vi "UNITEST MAIN v01.vi"() -> ()   [LabVIEW 2025]
uses:
  controls/LAB-IQ UI Data.ctl
  02c5850b-52e8-4ed5-91f8-6f0ad62f4994.vi
  support/Message Queue/Enqueue Message (Single).vi
  <vilib>/Utility/error.llb/Error Cluster From Error Code.vi
  <vilib>/ErrorRing/Error Ring.xnode
  support/Message Queue/LAB-IQ Message Queue.lvlib
  support/User Event - Stop/LAB-IQ User Event - Stop.lvlib
panel:
  in  "Stop Scratch":bool
  in  "Enter Fixed SRR 2":dbl min=0.0 max=0.0 format="%.3f"
  in  "E.Velocity 2":bool=TRUE caption="SRR"
  out "Message":string="Load Entered is out of range!!!"
  in  "Tab Control 3":T1(tab)
  in  "Tab Control 5":enum32{""}(tab)
  in  "Tab Control 14":T2(tab)=enum."Motor Load"
  in  "Ramp MulFac":dbl=2.0
  in  "pulses LoadDiffRamp(2..10)":dbl=9.0
  in  "PulseControlRamp(diff<=3N)":dbl=5.0 min=1.0 max=1000.0 step=1.0 format="%#.1f"
  in  "SetLoadDeadband(%) Load(0-10N)":dbl=0.1 min=0.0001 max=100.0 step=0.0001 format="%#.6f"
  in  "PID gains out delay (microForce)":T3={"proportional gain (Kc)"=300.0, "integral time (Ti, min)"=0.00011, "derivative time (Td, min)"=0.0} {"derivative time (Td, min)" format="%.3f"; "integral time (Ti, min)" min=1e-05 max=100.0 step=1e-06 format="%.6f"; "proportional gain (Kc)" format="%.3f"}
  in  "Ramp":bool
  in  "Gain 2":dbl=0.016
  in  "pulses LoadDiff(2..10)":dbl=10.0
  in  "pulses LoadDiff(11..50)":dbl=40.0
  in  "PulseControl(diff<=3N)":dbl=1.0 min=1.0 max=1000.0 step=1.0 format="%#.1f"
  out "SetLoadDeadband(%)  2":dbl=1.0 min=0.001 max=100.0 step=0.001 format="%#.6f"
  in  "Dummy Run":bool
  out "Vertical load (N)":dbl format="%#.3f"
  in  "AutoTune":bool
  in  "Offset  3":dbl=1.5
  in  "apply load":bool
  in  "Enter ByPass Load":dbl
  in  "reinit 3":bool=TRUE
  in  "output range delay":cluster{"output high":dbl, "output low":dbl}={"output high"=100.0, "output low"=-100.0} {"output low" format="%.2f"; "output high" format="%.2f"}
  in  "PID gains out delay":T3={"proportional gain (Kc)"=30.0, "integral time (Ti, min)"=0.00101, "derivative time (Td, min)"=0.0} {"derivative time (Td, min)" format="%.3f"; "integral time (Ti, min)" min=1e-05 max=100.0 step=0.0001 format="%.4f"; "proportional gain (Kc)" format="%.3f"}
  in  "Bypass Load":bool
  in  "pulsesSent":dbl=200.0
  out "pulses":dbl
  out "actpid":dbl
  out "gFF Rot 7":cluster{dbl, dbl, dbl}(graph)
  in  "pulses LoadDiff(21..1000)":dbl=40.0
  in  "Delay":dbl=1.5 min=0.001 max=5.0 step=0.001 format="%#.6f"
  in  "deadband":dbl=0.2
  in  "Tab Control 26":enum32{"Page 1", "Page 2"}(tab)
  in  "ClearAll":bool
  out "Mz(Nm)":dbl[](array[numeric])
  out "My(Nm)":dbl[](array[numeric])
  out "Mx(Nm)":dbl[](array[numeric])
  in  "Save Dwell":dbl=0.015 caption="Save Dwell (sec)" min=0.0 max=5.0 step=0.001 format="%.3f"
  out "Mx":dbl[](graph)
  out "My":dbl[](graph)
  out "Mz":dbl[](graph)
  out "Fx(N)":dbl[](graph)
  out "Fy(N)":dbl[](graph)
  out "Fz(N)":dbl[](graph)
  in  "ZeroAll":bool
  in  "Acq Delay (ms)":dbl=10.0
  in  "Burst Delay (ms)":dbl=10.0
  out "model":string
  out "SN":i32
  out "FFx(N)":dbl[](array[numeric])
  in  "Sensor IP":string="192.168.1.100"
  in  "Port":i32=8080
  out "FFy(N)":dbl[](array[numeric])
  out "Load(N)":dbl[](array[numeric])
  out "AE":bool
  in  "delete Handle":bool
  in  "Create Handle":bool=TRUE
  out "ft_data":dbl[](array[numeric])=[1.0, 1.0, 1.0, 1.0, 1.0, 1.0]
  out "ft_range":dbl[](array[numeric])=[1.0, 1.0, 1.0, 1.0, 1.0, 1.0]
  in  "stop 6":bool
  out "running_flag":bool
  out "ft_udp_handle":i32
  out "get-data-return":i32
  out "get-range-return":i32
  out "zero-return":i32
  out "filter-return":i32
  out "initial-return":i32
  out "deleteHandle-result":i32
  in  "Tab Control 19":enum32{"Platform COM", "Config ", "DevInfo"}(tab)=enum."Config "
  in  "SAMPLES":dbl=100.0
  in  "Re-initilaize":bool
  in  "Filter ON/OFF":bool=TRUE
  in  "TracHomeSurgeOffsetCounts 10MM":dbl=505100.0
  in  "TracHomeSwayOffsetCounts 10MM":dbl=1432.0
  in  "Acoustic Emission:":dbl=1.0 min=0.0001 max=200.0 step=0.0001 format="%.4f"
  in  "Apply Filter (FF)":bool
  in  "Filter% 2":dbl=50.0 min=50.0 max=100.0 step=0.1 format="%.1f"
  in  "Apply Filter (Load)":bool=TRUE
  in  "Filter%":dbl=80.0 min=50.0 max=100.0 step=0.1 format="%.1f"
  in  "Sway distance (mm)":dbl=245.0
  in  "Surge distance (mm)":dbl=370.0
  in  "DataSavingLoopDelay(ms)":dbl=15.0
  in  "SAVE  2":bool
  in  "Enter Distance":bool caption="Enter Counts"
  in  "Sway Counts:":dbl=100.0 min=0.0 max=100000000.0 step=1.0 format="%.2f"
  in  "Distance (mm): 3":dbl=100.0 caption="Distance (mm):" min=0.0 max=1500.0 step=0.001 format="%.5f"
  in  "Surge Counts:":dbl=100.0 min=0.0 max=100000000.0 step=1.0 format="%.1f"
  in  "Distance (mm): 2":dbl=100.0 caption="Distance (mm):" min=0.0 max=1500.0 step=0.0001 format="%.3f"
  in  "Distance (mm):":dbl=100.0 min=0.0 max=1500.0 step=0.001 format="%.5f"
  in  "Heave Counts:":dbl=100.0 min=0.0 max=100000000.0 step=1.0
  in  "LRMHomeSurgeOffsetCounts":dbl=307197.0
  in  "LRMHomeSwayOffsetCounts":dbl=26880.0
  in  "TracHomeSurgeOffsetCounts 20MM":dbl=505100.0
  in  "TracHomeSwayOffsetCounts 20MM":dbl=1432.0
  in  "RotHomeSwayOffsetCounts":dbl=14656.0
  in  "RotHomeSurgeOffsetCounts":dbl=311465.0
  in  "Heave distance":dbl=340.0
  out "Zmm":dbl=1600.0
  out "Heave Pulses/mm":dbl=1600.0
  out "Surge Pulses/mm":dbl=1600.0
  out "Sway Pulses/mm":dbl=320.0
  in  "Heave Pitch":dbl=4.0
  in  "Surge Pitch":dbl=3.0
  in  "Sway Pitch":dbl=2.0
  in  "Heave PPR":dbl=6400.0
  in  "Surge PPR":dbl=6400.0
  in  "Sway PPR":dbl=6400.0
  in  "GUI":T4(tab)
  in  "Platform Settings":bool caption="Password"
  in  "Configure":bool caption="Password"
  in  "Home":bool caption="Password"
  in  "EXIT":bool
  in  "Analysis":bool caption="Password"
  in  "service 2":bool caption="Password"
  in  "MainPage":T5(tab)=enum."HOME"
  in  "Select Load Head":bool
  in  "Notes :":string
  in  "FILE":string
  in  "Sample ID :":string
  in  "Operator ID :":string
  in  "Operator Name :":string
  in  "Auto":bool caption="Power Status"
  out "mm/s  Surge":dbl=7.0 caption="Jog" min=0.001 max=50.0 step=0.0001 format="%.2f"
  in  "Update Surge Speed":bool
  out "Drive Error":string
  in  "Disable Axis Jog Soft Limits":bool
  out "mm/s  Sway":dbl=7.0 caption="Jog" min=0.001 max=50.0 step=0.0001 format="%.2f"
  out "Sway and Surge COM Status":bool=TRUE caption="Load COM Status"
  out "Heave COM Status":bool=TRUE caption="Load COM Status"
  in  "Enable Platform":bool
  in  "Surge Forward Main":bool
  in  "Surge Backward Main":bool
  in  "Sway Right Main":bool
  in  "Sway Left Main":bool
  in  "Heave Down Main":bool
  in  "Heave Up main":bool
  in  "Update Sway Speed":bool
  in  "Update Heave Speed":bool
  out "mm/s Heave":dbl=7.0 caption="Jog" min=0.001 max=30.0 step=0.0001 format="%.2f"
  in  "mm/sec":dbl=1.0 caption="Jog" min=0.001 max=50.0 step=0.001 format="%.2f"
  in  "mm":dbl=0.001 caption="Jog" min=0.001 max=200.0 step=0.0001 format="%#.3f"
  in  "Surface Analysis":bool
  in  "Imaging":bool
  in  "Image Analysis":bool
  in  "Post Analysis":bool
  in  "SSP 0.75":bool
  in  "SSP 0.5":bool
  in  "SSP 0.3":bool
  in  "Warning":enum32{"Page 2"}(tab)
  in  "gui GIF":enum32{"Check", "Deca", "kilo", "Micro"}(tab)
  out "Communication is established":bool=TRUE caption="Load COM Status"
  in  "Reference Sample":u16(ring) items=["None", "Brass", "Aluminium", "Mild Steel"]
  out "Load Cell Communication Slide":u8(slide)=1 min=1 max=10 step=1 scale=0.0..10.0
  in  "com 3":bool
  out "com":bool
  out "DecaForce COM Status":bool caption="Load COM Status"
  in  "Loading Mode":u16(ring) items=["Constant", "Ramp", "Steps", "Indentation"]
  in  "Enter the CoF Trip":dbl=1.0
  in  "Enter the Friction Force Trip":dbl=520.0 min=500.0 max=500.0 step=1.0 format="%#.1f"
  in  "Enter the Normal load Trip":dbl=520.0 min=500.0 max=500.0 step=0.001 format="%.3f"
  in  "KiloForce":bool
  in  "DecaForce":bool
  in  "MicroForce":bool
  in  "LHBack":bool
  in  "LHNext":bool
  in  "Load Selection":T6(tab)
  in  "Enter the Load  (N)":dbl=2.0 min=2.0 max=50.0 step=0.1 format="%#.4f"
  in  "Enter the Final Load (N)":dbl=1.0 min=0.0 max=500.0 step=1.0 format="%#.0f"
  in  "Update":bool
  in  "Enter the Loading Rate (N/min)":dbl=60.0 min=60.0 max=1200.0 step=0.1 format="%.2f"
  out "Warning 2":bool
  in  "Stribeck Table  For loading":string[][](table)=[["", "", ""], ["", "", ""], ["", "", ""], ["", "", ""]]
  in  "Stribeck table":bool
  in  "seq":bool=TRUE
  in  "Clear 3":bool
  in  "Indentation":string[][](table)=[["Detection", "5", "2"], ["Unload", "0", "5"], ["Load", "10", "2"], ["Unload", "0", "5"], ["Detection", "5", "2"], ["Unload", "0", "5"]]
  in  "Multipoint":bool caption="Singlepoint"
  in  "AppLoad 4":bool
  in  "zNL":bool
  out "NL disp":dbl caption="Normal Load ( N )" min=-2000.0 max=2000.0 step=0.0001 format="%.1f"
  in  "Traction":bool
  in  "Surge Forward MM":bool
  in  "Surge Backward MM":bool
  in  "M3 Image":enum32{"Page 1", "Page 2"}(tab)
  in  "String 39":string="Jog heave to bring the upper sample closer to the lower sample within 1mm."
  in  "Sway Left MM":bool
  in  "Sway Right MM":bool
  in  "Disable Axis Jog Soft Limits":bool
  in  "mm":dbl=0.001 caption="Jog" min=0.001 max=5.0 step=0.0001 format="%#.3f"
  in  "Heave Down MM":bool
  in  "Heave Up MM":bool
  in  "Wear Track Diameter (mm)":dbl=5.0 caption="Wear Track Diameter (mm):" min=1.0 max=30.0 step=1.0 format="%.2f"
  in  "Set WTD":bool
  in  "HomeScratch":bool
  in  "HomeRot":bool
  in  "PlaceModule":bool
  in  "Motion Mode:":u16(ring) items=["Uniform Rotation", "Angular Oscillation", "Stribeck ", "Steps"]
  in  "LR Sway":bool
  in  "Rot Hor":bool
  in  "Rot Ver":bool
  in  "Scratch":bool
  in  "LR Cam":bool
  in  "MMBack":bool
  in  "MMNext":bool
  in  "Rotary Module Selection":T7(tab)
  in  "SPEED SELECTION :":enum32{"Speed in RPM", "Speed in m/sec"}(radio)=enum."Speed in m/sec"
  in  "TEST SELECTION":enum32{"Time", "Cycle"}(radio)
  in  "Enter the Speed(mm/sec)":dbl=1.0 min=0.1 max=10.0 step=0.1 format="%.1f"
  in  "Enter the Speed(RPM)":dbl=45.0 min=5.0 max=300.0 step=1.0
  in  "Enter the Frequency (Hz)":dbl=1.0 min=0.1 max=10.0 step=0.1 format="%.1f"
  in  "Enter the Angle (Deg)":dbl=45.0 min=5.0 max=300.0 step=1.0
  in  "Angular Oscillation Set":bool
  in  "Rotary Tab":enum32{"Page 1", "Page 2"}(tab)
  out "e.v/ssr 2":enum32{"E.V", "SSR"}(tab)
  in  "Enter the Final E.Velocity (m/s) 2":dbl=1.0 min=0.001 max=4.0 step=0.001 format="%.3f"
  in  "Enter initial E.Velocity (m/s) 2":dbl=2.0 min=0.001 max=4.0 step=0.001 format="%.3f"
  in  "Enter Fixed E.Velocity 2":dbl=1.0 min=0.001 max=2.0 step=0.001 format="%.3f"
  in  "Enter Final SRR 2":dbl=1.0 min=0.001 max=1.0 step=0.001 format="%.2f"
  in  "Enter initial SRR 2":dbl=1.0 min=0.001 max=1.0 step=0.001 format="%.2f"
  out "Final Speed (RPM) 3":dbl=1.0 min=0.1 max=3000.0 step=0.1 format="%.1f"
  out "Initial Speed (RPM) 2":dbl=100.0 min=0.1 max=3000.0 step=0.1 format="%.1f"
  in  "Enter the Final Velocity (m/s) 3":dbl=1.0 min=0.001 max=2.0 step=0.001 format="%.3f"
  in  "Enter initial Velocity (m/s)  3":dbl=2.0 min=0.001 max=2.0 step=0.001 format="%.3f"
  out "Ramp Up 2":bool caption="Ramp Down"
  in  "File Path :  2":path
  in  "Import 2":bool
  in  "Save 2":bool
  in  "SPEED SELECTION : rotary":enum32{"Speed in Rpm", "Speed in m/sec"}(radio)=enum."Speed in m/sec"
  in  "calculate rotary":bool
  in  "String 45":string="File Path Location : C:-->LAB-IQ 150 --> User Defined\n                                       Protocol-->File.txt"
  in  "Step Speed":enum32{"Step Speed", "Step (load-Speed)"}(tab)
  in  "StepTable For Speed":string[][](table)=[["", "", ""], ["", "", ""], ["", "", ""], ["", "", ""]]
  in  "StepTable For Load-Speed":string[][](table)=[["", "", ""], ["", "", ""], ["", "", ""], ["", "", ""]]
  in  "StepTable For Speed 3":string[][](table)=[["", "", ""], ["", "", ""], ["", "", ""], ["", "", ""]]
  in  "Motion Direction:  3":u16(ring) items=["Clockwise", "Counter Clockwise"]
  out "Humidity  Status  3":bool caption="Communication Status"
  out "Low Temp  Status  2":bool caption="Communication Status"
  out "TK4 status 2":bool caption="Communication Status"
  in  "String 40":string="Before selecting Acoustic make sure the sensor output pin is connected to A4."
  in  "Stage Temperature":dbl[](array[numeric])=[150.0, 230.0, 300.0, 350.0, 400.0, 450.0, 500.0]
  in  "Sample Temperature":dbl[](array[numeric])=[100.0, 150.0, 200.0, 250.0, 300.0, 350.0, 400.0]
  in  "Humidity (Amb)":bool
  in  "Clear List":bool
  out "Sensors Picked":string
  in  "Add to list":bool
  in  "Wear":bool
  in  "Vibration":bool
  in  "Humidity (Chamber)":bool
  in  "Temperature (Chamber)":bool
  in  "ECR":bool
  in  "Temperature (Amb)":bool
  in  "Microphone":bool
  in  "Acoustic Emission 3":bool
  in  "SNext":bool
  in  "APBack":bool
  in  "Enter the Temperature (°C):":dbl
  in  "Enter the Stage \nTemperature (°C):":dbl=20.0 min=20.0 max=150.0 step=1.0 format="%#.0f"
  in  "Enter the Humidity (%Rh):":dbl=30.0 min=30.0 max=85.0 step=1.0
  in  "Low Temp":bool
  in  "High Temp":bool
  in  "Humidity":bool
  in  "Main Screen Tab":T8(tab)
  in  "AppLoadSeq scratch":bool
  in  "ClrLog":bool
  out "Trip Log":string
  in  "STOP":bool
  in  "Start Test":bool
  out "Test status":bool caption="Test Status"
  out "AR Led":bool caption="AR"
  out "Data":bool=TRUE
  out "Health":bool=TRUE
  out "Sway COM Status":bool=TRUE caption="Load COM Status"
  out "Heave COM Status":bool=TRUE caption="Load COM Status"
  in  "Grp Tab":enum32{"Rot/LRM", "FBT"}(tab)
  in  "Sub Graph":T9(tab)
  in  "Speed Reset Graph":bool
  in  "Speed Tab":enum32{" Rotary Disc", "MTM Ball", "MTM Disc"}(tab)
  out "speed mm/sec":dbl(graph)=0.13298760003255525
  out "MTM BALL SPEED":dbl(graph)=0.13298760003255525
  out "MTM DISC  SPEED":dbl(graph)=0.13298760003255525
  in  "Temperature Reset":bool
  out "Temperature (deg c)":dbl(graph)=0.13298760003255525
  in  "ECR RESET":bool
  out "ECR":dbl(graph)=0.13298760003255525
  out "Acoustic Emission (mV)":dbl min=0.0 max=5000.0 step=0.1
  in  "Aqucostic Reset Graph":bool
  out "gACQUOS":dbl(graph)=0.13298760003255525
  in  "Humidity Reset Graph":bool
  out "HumrGp":dbl(graph)=0.13298760003255525
  out "SD (mm)":dbl caption="Sliding Distance ( mm )" min=-200.0 max=200.0 step=0.1 format="%.4f"
  in  "Siliding distance Reset Graph":bool
  out "SDGp":dbl(graph)=0.13298760003255525
  out "Hymidity":bool
  in  "Humidity Disable trip":bool=TRUE
  in  "CoF Trip  2":dbl=540.0 min=100.0 max=540.0 step=1.0
  out "Depth Trip":dbl=600.0
  in  "Depth Trip":bool=TRUE
  out "Weart Deapth":bool
  in  "Depth Reset Graph":bool
  out "Weart":bool
  in  "Depthz":bool
  out "Depth (µm)":dbl min=-200.0 max=200.0 step=0.1 format="%.1f"
  out "WearGp":dbl(graph)=0.13298760003255525
  out "NL Trip 2":dbl=600.0
  out "Load pid":bool
  in  "Load Disable Trip":bool=TRUE
  in  "Load Reset Graph":bool
  out "NL Display 4":dbl caption="Normal Load ( N )" min=-2000.0 max=2000.0 step=0.0001 format="%.1f"
  out "Main Chart 3":cluster{dbl, "NL disp":dbl, dbl}(graph)
  in  "FF Tab":T10(tab)
  in  "COF Reset Graph":bool
  in  "COF Disable Trip":bool=TRUE
  out "COF TRIP":dbl=600.0
  out "COF MAIN CHART":cluster{dbl, "NL disp":dbl, dbl}(graph)
  out "Friction Force (N)":dbl min=-2000.0 max=2000.0 step=0.0001 format="%.1f"
  in  "FF Reset Graph":bool
  in  "FF Disable Trip":bool=TRUE
  out "FF TRIP":dbl=600.0
  out "FF MAIN CHART":cluster{dbl, "NL disp":dbl, dbl}(graph)
  in  "BACK":bool
  out "Ambient \nTemperature":dbl min=0.0 max=5000.0 step=0.1 format="%.1f"
  out "Ambient\n Humidity":dbl min=0.0 max=5000.0 step=0.1 format="%.2f"
  out "NL disp 2":dbl caption="Normal Load ( N )" min=-2000.0 max=2000.0 step=0.0001 format="%.1f"
  out "Set Humidity":dbl caption="Set Humidity  (% Rh)" min=-2000.0 max=2000.0 step=1.0 format="%.1f"
  out "humidity disp":dbl caption="Humidity (% Rh)" min=-2000.0 max=2000.0 step=1.0 format="%.1f"
  in  "Humidity On":bool
  in  "zNL 2":bool
  out "NLt":bool
  in  "Load En":bool
  out "Freq (Hz)":dbl min=0.0 max=5000.0 step=0.1 format="%.4f"
  out "HumCOMStatus":bool caption="Communication Status"
  out "Load Communication":bool
  in  "Temp Tabs":enum32{"Low Temp", "High Temp"}(tab)
  out "Controller  Status":bool
  out "ChamberTemp":dbl format="%#.1f"
  in  "SetTmp":dbl=-190.0 caption="Set Temperature (Deg C)" min=-190.0 max=100.0 step=1.0 format="%.1f"
  in  "Cooling":bool
  in  "Heater":bool
  out "TK4 status":bool caption="Controller  Status"
  out "ChamberTemp":dbl format="%#.1f"
  in  "SetTmp":dbl caption="Set Temperature (Deg C)" min=0.0 max=1000.0 step=1.0 format="%.1f"
  in  "Set Load (N)":dbl=100.0 min=0.01 max=1500.0 step=0.01 format="%.1f"
  in  "Time Tab":enum32{"cycles", "duration"}(tab)
  out "Test Duration 4":dbl=600.0 caption="Test Duration\n(HH:MM:SS)" min=0.0083 max=180000.0 step=0.0001 format="%<%H:%M:%S>t"
  out "TEST CYCLE":dbl min=0.0 max=5000.0 step=0.01 format="%.2f"
  in  "TOTAL CYCLES":dbl min=0.0 max=5000.0 step=0.1 format="%.4f"
  out "Time ( HH:MM:SS ) 2":dbl min=0.0 max=144000.0 step=1.0 format="%<%H:%M:%S>t"
  in  "Test Duration":dbl=600.0 caption="Test Duration\n(HH:MM:SS)" min=0.0083 max=180000.0 step=0.0001 format="%<%H:%M:%S>t"
  in  "Main Speed Tab":enum32{"ROTARY", "TRACTION"}(tab)
  in  "SPEED TAB":enum32{"RPM", "m/sec"}(tab)
  out "Speed (RPM)":dbl min=0.0 max=5000.0 step=0.1 format="%.1f"
  out "Set Speed":dbl caption="Set Speed (RPM)" min=0.0 max=1500.0 step=0.1 format="%.1f"
  out "Speed (m/sec)":dbl min=0.0 max=5000.0 step=0.001 format="%.4f"
  out "Set Speed (m/sec)":dbl min=0.0 max=1500.0 step=0.001 format="%.4f"
  in  "MTM MOTOR DISPLAY":enum32{"MTM RPM", "MTM m/sec"}(tab)
  out "Disc Speed (RPM)":dbl min=0.0 max=1500.0 step=0.1 format="%.1f"
  out "Ball Speed (RPM)":dbl min=0.0 max=1500.0 step=0.1 format="%.1f"
  out "Disc Speed (m/sec)":dbl min=0.0 max=1500.0 step=0.1 format="%.1f"
  out "Ball Speed (m/sec)":dbl min=0.0 max=1500.0 step=0.1 format="%.1f"
  in  "Angle and Frequency":enum32{"angular", "lrm"}(tab)
  out "Angle (Deg)":dbl min=0.0 max=5000.0 step=0.01 format="%.2f"
  out "Stroke (mm)":dbl min=0.0 max=5000.0 step=0.01 format="%.2f"
  in  "Analysis Home":bool
  in  "Password":string
  in  "Home Service":bool
  in  "Advanced Setting":bool
  in  "About Tab":enum32{"Primary"}(tab)
  in  "ECR Port:":refnum<visa-resource-name>="COM10"
  in  "Ramp Port:":refnum<visa-resource-name>="COM10"
  in  "Installation/Replacement completed":bool
  in  "Loahead":bool
  in  "Heave and Surge COM Port:":refnum<visa-resource-name>="COM9"
  in  "Sway COM Port:":refnum<visa-resource-name>="COM10"
  in  "Temp Modbus:":refnum<visa-resource-name>="COM14"
  in  "Humidity Port:":refnum<visa-resource-name>="COM10"
  in  "Edit Gain Constants":bool
  in  "Save Gain Constants":bool
  in  "Service About":bool
  # "load Aquisition off"
  # "load Aquisition On"
  # "Configuration"
  # "Limits for Heave Surge and Sway"
  # "Modules Offset Parameters"
  # "Counts-Distance Calculator"
  # "File Name :"
  # "Ensure the traction module is aligned\n horizontally with the stage before ENABLE."
  # "SET JOG SPEED"
  # "JOG MODE"
  # "Module Selection"
  # "Positioning Control"
  # "Connect the controller\ncable to M3"
  # "Environment"
  # "Sensors"
  # "Data Points"
  # "Data Points"
  # "Data Points"
  # "Data Points"
  # "ohms"
  # "Data Points"
  # "Data Points"
  # "Data Points"
  # "LAB-IQ 150 / UNITEST / WO2456 / UT150  v05 / AUGUST 2025"
  # "NOTE: This operation needs to be done only when the machine is ON."
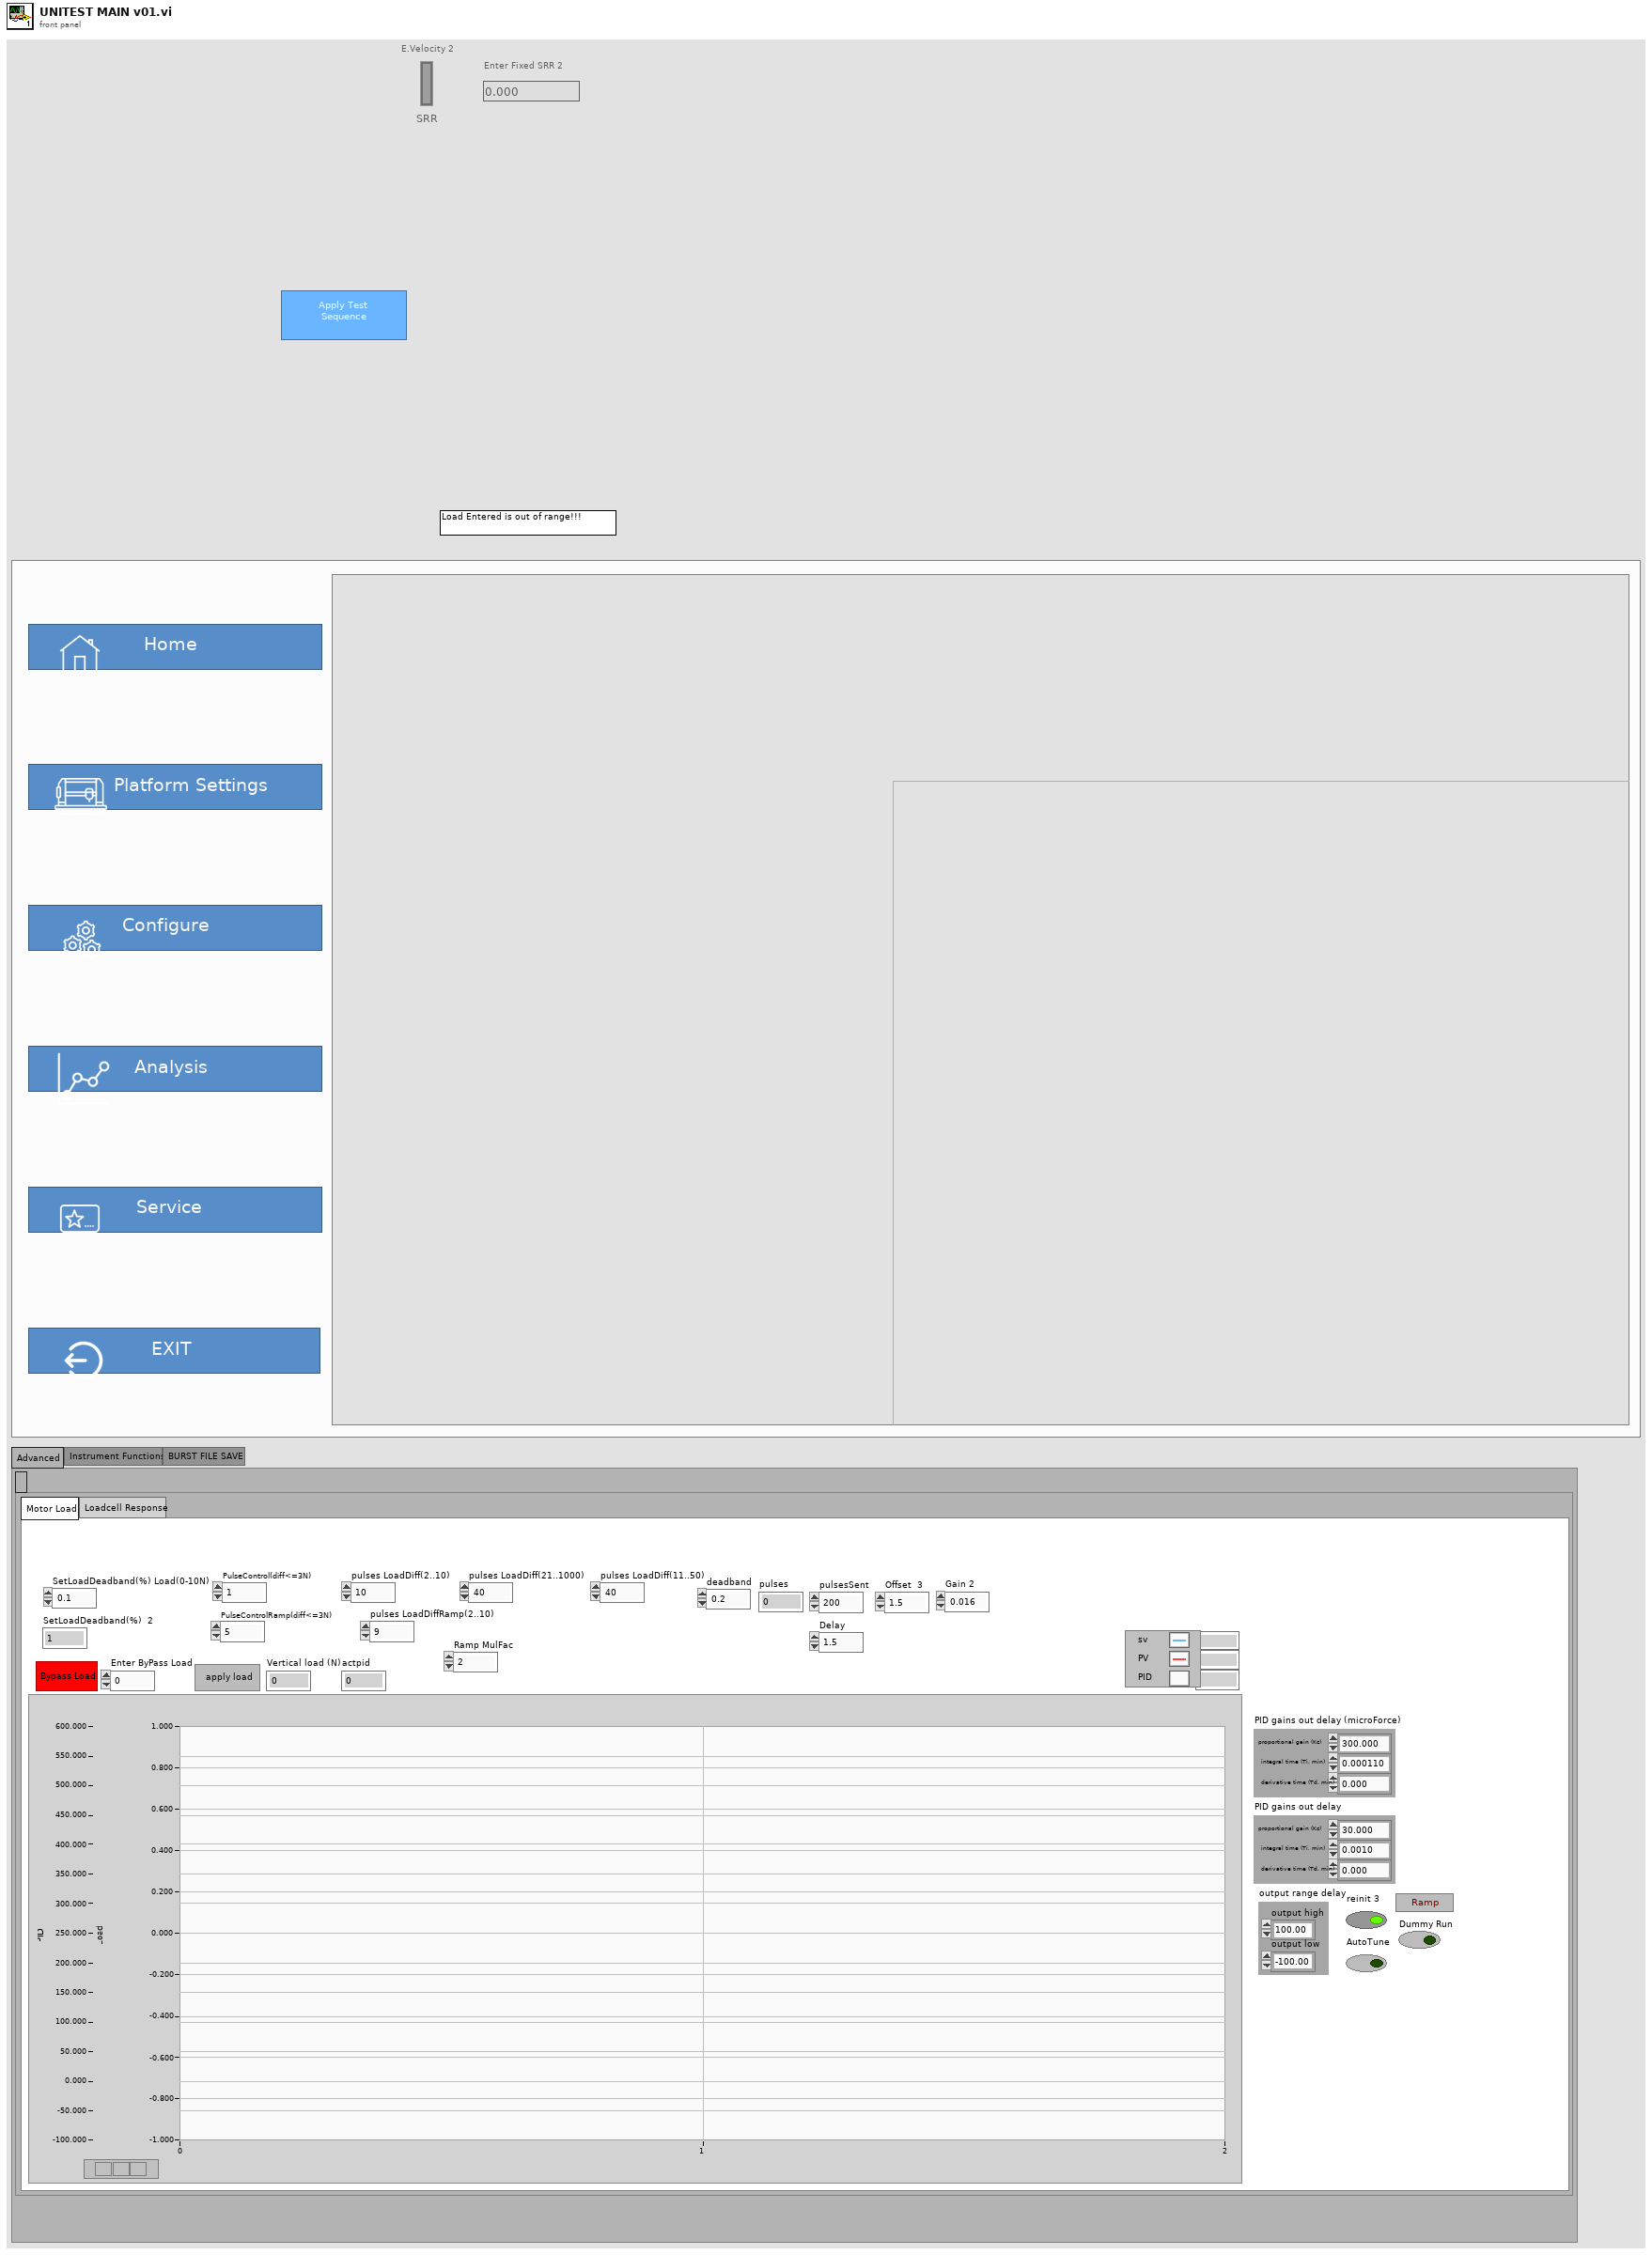
[diagram p1: front panel]
types:
  T1 = enum32{"Advanced", "Motor", "Depth_graph", "UIO Communicator", "Add to list parametrs", "Instrument Functions", "BURST FILE SAVE"}
  T2 = enum32{"LRM heating", "FBT_Heating", "Motor Load", "Loadcell Response", "Voice Load", "Step loading and speed ", "Depth"}
  T3 = cluster{"proportional gain (Kc)":dbl, "integral time (Ti, min)":dbl, "derivative time (Td, min)":dbl}
  T4 = enum32{"Setup", "Load Head", "Motion Module", "Environment", "Begin"}
  T5 = enum32{"Details", "PlatformSetting", "Analysis", "HOME"}
  T6 = enum32{"Constant", "Ramp", "Step", "Indentation"}
  T7 = enum32{"Uniform Rotation", "Angular Oscillation", "Speed Ramp", "Speed Step"}
  T8 = enum32{"  Acquire  ", "Compare Files Rot", "About", "Service"}
  T9 = enum32{"Speed", "Temperature", "ECR", "Acoustic Emission", "Humidity", "Sliding Distance"}
  T10 = enum32{"Coefficient of Friction ", "Friction Force (N)"}
  T11 = typedef "LAB-IQ UI Data.ctl" = cluster{"Main Home Screen":cluster{"GUI":refnum<vi>, "Platform Settings":refnum<vi>, "Configure":refnum<vi>, "Home":refnum<vi>, "EXIT":refnum<vi>, "service 2":refnum<vi>, "MainPage":refnum<vi>, "Analysis":refnum<vi>}, "Platform Settings":cluster{"mm/s  Surge":refnum<vi>, "Update Surge Speed":refnum<vi>, "Drive Error":refnum<vi>, "Disable Axis Jog Soft Limits":refnum<vi>, "mm/s  Sway":refnum<vi>, "Sway and Surge COM Status":refnum<vi>, "Heave COM Status":refnum<vi>, "Enable Platform":refnum<vi>, "Surge Forward Main":refnum<vi>, "Sway Right Main":refnum<vi>, "Sway Left Main":refnum<vi>, "Heave Down Main":refnum<vi>, "Heave Up main":refnum<vi>, "Update Sway Speed":refnum<vi>, "Update Heave Speed":refnum<vi>, "mm/s Heave":refnum<vi>, "mm/sec":refnum<vi>, "mm":refnum<vi>, "Surge Backward Main":refnum<vi>}, "Analysis Screen":cluster{"Analysis Home":refnum<vi>, "Surface Analysis":refnum<vi>, "Imaging":refnum<vi>, "Image Analysis":refnum<vi>, "Post Analysis":refnum<vi>}, "Config Screen":cluster{"Select Load Head":refnum<vi>, "Notes :":refnum<vi>, "FILE":refnum<vi>, "Sample ID :":refnum<vi>, "Operator ID :":refnum<vi>, "Operator Name :":refnum<vi>, "Auto":refnum<vi>}, "Motion Module":cluster{"zNL":refnum<vi>, "NL disp":refnum<vi>, "Rotary Tab":refnum<vi>, "Motion Direction:  3":refnum<vi>, "E.Velocity 2":refnum<vi>, "e.v/ssr 2":refnum<vi>, "Enter Fixed E.Velocity 2":refnum<vi>, "Enter Final SRR 2":refnum<vi>, "Enter initial SRR 2":refnum<vi>, "Enter Fixed SRR 2":refnum<vi>, "Enter the Final E.Velocity (m/s) 2":refnum<vi>, "Enter initial E.Velocity (m/s) 2":refnum<vi>, "Final Speed (RPM) 3":refnum<vi>, "Initial Speed (RPM) 2":refnum<vi>, "Enter the Final Velocity (m/s) 3":refnum<vi>, "Enter initial Velocity (m/s)  3":refnum<vi>, "Ramp Up 2":refnum<vi>, "TEST SELECTION":refnum<vi>, "SPEED SELECTION : ":refnum<vi>, "Angular Oscillation Set":refnum<vi>, "Traction":refnum<vi>, "Step Speed":refnum<vi>, "StepTable For Load-Speed":refnum<vi>, "StepTable For Speed":refnum<vi>, "Surge Forward MM":refnum<vi>, "Surge Backward MM":refnum<vi>, "M3 Image":refnum<vi>, "String 39":refnum<vi>, "Sway Left MM":refnum<vi>, "Sway Right MM":refnum<vi>, "Disable Axis Jog Soft Limits":refnum<vi>, "mm":refnum<vi>, "Heave Down MM":refnum<vi>, "Heave Up MM":refnum<vi>, "Wear Track Diameter (mm)":refnum<vi>, "Set WTD":refnum<vi>, "HomeScratch":refnum<vi>, "HomeRot":refnum<vi>, "PlaceModule":refnum<vi>, "Enter the Angle (Deg)":refnum<vi>, "Enter the Frequency (Hz)":refnum<vi>, "Motion Mode:":refnum<vi>, "LR Sway":refnum<vi>, "Rot Hor":refnum<vi>, "Scratch":refnum<vi>, "LR Cam":refnum<vi>, "MMBack":refnum<vi>, "MMNext":refnum<vi>, "Rot Ver":refnum<vi>, "Rotary Module Selection":refnum<vi>, "calculate rotary":refnum<vi>, "SPEED SELECTION : rotary":refnum<vi>, "Import 2":refnum<vi>, "Save 2":refnum<vi>, "File Path :  2":refnum<vi>, "String 45":refnum<vi>, "StepTable For Speed 3":refnum<vi>, "Enter the Speed(mm/sec)":refnum<vi>, "Enter the Speed(RPM)":refnum<vi>}, "Environmental control":cluster{"Humidity  Status  3":refnum<vi>, "Low Temp  Status  2":refnum<vi>, "TK4 status 2":refnum<vi>, "Stage Temperature":refnum<vi>, "Sample Temperature":refnum<vi>, "Humidity (Amb)":refnum<vi>, "Clear List":refnum<vi>, "Add to list":refnum<vi>, "Wear":refnum<vi>, "Vibration":refnum<vi>, "Humidity (Chamber)":refnum<vi>, "Temperature (Chamber)":refnum<vi>, "ECR ":refnum<vi>, "Temperature (Amb)":refnum<vi>, "Microphone":refnum<vi>, "Acoustic Emission 3":refnum<vi>, "SNext":refnum<vi>, "APBack":refnum<vi>, "Enter the Temperature (°C):":refnum<vi>, "Enter the Stage \nTemperature (°C):":refnum<vi>, "Enter the Humidity (%Rh):":refnum<vi>, "Low Temp":refnum<vi>, "High Temp":refnum<vi>, "Humidity":refnum<vi>, "Sensors Picked":refnum<vi>}, "About Screen":cluster{"Password":refnum<vi>, "Home Service":refnum<vi>, "Advanced Setting":refnum<vi>, "About Tab":refnum<vi>, "ECR Port:":refnum<vi>, "Ramp Port:":refnum<vi>, "Installation/Replacement completed":refnum<vi>, "Loahead":refnum<vi>, "Heave and Surge COM Port:":refnum<vi>, "Sway COM Port:":refnum<vi>, "Temp Modbus:":refnum<vi>, "Humidity Port:":refnum<vi>, "Edit Gain Constants":refnum<vi>, "Save Gain Constants":refnum<vi>}, "Main Screen":cluster{"Main Screen Tab":refnum<vi>, "Angle and Frequency":refnum<vi>, "Stroke (mm)":refnum<vi>, "Angle (Deg)":refnum<vi>, "Main Speed Tab":refnum<vi>, "MTM MOTOR DISPLAY":refnum<vi>, "Disc Speed (m/sec)":refnum<vi>, "Ball Speed (m/sec)":refnum<vi>, "Disc Speed (RPM)":refnum<vi>, "Ball Speed (RPM)":refnum<vi>, "SPEED TAB":refnum<vi>, "Speed (m/sec)":refnum<vi>, "Set Speed (m/sec)":refnum<vi>, "Speed (RPM)":refnum<vi>, "Set Speed":refnum<vi>, "Time Tab":refnum<vi>, "Time ( HH:MM:SS ) 2":refnum<vi>, "Test Duration":refnum<vi>, "Test Duration 4":refnum<vi>, "TEST CYCLE":refnum<vi>, "TOTAL CYCLES":refnum<vi>, "Set Load (N)":refnum<vi>, "Temp Tabs":refnum<vi>, "Heater":refnum<vi>, "TK4 status":refnum<vi>, "ChamberTemp":refnum<vi>, "SetTmp":refnum<vi>, "Controller  Status":refnum<vi>, "ChamberTemp 2":refnum<vi>, "SetTmp 2":refnum<vi>, "Controller  Status 2":refnum<vi>, "ChamberTemp 3":refnum<vi>, "SetTmp 3":refnum<vi>, "Cooling":refnum<vi>, "Load Communication":refnum<vi>, "Ambient \nTemperature":refnum<vi>, "HumCOMStatus":refnum<vi>, "Ambient\n Humidity":refnum<vi>, "Freq (Hz)":refnum<vi>, "Load En":refnum<vi>, "NLt":refnum<vi>, "zNL 2":refnum<vi>, "Humidity On":refnum<vi>, "humidity disp":refnum<vi>, "Set Humidity":refnum<vi>, "NL disp 2":refnum<vi>, "Humidity On 2":refnum<vi>, "humidity disp 2":refnum<vi>, "Set Humidity 2":refnum<vi>, "NL disp 3":refnum<vi>, "AppLoadSeq scratch":refnum<vi>, "Stop Scratch":refnum<vi>, "ClrLog":refnum<vi>, "Trip Log":refnum<vi>, "STOP":refnum<vi>, "Start Test":refnum<vi>, "Test status":refnum<vi>, "AR Led":refnum<vi>, "Data":refnum<vi>, "Health":refnum<vi>, "Sway COM Status":refnum<vi>, "Heave COM Status":refnum<vi>, "Grp Tab":refnum<vi>, "Sub Graph":refnum<vi>, "SD (mm)":refnum<vi>, "Siliding distance Reset Graph":refnum<vi>, "SDGp":refnum<vi>, "Humidity Reset Graph":refnum<vi>, "HumrGp":refnum<vi>, "Acoustic Emission (mV)":refnum<vi>, "Aqucostic Reset Graph":refnum<vi>, "gACQUOS":refnum<vi>, "ECR RESET":refnum<vi>, "ECR":refnum<vi>, "Temperature Reset":refnum<vi>, "Acoustic Emission (mV) 2":refnum<vi>, "Aqucostic Reset Graph 2":refnum<vi>, "gACQUOS 2":refnum<vi>, "ECR RESET 2":refnum<vi>, "ECR 2":refnum<vi>, "Temperature Reset 2":refnum<vi>, "Temperature (deg c)":refnum<vi>, "Speed Reset Graph":refnum<vi>, "Speed Tab":refnum<vi>, "MTM DISC  SPEED":refnum<vi>, "MTM BALL SPEED":refnum<vi>, "speed mm/sec":refnum<vi>, "Hymidity":refnum<vi>, "Humidity Disable trip":refnum<vi>, "CoF Trip  2":refnum<vi>, "Depth Trip":refnum<vi>, "Weart Deapth":refnum<vi>, "Depth Reset Graph":refnum<vi>, "Weart":refnum<vi>, "Depthz":refnum<vi>, "Depth (µm)":refnum<vi>, "WearGp":refnum<vi>, "NL Trip 2":refnum<vi>, "Load pid":refnum<vi>, "Load Disable Trip":refnum<vi>, "Load Reset Graph":refnum<vi>, "NL Display 4":refnum<vi>, "Main Chart 3":refnum<vi>, "BACK":refnum<vi>, "Depth Trip 2":refnum<vi>}, "Loading":cluster{"Indentation":refnum<vi>, "Reference Sample":refnum<vi>, "Load Cell Communication Slide":refnum<vi>, "com 3":refnum<vi>, "com":refnum<vi>, "DecaForce COM Status":refnum<vi>, "Update":refnum<vi>, "Clear 3":refnum<vi>, "seq":refnum<vi>, "Stribeck table":refnum<vi>, "Stribeck Table  For loading":refnum<vi>, "Loading Mode":refnum<vi>, "Enter the Final Load (N)":refnum<vi>, "Enter the CoF Trip":refnum<vi>, "Enter the Friction Force Trip":refnum<vi>, "Enter the Normal load Trip":refnum<vi>, "Enter the Load  (N)":refnum<vi>, "KiloForce":refnum<vi>, "DecaForce ":refnum<vi>, "MicroForce":refnum<vi>, "LHBack":refnum<vi>, "LHNext":refnum<vi>, "Enter the Loading Rate (N/min)":refnum<vi>, "Message":refnum<vi>, "Warning 2":refnum<vi>, "SSP 0.75":refnum<vi>, "SSP 0.5":refnum<vi>, "SSP 0.3":refnum<vi>, "Warning":refnum<vi>, "gui GIF":refnum<vi>, "Communication is established":refnum<vi>, "AppLoad 4":refnum<vi>, "Multipoint":refnum<vi>, "Load Selection":refnum<vi>}, "PID":cluster{"Ramp MulFac":refnum<vi>, "pulses LoadDiffRamp(2..10)":refnum<vi>, "PulseControlRamp(diff<=3N)":refnum<vi>, "SetLoadDeadband(%) Load(0-10N)":refnum<vi>, "PID gains out delay (microForce)":refnum<vi>, "Ramp":refnum<vi>, "Gain 2":refnum<vi>, "pulses LoadDiff(2..10)":refnum<vi>, "pulses LoadDiff(11..50)":refnum<vi>, "PulseControl(diff<=3N)":refnum<vi>, "SetLoadDeadband(%)  2":refnum<vi>, "Dummy Run":refnum<vi>, "Vertical load (N)":refnum<vi>, "AutoTune":refnum<vi>, "Offset 3 ":refnum<vi>, "apply load":refnum<vi>, "Offset  3":refnum<vi>, "apply load 2":refnum<vi>, "Enter ByPass Load":refnum<vi>, "reinit 3":refnum<vi>, "output range delay":refnum<vi>, "PID gains out delay":refnum<vi>, "Bypass Load":refnum<vi>, "pulsesSent":refnum<vi>, "pulses ":refnum<vi>, "actpid":refnum<vi>, "gFF Rot":refnum<vi>, "pulses LoadDiff(21..1000)":refnum<vi>, "Delay":refnum<vi>, "deadband":refnum<vi>}, "Config Parameters":cluster{"Tab Control 3":refnum<vi>, "Tab Control 19":refnum<vi>, "SAMPLES":refnum<vi>, "Re-initilaize":refnum<vi>, "Filter ON/OFF":refnum<vi>, "TracHomeSurgeOffsetCounts 10MM":refnum<vi>, "TracHomeSwayOffsetCounts 10MM":refnum<vi>, "Acoustic Emission:":refnum<vi>, "Apply Filter (FF)":refnum<vi>, "Filter% 2":refnum<vi>, "Apply Filter (Load)":refnum<vi>, "Filter% ":refnum<vi>, "Sway distance (mm)":refnum<vi>, "Surge distance (mm)":refnum<vi>, "DataSavingLoopDelay(ms)":refnum<vi>, "SAVE 2":refnum<vi>, "Enter Distance":refnum<vi>, "Sway Counts:":refnum<vi>, "Distance (mm): 3":refnum<vi>, "Surge Counts:":refnum<vi>, "Distance (mm): 2":refnum<vi>, "Distance (mm):":refnum<vi>, "Heave Counts:":refnum<vi>, "LRMHomeSurgeOffsetCounts":refnum<vi>, "LRMHomeSwayOffsetCounts":refnum<vi>, "TracHomeSurgeOffsetCounts 20MM":refnum<vi>, "TracHomeSwayOffsetCounts 20MM":refnum<vi>, "RotHomeSwayOffsetCounts":refnum<vi>, "RotHomeSurgeOffsetCounts":refnum<vi>, "Heave distance":refnum<vi>, "Zmm":refnum<vi>, "Heave Pulses/mm":refnum<vi>, "Surge Pulses/mm":refnum<vi>, "Sway Pulses/mm":refnum<vi>, "Heave Pitch":refnum<vi>, "Surge Pitch":refnum<vi>, "Sway Pitch":refnum<vi>, "Heave PPR":refnum<vi>, "Surge PPR":refnum<vi>, "Sway PPR":refnum<vi>, "Tab Control 5":refnum<vi>, "Tab Control 14":refnum<vi>, "Tab Control 26":refnum<vi>, "AE":refnum<vi>}, "Loading Com Port":cluster{"ClearAll":refnum<vi>, "Mz(Nm)":refnum<vi>, "My(Nm)":refnum<vi>, "Mx(Nm)":refnum<vi>, "Save Dwell":refnum<vi>, "Mx ":refnum<vi>, "My ":refnum<vi>, "Mz":refnum<vi>, "Fx(N)":refnum<vi>, "Fy(N)":refnum<vi>, "Fz(N)":refnum<vi>, "ZeroAll":refnum<vi>, "Acq Delay (ms)":refnum<vi>, "Burst Delay (ms)":refnum<vi>, "model":refnum<vi>, "SN":refnum<vi>, "FFx(N)":refnum<vi>, "Sensor IP":refnum<vi>, "Port":refnum<vi>, "FFy(N)":refnum<vi>, "Load(N)":refnum<vi>, "delete Handle":refnum<vi>, "Create Handle":refnum<vi>, "ft_data":refnum<vi>, "ft_range":refnum<vi>, "ft_data 2":refnum<vi>, "stop 6":refnum<vi>, "running_flag":refnum<vi>, "ft_udp_handle":refnum<vi>, "get-data-return":refnum<vi>, "get-range-return":refnum<vi>, "zero-return":refnum<vi>, "filter-return":refnum<vi>, "initial-return":refnum<vi>, "deleteHandle-result":refnum<vi>}}
  T12 = typedef "init queue out loop.ctl" = cluster{"UI Loop":refnum<queue>, "LOAD COM LOOP ":refnum<queue>, "SWAY MOTOR COM LOOP":refnum<queue>, "HEAVE MOTOR COM LOOP":refnum<queue>, "TEMPERATURE COM LOOP":refnum<queue>, "RAMP MOTOR COM LOOP":refnum<queue>, "ECR PORT":refnum<queue>, "HUMIDITY COM PORT":refnum<queue>, "PROGRAM LOOP":refnum<queue>, "MONITOR LOOP":refnum<queue>, "REPORT":refnum<queue>, "LOAD PID":refnum<queue>}
  T13 = enum8{"Enabled", "Disabled", "Disabled and Grayed Out"}
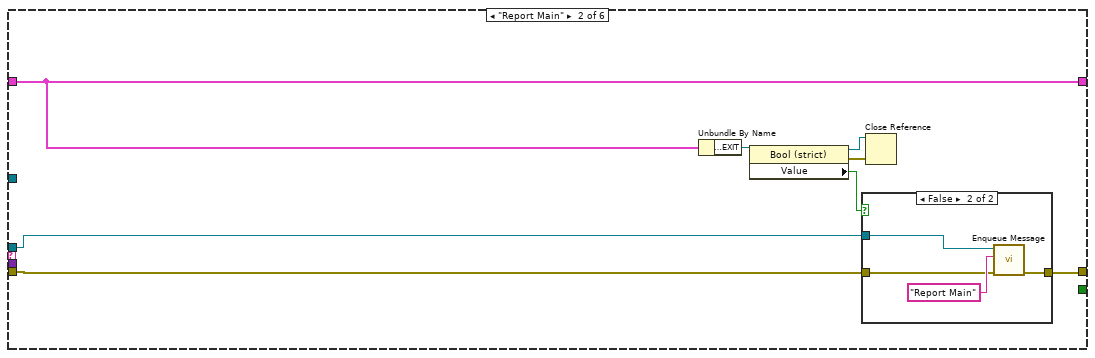
[diagram p2: hidden frame]
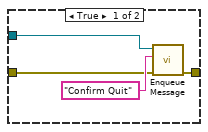
[diagram p3: hidden frame]
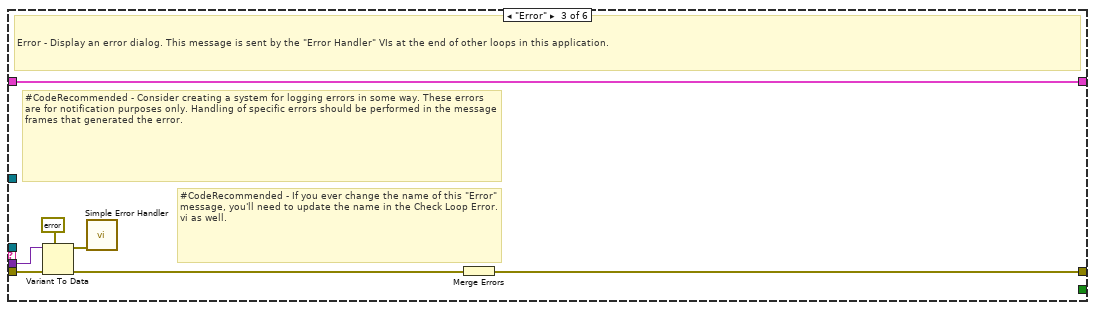
[diagram p4: hidden frame]
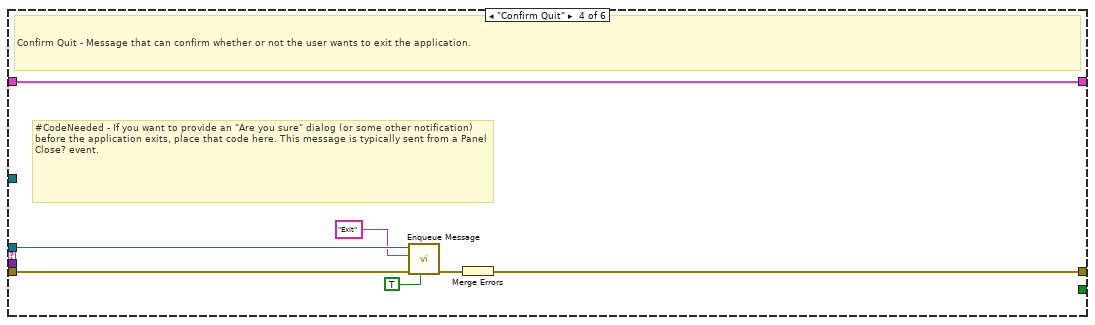
[diagram p5: hidden frame]
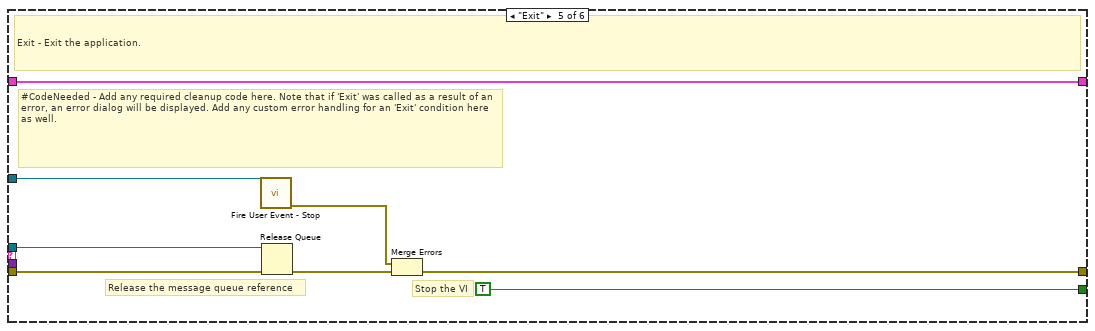
[diagram p6: hidden frame]
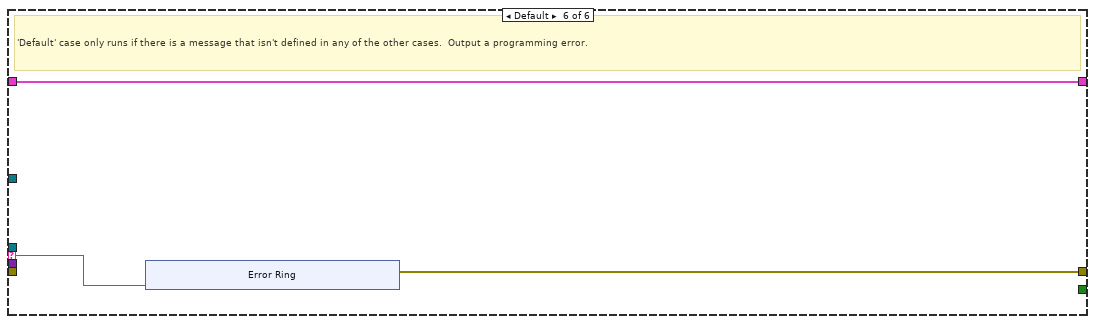
[diagram p7: hidden frame]
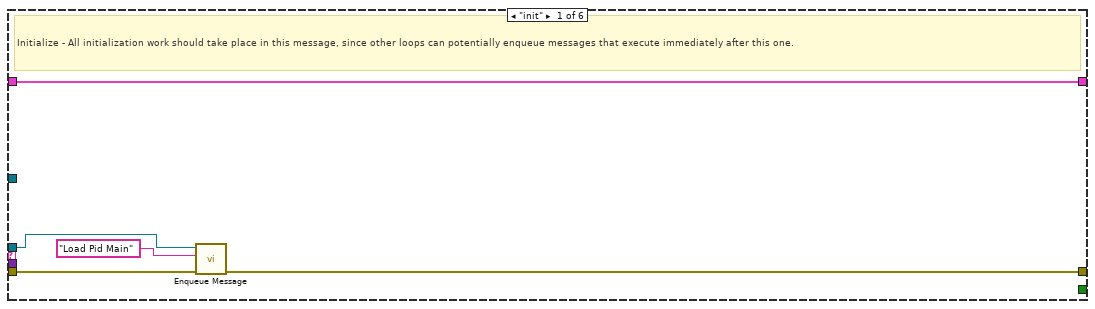
[diagram p8: hidden frame]
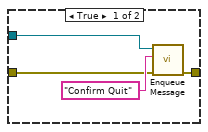
[diagram p9: hidden frame]
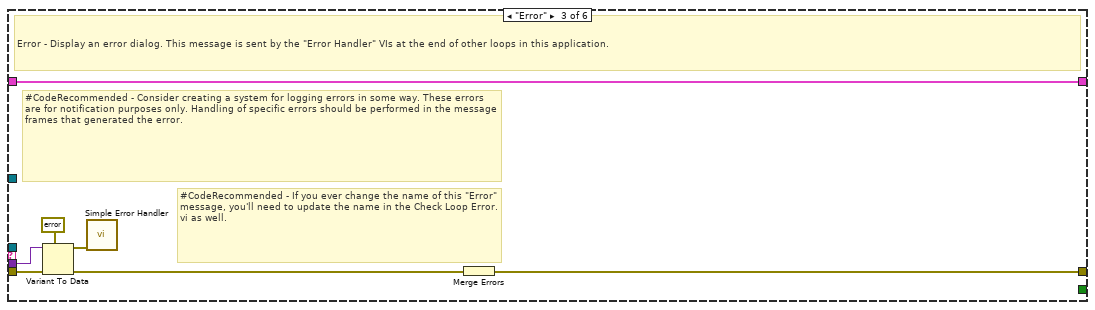
[diagram p10: hidden frame]
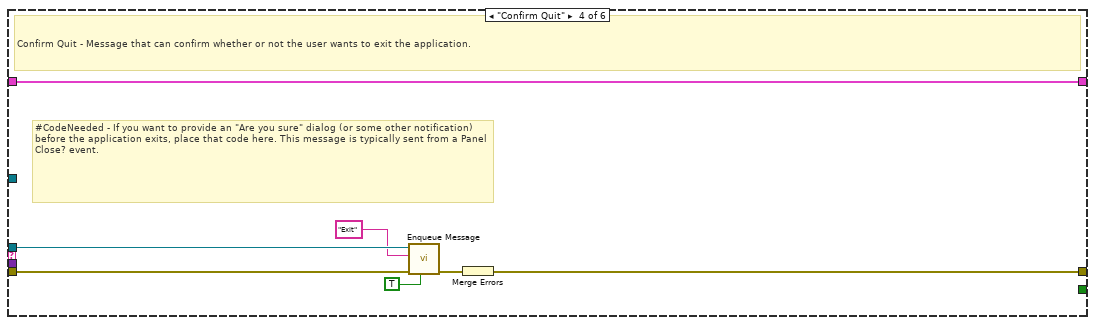
[diagram p11: hidden frame]
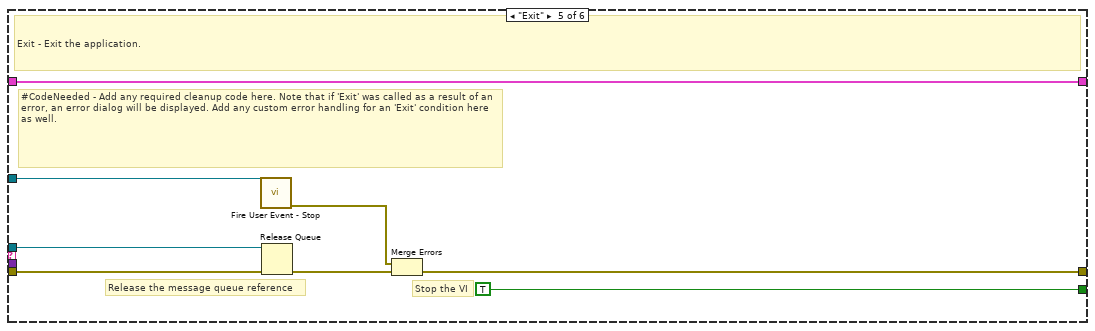
[diagram p12: hidden frame]
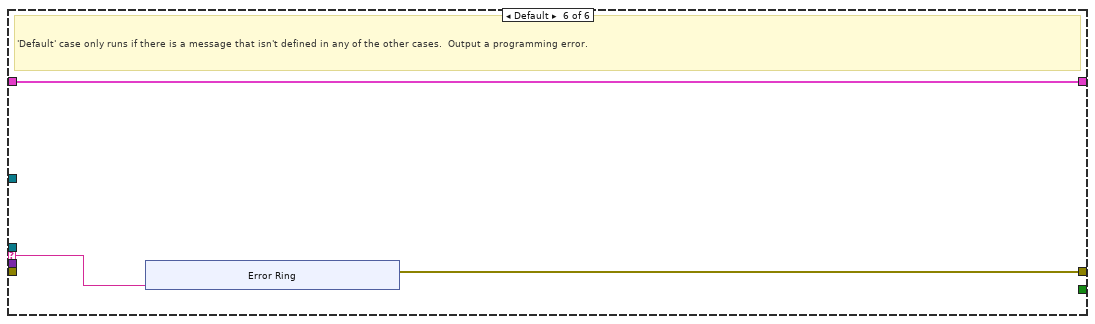
[diagram p13: hidden frame]
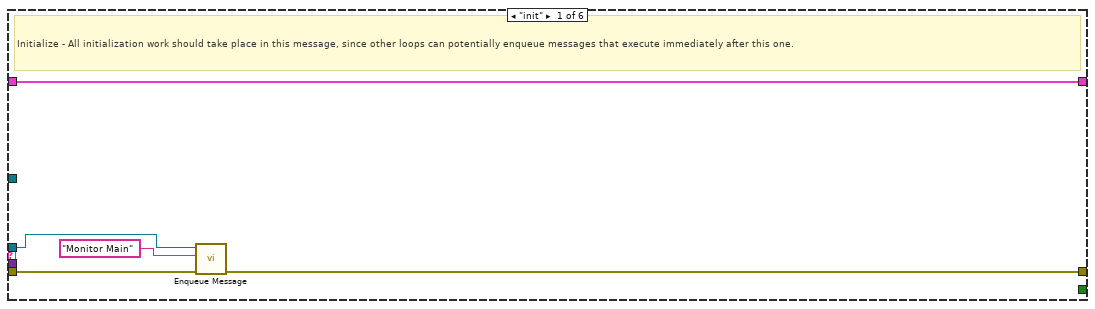
[diagram p14: hidden frame]
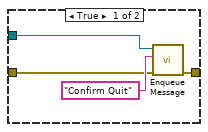
[diagram p15: hidden frame]
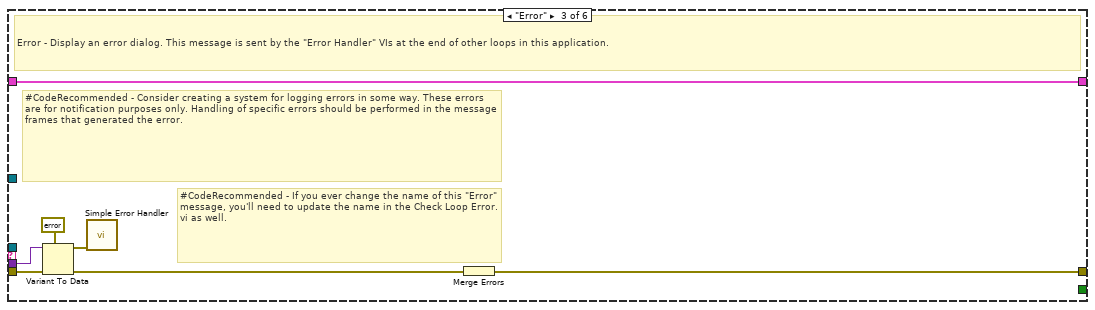
[diagram p16: hidden frame]
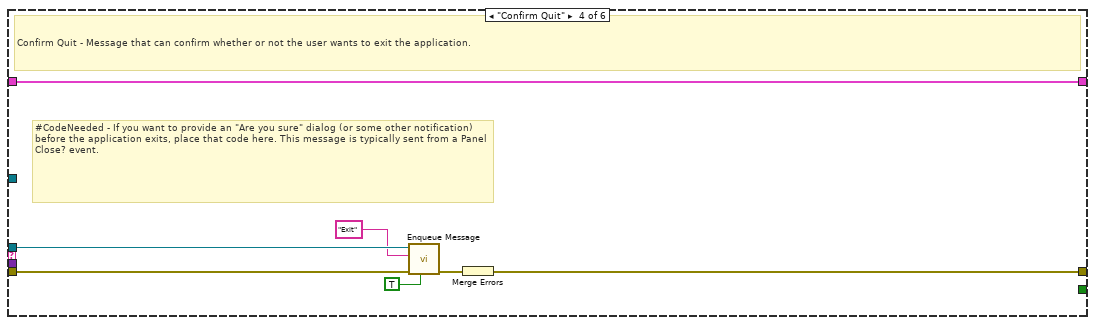
[diagram p17: hidden frame]
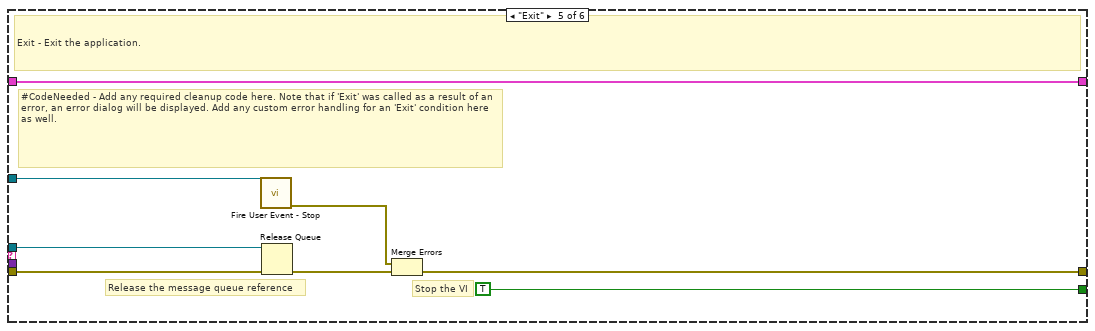
[diagram p18: hidden frame]
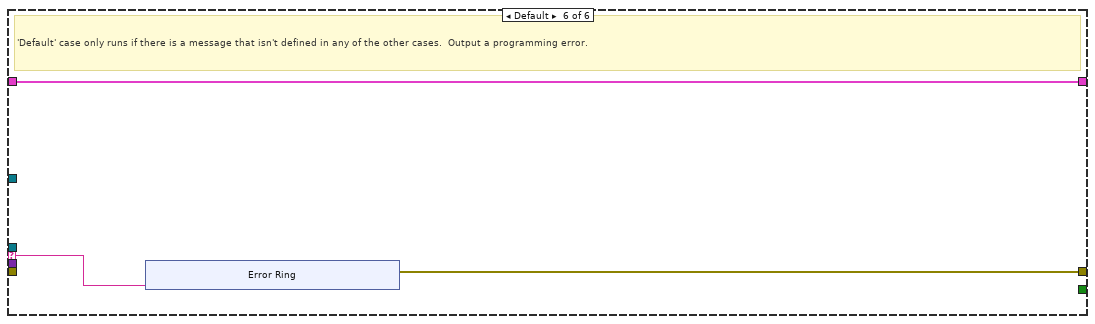
[diagram p19: hidden frame]
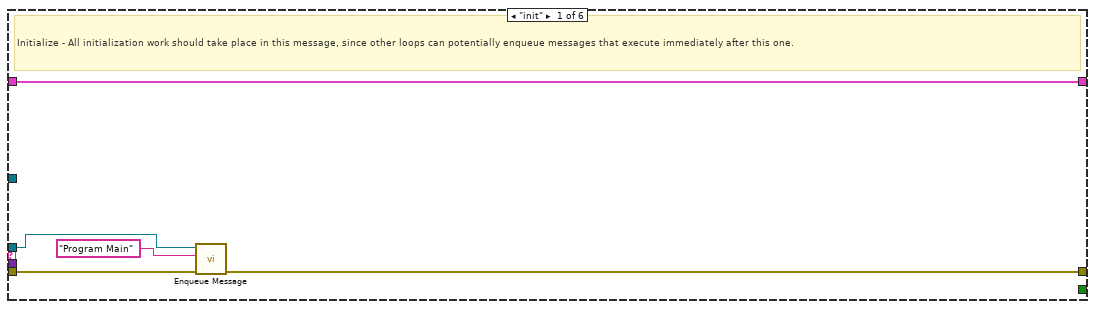
[diagram p20: hidden frame]
diagram:
  n1 = flat-sequence {
    tunnel: [w52] -> w39
    tunnel: T11 {"Main Home Screen"={"GUI"=refnum, "Platform Settings"=refnum, "Configure"=refnum, "Home"=refnum, "EXIT"=refnum, "service 2"=refnum, "MainPage"=refnum, "Analysis"=refnum}, "Platform Settings"={"mm/s  Surge"=refnum, "Update Surge Speed"=refnum, "Drive Error"=refnum, "Disable Axis Jog Soft Limits"=refnum, "mm/s  Sway"=refnum, "Sway and Surge COM Status"=refnum, "Heave COM Status"=refnum, "Enable Platform"=refnum, "Surge Forward Main"=refnum, "Sway Right Main"=refnum, "Sway Left Main"=refnum, "Heave Down Main"=refnum, "Heave Up main"=refnum, "Update Sway Speed"=refnum, "Update Heave Speed"=refnum, "mm/s Heave"=refnum, "mm/sec"=refnum, "mm"=refnum, "Surge Backward Main"=refnum}, "Analysis Screen"={"Analysis Home"=refnum, "Surface Analysis"=refnum, "Imaging"=refnum, "Image Analysis"=refnum, "Post Analysis"=refnum}, "Config Screen"={"Select Load Head"=refnum, "Notes :"=refnum, "FILE"=refnum, "Sample ID :"=refnum, "Operator ID :"=refnum, "Operator Name :"=refnum, "Auto"=refnum}, "Motion Module"={"zNL"=refnum, "NL disp"=refnum, "Rotary Tab"=refnum, "Motion Direction:  3"=refnum, "E.Velocity 2"=refnum, "e.v/ssr 2"=refnum, "Enter Fixed E.Velocity 2"=refnum, "Enter Final SRR 2"=refnum, "Enter initial SRR 2"=refnum, "Enter Fixed SRR 2"=refnum, "Enter the Final E.Velocity (m/s) 2"=refnum, "Enter initial E.Velocity (m/s) 2"=refnum, "Final Speed (RPM) 3"=refnum, "Initial Speed (RPM) 2"=refnum, "Enter the Final Velocity (m/s) 3"=refnum, "Enter initial Velocity (m/s)  3"=refnum, "Ramp Up 2"=refnum, "TEST SELECTION"=refnum, "SPEED SELECTION : "=refnum, "Angular Oscillation Set"=refnum, "Traction"=refnum, "Step Speed"=refnum, "StepTable For Load-Speed"=refnum, "StepTable For Speed"=refnum, "Surge Forward MM"=refnum, "Surge Backward MM"=refnum, "M3 Image"=refnum, "String 39"=refnum, "Sway Left MM"=refnum, "Sway Right MM"=refnum, "Disable Axis Jog Soft Limits"=refnum, "mm"=refnum, "Heave Down MM"=refnum, "Heave Up MM"=refnum, "Wear Track Diameter (mm)"=refnum, "Set WTD"=refnum, "HomeScratch"=refnum, "HomeRot"=refnum, "PlaceModule"=refnum, "Enter the Angle (Deg)"=refnum, "Enter the Frequency (Hz)"=refnum, "Motion Mode:"=refnum, "LR Sway"=refnum, "Rot Hor"=refnum, "Scratch"=refnum, "LR Cam"=refnum, "MMBack"=refnum, "MMNext"=refnum, "Rot Ver"=refnum, "Rotary Module Selection"=refnum, "calculate rotary"=refnum, "SPEED SELECTION : rotary"=refnum, "Import 2"=refnum, "Save 2"=refnum, "File Path :  2"=refnum, "String 45"=refnum, "StepTable For Speed 3"=refnum, "Enter the Speed(mm/sec)"=refnum, "Enter the Speed(RPM)"=refnum}, "Environmental control"={"Humidity  Status  3"=refnum, "Low Temp  Status  2"=refnum, "TK4 status 2"=refnum, "Stage Temperature"=refnum, "Sample Temperature"=refnum, "Humidity (Amb)"=refnum, "Clear List"=refnum, "Add to list"=refnum, "Wear"=refnum, "Vibration"=refnum, "Humidity (Chamber)"=refnum, "Temperature (Chamber)"=refnum, "ECR "=refnum, "Temperature (Amb)"=refnum, "Microphone"=refnum, "Acoustic Emission 3"=refnum, "SNext"=refnum, "APBack"=refnum, "Enter the Temperature (°C):"=refnum, "Enter the Stage \nTemperature (°C):"=refnum, "Enter the Humidity (%Rh):"=refnum, "Low Temp"=refnum, "High Temp"=refnum, "Humidity"=refnum, "Sensors Picked"=refnum}, "About Screen"={"Password"=refnum, "Home Service"=refnum, "Advanced Setting"=refnum, "About Tab"=refnum, "ECR Port:"=refnum, "Ramp Port:"=refnum, "Installation/Replacement completed"=refnum, "Loahead"=refnum, "Heave and Surge COM Port:"=refnum, "Sway COM Port:"=refnum, "Temp Modbus:"=refnum, "Humidity Port:"=refnum, "Edit Gain Constants"=refnum, "Save Gain Constants"=refnum}, "Main Screen"={"Main Screen Tab"=refnum, "Angle and Frequency"=refnum, "Stroke (mm)"=refnum, "Angle (Deg)"=refnum, "Main Speed Tab"=refnum, "MTM MOTOR DISPLAY"=refnum, "Disc Speed (m/sec)"=refnum, "Ball Speed (m/sec)"=refnum, "Disc Speed (RPM)"=refnum, "Ball Speed (RPM)"=refnum, "SPEED TAB"=refnum, "Speed (m/sec)"=refnum, "Set Speed (m/sec)"=refnum, "Speed (RPM)"=refnum, "Set Speed"=refnum, "Time Tab"=refnum, "Time ( HH:MM:SS ) 2"=refnum, "Test Duration"=refnum, "Test Duration 4"=refnum, "TEST CYCLE"=refnum, "TOTAL CYCLES"=refnum, "Set Load (N)"=refnum, "Temp Tabs"=refnum, "Heater"=refnum, "TK4 status"=refnum, "ChamberTemp"=refnum, "SetTmp"=refnum, "Controller  Status"=refnum, "ChamberTemp 2"=refnum, "SetTmp 2"=refnum, "Controller  Status 2"=refnum, "ChamberTemp 3"=refnum, "SetTmp 3"=refnum, "Cooling"=refnum, "Load Communication"=refnum, "Ambient \nTemperature"=refnum, "HumCOMStatus"=refnum, "Ambient\n Humidity"=refnum, "Freq (Hz)"=refnum, "Load En"=refnum, "NLt"=refnum, "zNL 2"=refnum, "Humidity On"=refnum, "humidity disp"=refnum, "Set Humidity"=refnum, "NL disp 2"=refnum, "Humidity On 2"=refnum, "humidity disp 2"=refnum, "Set Humidity 2"=refnum, "NL disp 3"=refnum, "AppLoadSeq scratch"=refnum, "Stop Scratch"=refnum, "ClrLog"=refnum, "Trip Log"=refnum, "STOP"=refnum, "Start Test"=refnum, "Test status"=refnum, "AR Led"=refnum, "Data"=refnum, "Health"=refnum, "Sway COM Status"=refnum, "Heave COM Status"=refnum, "Grp Tab"=refnum, "Sub Graph"=refnum, "SD (mm)"=refnum, "Siliding distance Reset Graph"=refnum, "SDGp"=refnum, "Humidity Reset Graph"=refnum, "HumrGp"=refnum, "Acoustic Emission (mV)"=refnum, "Aqucostic Reset Graph"=refnum, "gACQUOS"=refnum, "ECR RESET"=refnum, "ECR"=refnum, "Temperature Reset"=refnum, "Acoustic Emission (mV) 2"=refnum, "Aqucostic Reset Graph 2"=refnum, "gACQUOS 2"=refnum, "ECR RESET 2"=refnum, "ECR 2"=refnum, "Temperature Reset 2"=refnum, "Temperature (deg c)"=refnum, "Speed Reset Graph"=refnum, "Speed Tab"=refnum, "MTM DISC  SPEED"=refnum, "MTM BALL SPEED"=refnum, "speed mm/sec"=refnum, "Hymidity"=refnum, "Humidity Disable trip"=refnum, "CoF Trip  2"=refnum, "Depth Trip"=refnum, "Weart Deapth"=refnum, "Depth Reset Graph"=refnum, "Weart"=refnum, "Depthz"=refnum, "Depth (µm)"=refnum, "WearGp"=refnum, "NL Trip 2"=refnum, "Load pid"=refnum, "Load Disable Trip"=refnum, "Load Reset Graph"=refnum, "NL Display 4"=refnum, "Main Chart 3"=refnum, "BACK"=refnum, "Depth Trip 2"=refnum}, "Loading"={"Indentation"=refnum, "Reference Sample"=refnum, "Load Cell Communication Slide"=refnum, "com 3"=refnum, "com"=refnum, "DecaForce COM Status"=refnum, "Update"=refnum, "Clear 3"=refnum, "seq"=refnum, "Stribeck table"=refnum, "Stribeck Table  For loading"=refnum, "Loading Mode"=refnum, "Enter the Final Load (N)"=refnum, "Enter the CoF Trip"=refnum, "Enter the Friction Force Trip"=refnum, "Enter the Normal load Trip"=refnum, "Enter the Load  (N)"=refnum, "KiloForce"=refnum, "DecaForce "=refnum, "MicroForce"=refnum, "LHBack"=refnum, "LHNext"=refnum, "Enter the Loading Rate (N/min)"=refnum, "Message"=refnum, "Warning 2"=refnum, "SSP 0.75"=refnum, "SSP 0.5"=refnum, "SSP 0.3"=refnum, "Warning"=refnum, "gui GIF"=refnum, "Communication is established"=refnum, "AppLoad 4"=refnum, "Multipoint"=refnum, "Load Selection"=refnum}, "PID"={"Ramp MulFac"=refnum, "pulses LoadDiffRamp(2..10)"=refnum, "PulseControlRamp(diff<=3N)"=refnum, "SetLoadDeadband(%) Load(0-10N)"=refnum, "PID gains out delay (microForce)"=refnum, "Ramp"=refnum, "Gain 2"=refnum, "pulses LoadDiff(2..10)"=refnum, "pulses LoadDiff(11..50)"=refnum, "PulseControl(diff<=3N)"=refnum, "SetLoadDeadband(%)  2"=refnum, "Dummy Run"=refnum, "Vertical load (N)"=refnum, "AutoTune"=refnum, "Offset 3 "=refnum, "apply load"=refnum, "Offset  3"=refnum, "apply load 2"=refnum, "Enter ByPass Load"=refnum, "reinit 3"=refnum, "output range delay"=refnum, "PID gains out delay"=refnum, "Bypass Load"=refnum, "pulsesSent"=refnum, "pulses "=refnum, "actpid"=refnum, "gFF Rot"=refnum, "pulses LoadDiff(21..1000)"=refnum, "Delay"=refnum, "deadband"=refnum}, "Config Parameters"={"Tab Control 3"=refnum, "Tab Control 19"=refnum, "SAMPLES"=refnum, "Re-initilaize"=refnum, "Filter ON/OFF"=refnum, "TracHomeSurgeOffsetCounts 10MM"=refnum, "TracHomeSwayOffsetCounts 10MM"=refnum, "Acoustic Emission:"=refnum, "Apply Filter (FF)"=refnum, "Filter% 2"=refnum, "Apply Filter (Load)"=refnum, "Filter% "=refnum, "Sway distance (mm)"=refnum, "Surge distance (mm)"=refnum, "DataSavingLoopDelay(ms)"=refnum, "SAVE 2"=refnum, "Enter Distance"=refnum, "Sway Counts:"=refnum, "Distance (mm): 3"=refnum, "Surge Counts:"=refnum, "Distance (mm): 2"=refnum, "Distance (mm):"=refnum, "Heave Counts:"=refnum, "LRMHomeSurgeOffsetCounts"=refnum, "LRMHomeSwayOffsetCounts"=refnum, "TracHomeSurgeOffsetCounts 20MM"=refnum, "TracHomeSwayOffsetCounts 20MM"=refnum, "RotHomeSwayOffsetCounts"=refnum, "RotHomeSurgeOffsetCounts"=refnum, "Heave distance"=refnum, "Zmm"=refnum, "Heave Pulses/mm"=refnum, "Surge Pulses/mm"=refnum, "Sway Pulses/mm"=refnum, "Heave Pitch"=refnum, "Surge Pitch"=refnum, "Sway Pitch"=refnum, "Heave PPR"=refnum, "Surge PPR"=refnum, "Sway PPR"=refnum, "Tab Control 5"=refnum, "Tab Control 14"=refnum, "Tab Control 26"=refnum, "AE"=refnum}, "Loading Com Port"={"ClearAll"=refnum, "Mz(Nm)"=refnum, "My(Nm)"=refnum, "Mx(Nm)"=refnum, "Save Dwell"=refnum, "Mx "=refnum, "My "=refnum, "Mz"=refnum, "Fx(N)"=refnum, "Fy(N)"=refnum, "Fz(N)"=refnum, "ZeroAll"=refnum, "Acq Delay (ms)"=refnum, "Burst Delay (ms)"=refnum, "model"=refnum, "SN"=refnum, "FFx(N)"=refnum, "Sensor IP"=refnum, "Port"=refnum, "FFy(N)"=refnum, "Load(N)"=refnum, "delete Handle"=refnum, "Create Handle"=refnum, "ft_data"=refnum, "ft_range"=refnum, "ft_data 2"=refnum, "stop 6"=refnum, "running_flag"=refnum, "ft_udp_handle"=refnum, "get-data-return"=refnum, "get-range-return"=refnum, "zero-return"=refnum, "filter-return"=refnum, "initial-return"=refnum, "deleteHandle-result"=refnum}} ("Data Cluster") -> [w51]
    tunnel: w39 -> [w81]
    tunnel: [w61] -> w38
    tunnel: w38 -> [w88]
    tunnel: [w82] -> w37
    tunnel: w37 -> [w97]
    tunnel: [w96] -> w36
    tunnel: w36 -> [w133]
    tunnel: [w132] -> w34
    tunnel: w34 -> [w194]
    tunnel: [w193] -> w33
    tunnel: w33 -> [w221]
    tunnel: [w220] -> w32
    tunnel: w32 -> [w237]
    tunnel: [w236] -> w31
    tunnel: w31 -> [w330]
    tunnel: [w329] -> w3
    tunnel: w3 -> [w360]
    tunnel: [w359] -> w2
    tunnel: w2 -> [w406]
    tunnel: [w405] -> w1
    tunnel: [w441] -> w9
    tunnel: w1 -> [w442]
    frame #0 {
      n2 = control-ref of="GUI"() -> (w60:refnum<vi>)
      n3 = control-ref of="MainPage"() -> (w54:refnum<vi>)
      n4 = control-ref of="Platform Settings"() -> (w59:refnum<vi>)
      n5 = control-ref of="Configure"() -> (w58:refnum<vi>)
      n6 = control-ref of="Home"() -> (w57:refnum<vi>)
      n7 = control-ref of="EXIT"() -> (w56:refnum<vi>)
      n8 = control-ref of="service 2"() -> (w55:refnum<vi>)
      n9 = control-ref of="Analysis"() -> (w53:refnum<vi>)
      n10 = Bundle By Name(cluster=w51, "Main Home Screen.GUI"=w60, "Main Home Screen.Platform Settings"=w59, "Main Home Screen.Configure"=w58, "Main Home Screen.Home"=w57, "Main Home Screen.EXIT"=w56, "Main Home Screen.service 2"=w55, "Main Home Screen.MainPage"=w54, "Main Home Screen.Analysis"=w53) -> (w52:T11)
    }
    frame #1 {
      n11 = control-ref of="Sway Right Main"() -> (w71:refnum<vi>)
      n12 = control-ref of="Sway Left Main"() -> (w70:refnum<vi>)
      n13 = control-ref of="Heave Down Main"() -> (w69:refnum<vi>)
      n14 = control-ref of="Heave Up main"() -> (w68:refnum<vi>)
      n15 = control-ref of="Update Sway Speed"() -> (w67:refnum<vi>)
      n16 = control-ref of="Update Heave Speed"() -> (w66:refnum<vi>)
      n17 = control-ref of="Surge Backward Main"() -> (w62:refnum<vi>)
      n18 = control-ref of="Update Surge Speed"() -> (w79:refnum<vi>)
      n19 = control-ref of="Disable Axis Jog Soft Limits"() -> (w77:refnum<vi>)
      n20 = control-ref of="Sway and Surge COM Status"() -> (w75:refnum<vi>)
      n21 = control-ref of="Heave COM Status"() -> (w74:refnum<vi>)
      n22 = control-ref of="Enable Platform"() -> (w73:refnum<vi>)
      n23 = control-ref of="Surge Forward Main"() -> (w72:refnum<vi>)
      n24 = control-ref of="mm/s Heave"() -> (w65:refnum<vi>)
      n25 = control-ref of="mm/sec"() -> (w64:refnum<vi>)
      n26 = control-ref of="mm"() -> (w63:refnum<vi>)
      n27 = control-ref of="mm/s  Surge"() -> (w80:refnum<vi>)
      n28 = control-ref of="mm/s  Sway"() -> (w76:refnum<vi>)
      n29 = control-ref of="Drive Error"() -> (w78:refnum<vi>)
      n30 = Bundle By Name(cluster=w81, "Platform Settings.mm/s  Surge"=w80, "Platform Settings.Update Surge Speed"=w79, "Platform Settings.Drive Error"=w78, "Platform Settings.Disable Axis Jog Soft Limits"=w77, "Platform Settings.mm/s  Sway"=w76, "Platform Settings.Sway and Surge COM Status"=w75, "Platform Settings.Heave COM Status"=w74, "Platform Settings.Enable Platform"=w73, "Platform Settings.Surge Forward Main"=w72, "Platform Settings.Sway Right Main"=w71, "Platform Settings.Sway Left Main"=w70, "Platform Settings.Heave Down Main"=w69, "Platform Settings.Heave Up main"=w68, "Platform Settings.Update Sway Speed"=w67, "Platform Settings.Update Heave Speed"=w66, "Platform Settings.mm/s Heave"=w65, "Platform Settings.mm/sec"=w64, "Platform Settings.mm"=w63, "Platform Settings.Surge Backward Main"=w62) -> (w61:T11)
    }
    frame #2 {
      n31 = control-ref of="Analysis Home"() -> (w87:refnum<vi>)
      n32 = control-ref of="Surface Analysis"() -> (w86:refnum<vi>)
      n33 = control-ref of="Imaging"() -> (w85:refnum<vi>)
      n34 = control-ref of="Image Analysis"() -> (w84:refnum<vi>)
      n35 = control-ref of="Post Analysis"() -> (w83:refnum<vi>)
      n36 = Bundle By Name(cluster=w88, "Analysis Screen.Analysis Home"=w87, "Analysis Screen.Surface Analysis"=w86, "Analysis Screen.Imaging"=w85, "Analysis Screen.Image Analysis"=w84, "Analysis Screen.Post Analysis"=w83) -> (w82:T11)
    }
    frame #3 {
      n37 = control-ref of="Select Load Head"() -> (w95:refnum<vi>)
      n38 = control-ref of="Auto"() -> (w89:refnum<vi>)
      n39 = control-ref of="Notes :"() -> (w94:refnum<vi>)
      n40 = control-ref of="FILE"() -> (w93:refnum<vi>)
      n41 = control-ref of="Sample ID :"() -> (w92:refnum<vi>)
      n42 = control-ref of="Operator ID :"() -> (w91:refnum<vi>)
      n43 = control-ref of="Operator Name :"() -> (w90:refnum<vi>)
      n44 = Bundle By Name(cluster=w97, "Config Screen.Select Load Head"=w95, "Config Screen.Notes :"=w94, "Config Screen.FILE"=w93, "Config Screen.Sample ID :"=w92, "Config Screen.Operator ID :"=w91, "Config Screen.Operator Name :"=w90, "Config Screen.Auto"=w89) -> (w96:T11)
    }
    frame #4 {
      n45 = control-ref of="Warning"() -> (w125:refnum<vi>)
      n46 = control-ref of="gui GIF"() -> (w124:refnum<vi>)
      n47 = control-ref of="Load Selection"() -> (w98:refnum<vi>)
      n48 = control-ref of="Warning 2"() -> (w129:refnum<vi>)
      n49 = control-ref of="SSP 0.75"() -> (w128:refnum<vi>)
      n50 = control-ref of="SSP 0.5"() -> (w127:refnum<vi>)
      n51 = control-ref of="SSP 0.3"() -> (w126:refnum<vi>)
      n52 = control-ref of="Communication is established"() -> (w123:refnum<vi>)
      n53 = control-ref of="AppLoad 4"() -> (w122:refnum<vi>)
      n54 = control-ref of="Multipoint"() -> (w121:refnum<vi>)
      n55 = control-ref of="com 3"() -> (w117:refnum<vi>)
      n56 = control-ref of="com"() -> (w116:refnum<vi>)
      n57 = control-ref of="DecaForce COM Status"() -> (w115:refnum<vi>)
      n58 = control-ref of="Update"() -> (w114:refnum<vi>)
      n59 = control-ref of="Clear 3"() -> (w113:refnum<vi>)
      n60 = control-ref of="seq"() -> (w112:refnum<vi>)
      n61 = control-ref of="Stribeck table"() -> (w111:refnum<vi>)
      n62 = control-ref of="KiloForce"() -> (w103:refnum<vi>)
      n63 = control-ref of="DecaForce"() -> (w102:refnum<vi>)
      n64 = control-ref of="MicroForce"() -> (w101:refnum<vi>)
      n65 = control-ref of="LHBack"() -> (w100:refnum<vi>)
      n66 = control-ref of="LHNext"() -> (w99:refnum<vi>)
      n67 = control-ref of="Enter the Loading Rate (N/min)"() -> (w131:refnum<vi>)
      n68 = control-ref of="Enter the Final Load (N)"() -> (w108:refnum<vi>)
      n69 = control-ref of="Enter the CoF Trip"() -> (w107:refnum<vi>)
      n70 = control-ref of="Enter the Friction Force Trip"() -> (w106:refnum<vi>)
      n71 = control-ref of="Enter the Normal load Trip"() -> (w105:refnum<vi>)
      n72 = control-ref of="Enter the Load  (N)"() -> (w104:refnum<vi>)
      n73 = control-ref of="Message"() -> (w130:refnum<vi>)
      n74 = control-ref of="Indentation"() -> (w120:refnum<vi>)
      n75 = control-ref of="Stribeck Table  For loading"() -> (w110:refnum<vi>)
      n76 = control-ref of="Reference Sample"() -> (w119:refnum<vi>)
      n77 = control-ref of="Load Cell Communication Slide"() -> (w118:refnum<vi>)
      n78 = control-ref of="Loading Mode"() -> (w109:refnum<vi>)
      n79 = Bundle By Name(cluster=w133, "Loading.Enter the Loading Rate (N/min)"=w131, "Loading.Message"=w130, "Loading.Warning 2"=w129, "Loading.SSP 0.75"=w128, "Loading.SSP 0.5"=w127, "Loading.SSP 0.3"=w126, "Loading.Warning"=w125, "Loading.gui GIF"=w124, "Loading.Communication is established"=w123, "Loading.AppLoad 4"=w122, "Loading.Multipoint"=w121, "Loading.Indentation"=w120, "Loading.Reference Sample"=w119, "Loading.Load Cell Communication Slide"=w118, "Loading.com 3"=w117, "Loading.com"=w116, "Loading.DecaForce COM Status"=w115, "Loading.Update"=w114, "Loading.Clear 3"=w113, "Loading.seq"=w112, "Loading.Stribeck table"=w111, "Loading.Stribeck Table  For loading"=w110, "Loading.Loading Mode"=w109, "Loading.Enter the Final Load (N)"=w108, "Loading.Enter the CoF Trip"=w107, "Loading.Enter the Friction Force Trip"=w106, "Loading.Enter the Normal load Trip"=w105, "Loading.Enter the Load  (N)"=w104, "Loading.KiloForce"=w103, "Loading.DecaForce"=w102, "Loading.MicroForce"=w101, "Loading.LHBack"=w100, "Loading.LHNext"=w99, "Loading.Load Selection"=w98) -> (w132:T11)
    }
    frame #5 {
      n80 = control-ref of="TEST SELECTION"() -> (w175:refnum<vi>)
      n81 = control-ref of="SPEED SELECTION :"() -> (w174:refnum<vi>)
      n82 = control-ref of="SPEED SELECTION : rotary"() -> (w141:refnum<vi>)
      n83 = control-ref of="Rotary Tab"() -> (w190:refnum<vi>)
      n84 = control-ref of="e.v/ssr 2"() -> (w187:refnum<vi>)
      n85 = control-ref of="Step Speed"() -> (w171:refnum<vi>)
      n86 = control-ref of="M3 Image"() -> (w166:refnum<vi>)
      n87 = control-ref of="Rotary Module Selection"() -> (w143:refnum<vi>)
      n88 = control-ref of="zNL"() -> (w192:refnum<vi>)
      n89 = control-ref of="E.Velocity 2"() -> (w188:refnum<vi>)
      n90 = control-ref of="Ramp Up 2"() -> (w176:refnum<vi>)
      n91 = control-ref of="Angular Oscillation Set"() -> (w173:refnum<vi>)
      n92 = control-ref of="Traction"() -> (w172:refnum<vi>)
      n93 = control-ref of="Surge Forward MM"() -> (w168:refnum<vi>)
      n94 = control-ref of="Surge Backward MM"() -> (w167:refnum<vi>)
      n95 = control-ref of="Sway Left MM"() -> (w164:refnum<vi>)
      n96 = control-ref of="Sway Right MM"() -> (w163:refnum<vi>)
      n97 = control-ref of="Disable Axis Jog Soft Limits"() -> (w162:refnum<vi>)
      n98 = control-ref of="Heave Down MM"() -> (w160:refnum<vi>)
      n99 = control-ref of="Heave Up MM"() -> (w159:refnum<vi>)
      n100 = control-ref of="Set WTD"() -> (w157:refnum<vi>)
      n101 = control-ref of="HomeScratch"() -> (w156:refnum<vi>)
      n102 = control-ref of="HomeRot"() -> (w155:refnum<vi>)
      n103 = control-ref of="PlaceModule"() -> (w154:refnum<vi>)
      n104 = control-ref of="LR Sway"() -> (w150:refnum<vi>)
      n105 = control-ref of="Rot Hor"() -> (w149:refnum<vi>)
      n106 = control-ref of="Scratch"() -> (w148:refnum<vi>)
      n107 = control-ref of="LR Cam"() -> (w147:refnum<vi>)
      n108 = control-ref of="MMBack"() -> (w146:refnum<vi>)
      n109 = control-ref of="MMNext"() -> (w145:refnum<vi>)
      n110 = control-ref of="Rot Ver"() -> (w144:refnum<vi>)
      n111 = control-ref of="calculate rotary"() -> (w142:refnum<vi>)
      n112 = control-ref of="Import 2"() -> (w140:refnum<vi>)
      n113 = control-ref of="Save 2"() -> (w139:refnum<vi>)
      n114 = control-ref of="NL disp"() -> (w191:refnum<vi>)
      n115 = control-ref of="Enter Fixed E.Velocity 2"() -> (w186:refnum<vi>)
      n116 = control-ref of="Enter Final SRR 2"() -> (w185:refnum<vi>)
      n117 = control-ref of="Enter initial SRR 2"() -> (w184:refnum<vi>)
      n118 = control-ref of="Enter Fixed SRR 2"() -> (w183:refnum<vi>)
      n119 = control-ref of="Enter the Final E.Velocity (m/s) 2"() -> (w182:refnum<vi>)
      n120 = control-ref of="Enter initial E.Velocity (m/s) 2"() -> (w181:refnum<vi>)
      n121 = control-ref of="Final Speed (RPM) 3"() -> (w180:refnum<vi>)
      n122 = control-ref of="Initial Speed (RPM) 2"() -> (w179:refnum<vi>)
      n123 = control-ref of="Enter the Final Velocity (m/s) 3"() -> (w178:refnum<vi>)
      n124 = control-ref of="Enter initial Velocity (m/s)  3"() -> (w177:refnum<vi>)
      n125 = control-ref of="mm"() -> (w161:refnum<vi>)
      n126 = control-ref of="Wear Track Diameter (mm)"() -> (w158:refnum<vi>)
      n127 = control-ref of="Enter the Angle (Deg)"() -> (w153:refnum<vi>)
      n128 = control-ref of="Enter the Frequency (Hz)"() -> (w152:refnum<vi>)
      n129 = control-ref of="Enter the Speed(mm/sec)"() -> (w135:refnum<vi>)
      n130 = control-ref of="Enter the Speed(RPM)"() -> (w134:refnum<vi>)
      n131 = control-ref of="String 39"() -> (w165:refnum<vi>)
      n132 = control-ref of="String 45"() -> (w137:refnum<vi>)
      n133 = control-ref of="StepTable For Load-Speed"() -> (w170:refnum<vi>)
      n134 = control-ref of="StepTable For Speed"() -> (w169:refnum<vi>)
      n135 = control-ref of="Motion Direction:  3"() -> (w189:refnum<vi>)
      n136 = control-ref of="Motion Mode:"() -> (w151:refnum<vi>)
      n137 = control-ref of="StepTable For Speed 3"() -> (w136:refnum<vi>)
      n138 = control-ref of="File Path :  2"() -> (w138:refnum<vi>)
      n139 = Bundle By Name(cluster=w194, "Motion Module.zNL"=w192, "Motion Module.NL disp"=w191, "Motion Module.Rotary Tab"=w190, "Motion Module.Motion Direction:  3"=w189, "Motion Module.E.Velocity 2"=w188, "Motion Module.e.v/ssr 2"=w187, "Motion Module.Enter Fixed E.Velocity 2"=w186, "Motion Module.Enter Final SRR 2"=w185, "Motion Module.Enter initial SRR 2"=w184, "Motion Module.Enter Fixed SRR 2"=w183, "Motion Module.Enter the Final E.Velocity (m/s) 2"=w182, "Motion Module.Enter initial E.Velocity (m/s) 2"=w181, "Motion Module.Final Speed (RPM) 3"=w180, "Motion Module.Initial Speed (RPM) 2"=w179, "Motion Module.Enter the Final Velocity (m/s) 3"=w178, "Motion Module.Enter initial Velocity (m/s)  3"=w177, "Motion Module.Ramp Up 2"=w176, "Motion Module.TEST SELECTION"=w175, "Motion Module.SPEED SELECTION :"=w174, "Motion Module.Angular Oscillation Set"=w173, "Motion Module.Traction"=w172, "Motion Module.Step Speed"=w171, "Motion Module.StepTable For Load-Speed"=w170, "Motion Module.StepTable For Speed"=w169, "Motion Module.Surge Forward MM"=w168, "Motion Module.Surge Backward MM"=w167, "Motion Module.M3 Image"=w166, "Motion Module.String 39"=w165, "Motion Module.Sway Left MM"=w164, "Motion Module.Sway Right MM"=w163, "Motion Module.Disable Axis Jog Soft Limits"=w162, "Motion Module.mm"=w161, "Motion Module.Heave Down MM"=w160, "Motion Module.Heave Up MM"=w159, "Motion Module.Wear Track Diameter (mm)"=w158, "Motion Module.Set WTD"=w157, "Motion Module.HomeScratch"=w156, "Motion Module.HomeRot"=w155, "Motion Module.PlaceModule"=w154, "Motion Module.Enter the Angle (Deg)"=w153, "Motion Module.Enter the Frequency (Hz)"=w152, "Motion Module.Motion Mode:"=w151, "Motion Module.LR Sway"=w150, "Motion Module.Rot Hor"=w149, "Motion Module.Scratch"=w148, "Motion Module.LR Cam"=w147, "Motion Module.MMBack"=w146, "Motion Module.MMNext"=w145, "Motion Module.Rot Ver"=w144, "Motion Module.Rotary Module Selection"=w143, "Motion Module.calculate rotary"=w142, "Motion Module.SPEED SELECTION : rotary"=w141, "Motion Module.Import 2"=w140, "Motion Module.Save 2"=w139, "Motion Module.File Path :  2"=w138, "Motion Module.String 45"=w137, "Motion Module.StepTable For Speed 3"=w136, "Motion Module.Enter the Speed(mm/sec)"=w135, "Motion Module.Enter the Speed(RPM)"=w134) -> (w193:T11)
    }
    frame #6 {
      n140 = control-ref of="Add to list"() -> (w212:refnum<vi>)
      n141 = control-ref of="Wear"() -> (w211:refnum<vi>)
      n142 = control-ref of="Vibration"() -> (w210:refnum<vi>)
      n143 = control-ref of="Humidity (Chamber)"() -> (w209:refnum<vi>)
      n144 = control-ref of="Temperature (Chamber)"() -> (w208:refnum<vi>)
      n145 = control-ref of="ECR"() -> (w207:refnum<vi>)
      n146 = control-ref of="Temperature (Amb)"() -> (w206:refnum<vi>)
      n147 = control-ref of="Microphone"() -> (w205:refnum<vi>)
      n148 = control-ref of="Acoustic Emission 3"() -> (w204:refnum<vi>)
      n149 = control-ref of="SNext"() -> (w203:refnum<vi>)
      n150 = control-ref of="APBack"() -> (w202:refnum<vi>)
      n151 = control-ref of="Low Temp"() -> (w198:refnum<vi>)
      n152 = control-ref of="High Temp"() -> (w197:refnum<vi>)
      n153 = control-ref of="Humidity"() -> (w196:refnum<vi>)
      n154 = control-ref of="Humidity  Status  3"() -> (w219:refnum<vi>)
      n155 = control-ref of="Low Temp  Status  2"() -> (w218:refnum<vi>)
      n156 = control-ref of="TK4 status 2"() -> (w217:refnum<vi>)
      n157 = control-ref of="Humidity (Amb)"() -> (w214:refnum<vi>)
      n158 = control-ref of="Clear List"() -> (w213:refnum<vi>)
      n159 = control-ref of="Enter the Temperature (°C):"() -> (w201:refnum<vi>)
      n160 = control-ref of="Enter the Stage \nTemperature (°C):"() -> (w200:refnum<vi>)
      n161 = control-ref of="Enter the Humidity (%Rh):"() -> (w199:refnum<vi>)
      n162 = control-ref of="Sensors Picked"() -> (w195:refnum<vi>)
      n163 = control-ref of="Stage Temperature"() -> (w216:refnum<vi>)
      n164 = control-ref of="Sample Temperature"() -> (w215:refnum<vi>)
      n165 = Bundle By Name(cluster=w221, "Environmental control.Humidity  Status  3"=w219, "Environmental control.Low Temp  Status  2"=w218, "Environmental control.TK4 status 2"=w217, "Environmental control.Stage Temperature"=w216, "Environmental control.Sample Temperature"=w215, "Environmental control.Humidity (Amb)"=w214, "Environmental control.Clear List"=w213, "Environmental control.Add to list"=w212, "Environmental control.Wear"=w211, "Environmental control.Vibration"=w210, "Environmental control.Humidity (Chamber)"=w209, "Environmental control.Temperature (Chamber)"=w208, "Environmental control.ECR"=w207, "Environmental control.Temperature (Amb)"=w206, "Environmental control.Microphone"=w205, "Environmental control.Acoustic Emission 3"=w204, "Environmental control.SNext"=w203, "Environmental control.APBack"=w202, "Environmental control.Enter the Temperature (°C):"=w201, "Environmental control.Enter the Stage \nTemperature (°C):"=w200, "Environmental control.Enter the Humidity (%Rh):"=w199, "Environmental control.Low Temp"=w198, "Environmental control.High Temp"=w197, "Environmental control.Humidity"=w196, "Environmental control.Sensors Picked"=w195) -> (w220:T11)
    }
    frame #7 {
      n166 = control-ref of="ECR Port:"() -> (w231:refnum<vi>)
      n167 = control-ref of="Ramp Port:"() -> (w230:refnum<vi>)
      n168 = control-ref of="Heave and Surge COM Port:"() -> (w227:refnum<vi>)
      n169 = control-ref of="Sway COM Port:"() -> (w226:refnum<vi>)
      n170 = control-ref of="Temp Modbus:"() -> (w225:refnum<vi>)
      n171 = control-ref of="Humidity Port:"() -> (w224:refnum<vi>)
      n172 = control-ref of="About Tab"() -> (w232:refnum<vi>)
      n173 = control-ref of="Home Service"() -> (w234:refnum<vi>)
      n174 = control-ref of="Advanced Setting"() -> (w233:refnum<vi>)
      n175 = control-ref of="Installation/Replacement completed"() -> (w229:refnum<vi>)
      n176 = control-ref of="Loahead"() -> (w228:refnum<vi>)
      n177 = control-ref of="Edit Gain Constants"() -> (w223:refnum<vi>)
      n178 = control-ref of="Save Gain Constants"() -> (w222:refnum<vi>)
      n179 = control-ref of="Password"() -> (w235:refnum<vi>)
      n180 = Bundle By Name(cluster=w237, "About Screen.Password"=w235, "About Screen.Home Service"=w234, "About Screen.Advanced Setting"=w233, "About Screen.About Tab"=w232, "About Screen.ECR Port:"=w231, "About Screen.Ramp Port:"=w230, "About Screen.Installation/Replacement completed"=w229, "About Screen.Loahead"=w228, "About Screen.Heave and Surge COM Port:"=w227, "About Screen.Sway COM Port:"=w226, "About Screen.Temp Modbus:"=w225, "About Screen.Humidity Port:"=w224, "About Screen.Edit Gain Constants"=w223, "About Screen.Save Gain Constants"=w222) -> (w236:T11)
    }
    frame #8 {
      n181 = control-ref of="SDGp"() -> (w269:refnum<vi>)
      n182 = control-ref of="HumrGp"() -> (w267:refnum<vi>)
      n183 = control-ref of="gACQUOS"() -> (w264:refnum<vi>)
      n184 = control-ref of="ECR"() -> (w262:refnum<vi>)
      n185 = control-ref of="Temperature (deg c)"() -> (w260:refnum<vi>)
      n186 = control-ref of="MTM DISC  SPEED"() -> (w257:refnum<vi>)
      n187 = control-ref of="MTM BALL SPEED"() -> (w256:refnum<vi>)
      n188 = control-ref of="speed mm/sec"() -> (w255:refnum<vi>)
      n189 = control-ref of="WearGp"() -> (w245:refnum<vi>)
      n190 = control-ref of="Main Chart 3"() -> (w239:refnum<vi>)
      n191 = control-ref of="Main Screen Tab"() -> (w328:refnum<vi>)
      n192 = control-ref of="Angle and Frequency"() -> (w327:refnum<vi>)
      n193 = control-ref of="Main Speed Tab"() -> (w324:refnum<vi>)
      n194 = control-ref of="MTM MOTOR DISPLAY"() -> (w323:refnum<vi>)
      n195 = control-ref of="SPEED TAB"() -> (w318:refnum<vi>)
      n196 = control-ref of="Time Tab"() -> (w313:refnum<vi>)
      n197 = control-ref of="Temp Tabs"() -> (w306:refnum<vi>)
      n198 = control-ref of="Grp Tab"() -> (w273:refnum<vi>)
      n199 = control-ref of="Sub Graph"() -> (w272:refnum<vi>)
      n200 = control-ref of="Speed Tab"() -> (w258:refnum<vi>)
      n201 = control-ref of="Heater"() -> (w305:refnum<vi>)
      n202 = control-ref of="TK4 status"() -> (w304:refnum<vi>)
      n203 = control-ref of="Controller  Status"() -> (w301:refnum<vi>)
      n204 = control-ref of="Cooling"() -> (w298:refnum<vi>)
      n205 = control-ref of="Load Communication"() -> (w297:refnum<vi>)
      n206 = control-ref of="HumCOMStatus"() -> (w295:refnum<vi>)
      n207 = control-ref of="Load En"() -> (w292:refnum<vi>)
      n208 = control-ref of="NLt"() -> (w291:refnum<vi>)
      n209 = control-ref of="zNL 2"() -> (w290:refnum<vi>)
      n210 = control-ref of="Humidity On"() -> (w289:refnum<vi>)
      n211 = control-ref of="AppLoadSeq scratch"() -> (w285:refnum<vi>)
      n212 = control-ref of="Stop Scratch"() -> (w284:refnum<vi>)
      n213 = control-ref of="ClrLog"() -> (w283:refnum<vi>)
      n214 = control-ref of="STOP"() -> (w281:refnum<vi>)
      n215 = control-ref of="Start Test"() -> (w280:refnum<vi>)
      n216 = control-ref of="Test status"() -> (w279:refnum<vi>)
      n217 = control-ref of="AR Led"() -> (w278:refnum<vi>)
      n218 = control-ref of="Data"() -> (w277:refnum<vi>)
      n219 = control-ref of="Health"() -> (w276:refnum<vi>)
      n220 = control-ref of="Sway COM Status"() -> (w275:refnum<vi>)
      n221 = control-ref of="Heave COM Status"() -> (w274:refnum<vi>)
      n222 = control-ref of="Siliding distance Reset Graph"() -> (w270:refnum<vi>)
      n223 = control-ref of="Humidity Reset Graph"() -> (w268:refnum<vi>)
      n224 = control-ref of="Aqucostic Reset Graph"() -> (w265:refnum<vi>)
      n225 = control-ref of="ECR RESET"() -> (w263:refnum<vi>)
      n226 = control-ref of="Temperature Reset"() -> (w261:refnum<vi>)
      n227 = control-ref of="Speed Reset Graph"() -> (w259:refnum<vi>)
      n228 = control-ref of="Hymidity"() -> (w254:refnum<vi>)
      n229 = control-ref of="Humidity Disable trip"() -> (w253:refnum<vi>)
      n230 = control-ref of="Weart Deapth"() -> (w250:refnum<vi>)
      n231 = control-ref of="Depth Reset Graph"() -> (w249:refnum<vi>)
      n232 = control-ref of="Weart"() -> (w248:refnum<vi>)
      n233 = control-ref of="Depthz"() -> (w247:refnum<vi>)
      n234 = control-ref of="Load pid"() -> (w243:refnum<vi>)
      n235 = control-ref of="Load Disable Trip"() -> (w242:refnum<vi>)
      n236 = control-ref of="Load Reset Graph"() -> (w241:refnum<vi>)
      n237 = control-ref of="BACK"() -> (w238:refnum<vi>)
      n238 = control-ref of="Depth Trip"() -> ()  [unwired: 1 out]
      n239 = control-ref of="Stroke (mm)"() -> (w326:refnum<vi>)
      n240 = control-ref of="Angle (Deg)"() -> (w325:refnum<vi>)
      n241 = control-ref of="Disc Speed (m/sec)"() -> (w322:refnum<vi>)
      n242 = control-ref of="Ball Speed (m/sec)"() -> (w321:refnum<vi>)
      n243 = control-ref of="Disc Speed (RPM)"() -> (w320:refnum<vi>)
      n244 = control-ref of="Ball Speed (RPM)"() -> (w319:refnum<vi>)
      n245 = control-ref of="Speed (m/sec)"() -> (w317:refnum<vi>)
      n246 = control-ref of="Set Speed (m/sec)"() -> (w316:refnum<vi>)
      n247 = control-ref of="Speed (RPM)"() -> (w315:refnum<vi>)
      n248 = control-ref of="Set Speed"() -> (w314:refnum<vi>)
      n249 = control-ref of="Time ( HH:MM:SS ) 2"() -> (w312:refnum<vi>)
      n250 = control-ref of="Test Duration"() -> (w311:refnum<vi>)
      n251 = control-ref of="Test Duration 4"() -> (w310:refnum<vi>)
      n252 = control-ref of="TEST CYCLE"() -> (w309:refnum<vi>)
      n253 = control-ref of="TOTAL CYCLES"() -> (w308:refnum<vi>)
      n254 = control-ref of="Set Load (N)"() -> (w307:refnum<vi>)
      n255 = control-ref of="ChamberTemp"() -> (w303:refnum<vi>)
      n256 = control-ref of="SetTmp"() -> (w302:refnum<vi>)
      n257 = control-ref of="ChamberTemp"() -> (w300:refnum<vi>)
      n258 = control-ref of="SetTmp"() -> (w299:refnum<vi>)
      n259 = control-ref of="Ambient \nTemperature"() -> (w296:refnum<vi>)
      n260 = control-ref of="Ambient\n Humidity"() -> (w294:refnum<vi>)
      n261 = control-ref of="Freq (Hz)"() -> (w293:refnum<vi>)
      n262 = control-ref of="humidity disp"() -> (w288:refnum<vi>)
      n263 = control-ref of="Set Humidity"() -> (w287:refnum<vi>)
      n264 = control-ref of="NL disp 2"() -> (w286:refnum<vi>)
      n265 = control-ref of="SD (mm)"() -> (w271:refnum<vi>)
      n266 = control-ref of="Acoustic Emission (mV)"() -> (w266:refnum<vi>)
      n267 = control-ref of="CoF Trip  2"() -> (w252:refnum<vi>)
      n268 = control-ref of="Depth Trip"() -> (w251:refnum<vi>)
      n269 = control-ref of="Depth (µm)"() -> (w246:refnum<vi>)
      n270 = control-ref of="NL Trip 2"() -> (w244:refnum<vi>)
      n271 = control-ref of="NL Display 4"() -> (w240:refnum<vi>)
      n272 = control-ref of="Trip Log"() -> (w282:refnum<vi>)
      n273 = control-ref of="COF TRIP"() -> ()  [unwired: 1 out]
      n274 = control-ref of="Friction Force (N)"() -> ()  [unwired: 1 out]
      n275 = control-ref of="FF Reset Graph"() -> ()  [unwired: 1 out]
      n276 = control-ref of="FF Disable Trip"() -> ()  [unwired: 1 out]
      n277 = control-ref of="FF TRIP"() -> ()  [unwired: 1 out]
      n278 = control-ref of="FF MAIN CHART"() -> ()  [unwired: 1 out]
      n279 = control-ref of="COF Disable Trip"() -> ()  [unwired: 1 out]
      n280 = control-ref of="COF Reset Graph"() -> ()  [unwired: 1 out]
      n281 = control-ref of="COF MAIN CHART"() -> ()  [unwired: 1 out]
      n282 = control-ref of="FF Tab"() -> ()  [unwired: 1 out]
      n283 = Bundle By Name(cluster=w330, "Main Screen.Main Screen Tab"=w328, "Main Screen.Angle and Frequency"=w327, "Main Screen.Stroke (mm)"=w326, "Main Screen.Angle (Deg)"=w325, "Main Screen.Main Speed Tab"=w324, "Main Screen.MTM MOTOR DISPLAY"=w323, "Main Screen.Disc Speed (m/sec)"=w322, "Main Screen.Ball Speed (m/sec)"=w321, "Main Screen.Disc Speed (RPM)"=w320, "Main Screen.Ball Speed (RPM)"=w319, "Main Screen.SPEED TAB"=w318, "Main Screen.Speed (m/sec)"=w317, "Main Screen.Set Speed (m/sec)"=w316, "Main Screen.Speed (RPM)"=w315, "Main Screen.Set Speed"=w314, "Main Screen.Time Tab"=w313, "Main Screen.Time ( HH:MM:SS ) 2"=w312, "Main Screen.Test Duration"=w311, "Main Screen.Test Duration 4"=w310, "Main Screen.TEST CYCLE"=w309, "Main Screen.TOTAL CYCLES"=w308, "Main Screen.Set Load (N)"=w307, "Main Screen.Temp Tabs"=w306, "Main Screen.Heater"=w305, "Main Screen.TK4 status"=w304, "Main Screen.ChamberTemp"=w303, "Main Screen.SetTmp"=w302, "Main Screen.Controller  Status"=w301, "Main Screen.ChamberTemp 2"=w300, "Main Screen.SetTmp 2"=w299, "Main Screen.Cooling"=w298, "Main Screen.Load Communication"=w297, "Main Screen.Ambient \nTemperature"=w296, "Main Screen.HumCOMStatus"=w295, "Main Screen.Ambient\n Humidity"=w294, "Main Screen.Freq (Hz)"=w293, "Main Screen.Load En"=w292, "Main Screen.NLt"=w291, "Main Screen.zNL 2"=w290, "Main Screen.Humidity On"=w289, "Main Screen.humidity disp"=w288, "Main Screen.Set Humidity"=w287, "Main Screen.NL disp 2"=w286, "Main Screen.AppLoadSeq scratch"=w285, "Main Screen.Stop Scratch"=w284, "Main Screen.ClrLog"=w283, "Main Screen.Trip Log"=w282, "Main Screen.STOP"=w281, "Main Screen.Start Test"=w280, "Main Screen.Test status"=w279, "Main Screen.AR Led"=w278, "Main Screen.Data"=w277, "Main Screen.Health"=w276, "Main Screen.Sway COM Status"=w275, "Main Screen.Heave COM Status"=w274, "Main Screen.Grp Tab"=w273, "Main Screen.Sub Graph"=w272, "Main Screen.SD (mm)"=w271, "Main Screen.Siliding distance Reset Graph"=w270, "Main Screen.SDGp"=w269, "Main Screen.Humidity Reset Graph"=w268, "Main Screen.HumrGp"=w267, "Main Screen.Acoustic Emission (mV)"=w266, "Main Screen.Aqucostic Reset Graph"=w265, "Main Screen.gACQUOS"=w264, "Main Screen.ECR RESET"=w263, "Main Screen.ECR"=w262, "Main Screen.Temperature Reset"=w261, "Main Screen.Temperature (deg c)"=w260, "Main Screen.Speed Reset Graph"=w259, "Main Screen.Speed Tab"=w258, "Main Screen.MTM DISC  SPEED"=w257, "Main Screen.MTM BALL SPEED"=w256, "Main Screen.speed mm/sec"=w255, "Main Screen.Hymidity"=w254, "Main Screen.Humidity Disable trip"=w253, "Main Screen.CoF Trip  2"=w252, "Main Screen.Depth Trip"=w251, "Main Screen.Weart Deapth"=w250, "Main Screen.Depth Reset Graph"=w249, "Main Screen.Weart"=w248, "Main Screen.Depthz"=w247, "Main Screen.Depth (µm)"=w246, "Main Screen.WearGp"=w245, "Main Screen.NL Trip 2"=w244, "Main Screen.Load pid"=w243, "Main Screen.Load Disable Trip"=w242, "Main Screen.Load Reset Graph"=w241, "Main Screen.NL Display 4"=w240, "Main Screen.Main Chart 3"=w239, "Main Screen.BACK"=w238) -> (w329:T11)
    }
    frame #9 {
      n284 = control-ref of="gFF Rot 7"() -> (w334:refnum<vi>)
      n285 = control-ref of="Ramp"() -> (w353:refnum<vi>)
      n286 = control-ref of="Dummy Run"() -> (w347:refnum<vi>)
      n287 = control-ref of="AutoTune"() -> (w345:refnum<vi>)
      n288 = control-ref of="apply load"() -> (w343:refnum<vi>)
      n289 = control-ref of="reinit 3"() -> (w341:refnum<vi>)
      n290 = control-ref of="Bypass Load"() -> (w338:refnum<vi>)
      n291 = control-ref of="PID gains out delay (microForce)"() -> (w354:refnum<vi>)
      n292 = control-ref of="output range delay"() -> (w340:refnum<vi>)
      n293 = control-ref of="PID gains out delay"() -> (w339:refnum<vi>)
      n294 = control-ref of="Ramp MulFac"() -> (w358:refnum<vi>)
      n295 = control-ref of="pulses LoadDiffRamp(2..10)"() -> (w357:refnum<vi>)
      n296 = control-ref of="PulseControlRamp(diff<=3N)"() -> (w356:refnum<vi>)
      n297 = control-ref of="SetLoadDeadband(%) Load(0-10N)"() -> (w355:refnum<vi>)
      n298 = control-ref of="Gain 2"() -> (w352:refnum<vi>)
      n299 = control-ref of="pulses LoadDiff(2..10)"() -> (w351:refnum<vi>)
      n300 = control-ref of="pulses LoadDiff(11..50)"() -> (w350:refnum<vi>)
      n301 = control-ref of="PulseControl(diff<=3N)"() -> (w349:refnum<vi>)
      n302 = control-ref of="SetLoadDeadband(%)  2"() -> (w348:refnum<vi>)
      n303 = control-ref of="Vertical load (N)"() -> (w346:refnum<vi>)
      n304 = control-ref of="Offset  3"() -> (w344:refnum<vi>)
      n305 = control-ref of="Enter ByPass Load"() -> (w342:refnum<vi>)
      n306 = control-ref of="pulsesSent"() -> (w337:refnum<vi>)
      n307 = control-ref of="pulses"() -> (w336:refnum<vi>)
      n308 = control-ref of="actpid"() -> (w335:refnum<vi>)
      n309 = control-ref of="pulses LoadDiff(21..1000)"() -> (w333:refnum<vi>)
      n310 = control-ref of="Delay"() -> (w332:refnum<vi>)
      n311 = control-ref of="deadband"() -> (w331:refnum<vi>)
      n312 = Bundle By Name(cluster=w360, "PID.Ramp MulFac"=w358, "PID.pulses LoadDiffRamp(2..10)"=w357, "PID.PulseControlRamp(diff<=3N)"=w356, "PID.SetLoadDeadband(%) Load(0-10N)"=w355, "PID.PID gains out delay (microForce)"=w354, "PID.Ramp"=w353, "PID.Gain 2"=w352, "PID.pulses LoadDiff(2..10)"=w351, "PID.pulses LoadDiff(11..50)"=w350, "PID.PulseControl(diff<=3N)"=w349, "PID.SetLoadDeadband(%)  2"=w348, "PID.Dummy Run"=w347, "PID.Vertical load (N)"=w346, "PID.AutoTune"=w345, "PID.Offset 3"=w344, "PID.apply load"=w343, "PID.Enter ByPass Load"=w342, "PID.reinit 3"=w341, "PID.output range delay"=w340, "PID.PID gains out delay"=w339, "PID.Bypass Load"=w338, "PID.pulsesSent"=w337, "PID.pulses"=w336, "PID.actpid"=w335, "PID.gFF Rot"=w334, "PID.pulses LoadDiff(21..1000)"=w333, "PID.Delay"=w332, "PID.deadband"=w331) -> (w359:T11)
    }
    frame #10 {
      n313 = control-ref of="Tab Control 3"() -> (w404:refnum<vi>)
      n314 = control-ref of="Tab Control 19"() -> (w403:refnum<vi>)
      n315 = control-ref of="Tab Control 5"() -> (w364:refnum<vi>)
      n316 = control-ref of="Tab Control 14"() -> (w363:refnum<vi>)
      n317 = control-ref of="Tab Control 26"() -> (w362:refnum<vi>)
      n318 = control-ref of="Re-initilaize"() -> (w401:refnum<vi>)
      n319 = control-ref of="Filter ON/OFF"() -> (w400:refnum<vi>)
      n320 = control-ref of="Apply Filter (FF)"() -> (w396:refnum<vi>)
      n321 = control-ref of="Apply Filter (Load)"() -> (w394:refnum<vi>)
      n322 = control-ref of="SAVE  2"() -> (w389:refnum<vi>)
      n323 = control-ref of="Enter Distance"() -> (w388:refnum<vi>)
      n324 = control-ref of="AE"() -> (w361:refnum<vi>)
      n325 = control-ref of="SAMPLES"() -> (w402:refnum<vi>)
      n326 = control-ref of="TracHomeSurgeOffsetCounts 10MM"() -> (w399:refnum<vi>)
      n327 = control-ref of="TracHomeSwayOffsetCounts 10MM"() -> (w398:refnum<vi>)
      n328 = control-ref of="Acoustic Emission:"() -> (w397:refnum<vi>)
      n329 = control-ref of="Filter% 2"() -> (w395:refnum<vi>)
      n330 = control-ref of="Filter%"() -> (w393:refnum<vi>)
      n331 = control-ref of="Sway distance (mm)"() -> (w392:refnum<vi>)
      n332 = control-ref of="Surge distance (mm)"() -> (w391:refnum<vi>)
      n333 = control-ref of="DataSavingLoopDelay(ms)"() -> (w390:refnum<vi>)
      n334 = control-ref of="Sway Counts:"() -> (w387:refnum<vi>)
      n335 = control-ref of="Distance (mm): 3"() -> (w386:refnum<vi>)
      n336 = control-ref of="Surge Counts:"() -> (w385:refnum<vi>)
      n337 = control-ref of="Distance (mm): 2"() -> (w384:refnum<vi>)
      n338 = control-ref of="Distance (mm):"() -> (w383:refnum<vi>)
      n339 = control-ref of="Heave Counts:"() -> (w382:refnum<vi>)
      n340 = control-ref of="LRMHomeSurgeOffsetCounts"() -> (w381:refnum<vi>)
      n341 = control-ref of="LRMHomeSwayOffsetCounts"() -> (w380:refnum<vi>)
      n342 = control-ref of="TracHomeSurgeOffsetCounts 20MM"() -> (w379:refnum<vi>)
      n343 = control-ref of="TracHomeSwayOffsetCounts 20MM"() -> (w378:refnum<vi>)
      n344 = control-ref of="RotHomeSwayOffsetCounts"() -> (w377:refnum<vi>)
      n345 = control-ref of="RotHomeSurgeOffsetCounts"() -> (w376:refnum<vi>)
      n346 = control-ref of="Heave distance"() -> (w375:refnum<vi>)
      n347 = control-ref of="Zmm"() -> (w374:refnum<vi>)
      n348 = control-ref of="Heave Pulses/mm"() -> (w373:refnum<vi>)
      n349 = control-ref of="Surge Pulses/mm"() -> (w372:refnum<vi>)
      n350 = control-ref of="Sway Pulses/mm"() -> (w371:refnum<vi>)
      n351 = control-ref of="Heave Pitch"() -> (w370:refnum<vi>)
      n352 = control-ref of="Surge Pitch"() -> (w369:refnum<vi>)
      n353 = control-ref of="Sway Pitch"() -> (w368:refnum<vi>)
      n354 = control-ref of="Heave PPR"() -> (w367:refnum<vi>)
      n355 = control-ref of="Surge PPR"() -> (w366:refnum<vi>)
      n356 = control-ref of="Sway PPR"() -> (w365:refnum<vi>)
      n357 = Bundle By Name(cluster=w406, "Config Parameters.Tab Control 3"=w404, "Config Parameters.Tab Control 19"=w403, "Config Parameters.SAMPLES"=w402, "Config Parameters.Re-initilaize"=w401, "Config Parameters.Filter ON/OFF"=w400, "Config Parameters.TracHomeSurgeOffsetCounts 10MM"=w399, "Config Parameters.TracHomeSwayOffsetCounts 10MM"=w398, "Config Parameters.Acoustic Emission:"=w397, "Config Parameters.Apply Filter (FF)"=w396, "Config Parameters.Filter% 2"=w395, "Config Parameters.Apply Filter (Load)"=w394, "Config Parameters.Filter%"=w393, "Config Parameters.Sway distance (mm)"=w392, "Config Parameters.Surge distance (mm)"=w391, "Config Parameters.DataSavingLoopDelay(ms)"=w390, "Config Parameters.SAVE 2"=w389, "Config Parameters.Enter Distance"=w388, "Config Parameters.Sway Counts:"=w387, "Config Parameters.Distance (mm): 3"=w386, "Config Parameters.Surge Counts:"=w385, "Config Parameters.Distance (mm): 2"=w384, "Config Parameters.Distance (mm):"=w383, "Config Parameters.Heave Counts:"=w382, "Config Parameters.LRMHomeSurgeOffsetCounts"=w381, "Config Parameters.LRMHomeSwayOffsetCounts"=w380, "Config Parameters.TracHomeSurgeOffsetCounts 20MM"=w379, "Config Parameters.TracHomeSwayOffsetCounts 20MM"=w378, "Config Parameters.RotHomeSwayOffsetCounts"=w377, "Config Parameters.RotHomeSurgeOffsetCounts"=w376, "Config Parameters.Heave distance"=w375, "Config Parameters.Zmm"=w374, "Config Parameters.Heave Pulses/mm"=w373, "Config Parameters.Surge Pulses/mm"=w372, "Config Parameters.Sway Pulses/mm"=w371, "Config Parameters.Heave Pitch"=w370, "Config Parameters.Surge Pitch"=w369, "Config Parameters.Sway Pitch"=w368, "Config Parameters.Heave PPR"=w367, "Config Parameters.Surge PPR"=w366, "Config Parameters.Sway PPR"=w365, "Config Parameters.Tab Control 5"=w364, "Config Parameters.Tab Control 14"=w363, "Config Parameters.Tab Control 26"=w362, "Config Parameters.AE"=w361) -> (w405:T11)
    }
    frame #11 {
      n358 = control-ref of="Mx"() -> (w435:refnum<vi>)
      n359 = control-ref of="My"() -> (w434:refnum<vi>)
      n360 = control-ref of="Mz"() -> (w433:refnum<vi>)
      n361 = control-ref of="Fx(N)"() -> (w432:refnum<vi>)
      n362 = control-ref of="Fy(N)"() -> (w431:refnum<vi>)
      n363 = control-ref of="Fz(N)"() -> (w430:refnum<vi>)
      n364 = control-ref of="ClearAll"() -> (w440:refnum<vi>)
      n365 = control-ref of="ZeroAll"() -> (w429:refnum<vi>)
      n366 = control-ref of="delete Handle"() -> (w419:refnum<vi>)
      n367 = control-ref of="Create Handle"() -> (w418:refnum<vi>)
      n368 = control-ref of="stop 6"() -> (w415:refnum<vi>)
      n369 = control-ref of="running_flag"() -> (w414:refnum<vi>)
      n370 = control-ref of="Save Dwell"() -> (w436:refnum<vi>)
      n371 = control-ref of="Acq Delay (ms)"() -> (w428:refnum<vi>)
      n372 = control-ref of="Burst Delay (ms)"() -> (w427:refnum<vi>)
      n373 = control-ref of="SN"() -> (w425:refnum<vi>)
      n374 = control-ref of="Port"() -> (w422:refnum<vi>)
      n375 = control-ref of="ft_udp_handle"() -> (w413:refnum<vi>)
      n376 = control-ref of="get-data-return"() -> (w412:refnum<vi>)
      n377 = control-ref of="get-range-return"() -> (w411:refnum<vi>)
      n378 = control-ref of="zero-return"() -> (w410:refnum<vi>)
      n379 = control-ref of="filter-return"() -> (w409:refnum<vi>)
      n380 = control-ref of="initial-return"() -> (w408:refnum<vi>)
      n381 = control-ref of="deleteHandle-result"() -> (w407:refnum<vi>)
      n382 = control-ref of="model"() -> (w426:refnum<vi>)
      n383 = control-ref of="Sensor IP"() -> (w423:refnum<vi>)
      n384 = control-ref of="Mz(Nm)"() -> (w439:refnum<vi>)
      n385 = control-ref of="My(Nm)"() -> (w438:refnum<vi>)
      n386 = control-ref of="Mx(Nm)"() -> (w437:refnum<vi>)
      n387 = control-ref of="FFx(N)"() -> (w424:refnum<vi>)
      n388 = control-ref of="FFy(N)"() -> (w421:refnum<vi>)
      n389 = control-ref of="Load(N)"() -> (w420:refnum<vi>)
      n390 = control-ref of="ft_data"() -> (w417:refnum<vi>)
      n391 = control-ref of="ft_range"() -> (w416:refnum<vi>)
      n392 = Bundle By Name(cluster=w442, "Loading Com Port.ClearAll"=w440, "Loading Com Port.Mz(Nm)"=w439, "Loading Com Port.My(Nm)"=w438, "Loading Com Port.Mx(Nm)"=w437, "Loading Com Port.Save Dwell"=w436, "Loading Com Port.Mx"=w435, "Loading Com Port.My"=w434, "Loading Com Port.Mz"=w433, "Loading Com Port.Fx(N)"=w432, "Loading Com Port.Fy(N)"=w431, "Loading Com Port.Fz(N)"=w430, "Loading Com Port.ZeroAll"=w429, "Loading Com Port.Acq Delay (ms)"=w428, "Loading Com Port.Burst Delay (ms)"=w427, "Loading Com Port.model"=w426, "Loading Com Port.SN"=w425, "Loading Com Port.FFx(N)"=w424, "Loading Com Port.Sensor IP"=w423, "Loading Com Port.Port"=w422, "Loading Com Port.FFy(N)"=w421, "Loading Com Port.Load(N)"=w420, "Loading Com Port.delete Handle"=w419, "Loading Com Port.Create Handle"=w418, "Loading Com Port.ft_data"=w417, "Loading Com Port.ft_range"=w416, "Loading Com Port.stop 6"=w415, "Loading Com Port.running_flag"=w414, "Loading Com Port.ft_udp_handle"=w413, "Loading Com Port.get-data-return"=w412, "Loading Com Port.get-range-return"=w411, "Loading Com Port.zero-return"=w410, "Loading Com Port.filter-return"=w409, "Loading Com Port.initial-return"=w408, "Loading Com Port.deleteHandle-result"=w407) -> (w441:T11)
    }
  }
  n393 = call <userlib>:"Fit VI window to Largest Dec.vi"() -> ("error out"=w27:errorcluster, "dup VI Ref"=w24:refnum<vi>)  [unwired: 6 in]
  n394 = invoke on="Invoke Node" class="VI" method="FP.Run-Time Position.Maximized"(reference=w24, error in=w27) -> (error out=w26:errorcluster)  [unwired: 2 in, 3 out]
  n395 = call <vilib>:"Clear Errors.vi"("error in (no error)"=w26) -> ("error out"=w25:errorcluster)  [unwired: 5 in, 1 out]
  n396 = control-ref of="This VI"() -> (w30:refnum<vi>)
  n397 = invoke on="Invoke Node" class="VI" method="Default Vals.Reinit All"(reference=w30, error in=w25) -> (reference out=w28:refnum<vi>, error out=w29:errorcluster)  [unwired: 1 in, 1 out]
  n398 = Close Reference(reference=w28, error in (no error)=w29) -> (error out=w23:errorcluster)
  n399 = call "Create User Event - Stop.vi"("error in (no error)"=w23) -> ("error out"=w7:errorcluster, "User Event - Stop"=w8:refnum<user-event>)  [unwired: 9 in]
  n400 = call "main screen queue out Unitest.vi"("error in (no error)"=w7) -> ("error out"=w50:errorcluster, "output Queue"=w22:T12)  [unwired: 9 in]
  n401 = Unbundle By Name(w22) -> ("UI Loop"=w48:refnum<queue>)
  n402 = Unbundle By Name(w22) -> ("LOAD COM LOOP"=w20:refnum<queue>)
  n403 = Unbundle By Name(w22) -> ("SWAY MOTOR COM LOOP"=w19:refnum<queue>)
  n404 = Unbundle By Name(w22) -> ("HEAVE MOTOR COM LOOP"=w17:refnum<queue>)
  n405 = Unbundle By Name(w22) -> ("TEMPERATURE COM LOOP"=w16:refnum<queue>)
  n406 = Unbundle By Name(w22) -> ("RAMP MOTOR COM LOOP"=w13:refnum<queue>)
  n407 = Unbundle By Name(w22) -> ("ECR PORT"=w12:refnum<queue>)
  n408 = Unbundle By Name(w22) -> ("HUMIDITY COM PORT"=w11:refnum<queue>)
  n409 = Unbundle By Name(w22) -> ("PROGRAM LOOP"=w10:refnum<queue>)
  n410 = Unbundle By Name(w22) -> ("MONITOR LOOP"=w6:refnum<queue>)
  n411 = Unbundle By Name(w22) -> ("LOAD PID"=w5:refnum<queue>)
  n412 = Unbundle By Name(w22) -> ("REPORT"=w4:refnum<queue>)
  n413 = register-events(w8) -> (reference out=w42:refnum<event-registration>, error out=w40:errorcluster)  [unwired: 2 in]
  n414 = Merge Errors(w40, w50) -> (w41:errorcluster)
  n415 = while {
    tunnel: w48 -> [w450]
    shift-right: [w448] -> w45
    shift-left: w42 -> [w449]
    tunnel: [w444] -> w43
    stop <- w446 stop-if-true
    # "Event Handling Loop"
    n416 = event shown="[23] \"SNext\": Value Change" {
      selector: w449 -> [_ _ _ _ _ _ _ _ _ _ _ _ _ _ _ _ _ _ _ _ _ _ _ _ _ _ _]
      dyn-events: [_ _ _ _ _ _ _ _ _ _ _ _ _ _ _ _ _ _ _ _ _ _ _ _ _ _ _] -> w448
      timeout: 100 -> [_ _ _ _ _ _ _ _ _ _ _ _ _ _ _ _ _ _ _ _ _ _ _ _ _ _ _]
      tunnel: [_ _ _ _ _ _ _ _ _ _ _ _ _ _ _ _ _ _ _ _ _ _ _ _ _ _ TRUE ("Discard?")] -> w446
      tunnel: w450 -> [w455 w459 w464 w469 w474 w479 w484 w489 w494 w499 w504 w509 w514 w519 w524 w529 w534 w539 w544 w549 w554 w559 w564 w569 w572 w577 w579]
      tunnel: [w454 w457 w462 w467 w472 w477 w482 w487 w492 w497 w502 w507 w512 w517 w522 w527 w532 w537 w542 w547 w552 w557 w562 w567 _ w576 _] -> w447
      tunnel: [w453 w458 w463 w468 w473 w478 w483 w488 w493 w498 w503 w508 w513 w518 w523 w528 w533 w538 w543 w548 w553 w558 w563 w568 w572 w575 w579] -> w445
      event Panel Close? {
        n417 = event-data() -> ()  [unwired: 1 in, 1 out]
        n418 = call-poly "Enqueue Message.vi"("Priority Message? (F)"=TRUE, "Message"="Confirm Quit", "Message Queue"=w455) -> ("error out"=w454:errorcluster, "dup Message Queue"=w453:refnum<queue>)  [unwired: 7 in]
        n419 = event-data("Discard?"=TRUE) -> ()  [unwired: 1 in, 1 out]
      }
      event Timeout {
        n420 = event-data() -> ()  [unwired: 1 in, 1 out]
        n421 = call-poly "Enqueue Message.vi"("Priority Message? (F)"=TRUE, "Message"="Time Out", "Message Queue"=w459) -> ("error out"=w457:errorcluster, "dup Message Queue"=w458:refnum<queue>)  [unwired: 7 in]
      }
      event "SAVE  2": Value Change {
        n422 = event-data() -> ()  [unwired: 1 in, 1 out]
        n423 = call-poly "Enqueue Message.vi"("Priority Message? (F)"=TRUE, "Message"="Service Save", "Message Queue"=w464) -> ("error out"=w462:errorcluster, "dup Message Queue"=w463:refnum<queue>)  [unwired: 7 in]
      }
      event "Home": Value Change {
        n424 = event-data() -> ()  [unwired: 1 in, 1 out]
        n425 = call-poly "Enqueue Message.vi"("Priority Message? (F)"=TRUE, "Message"="HOME", "Message Queue"=w469) -> ("error out"=w467:errorcluster, "dup Message Queue"=w468:refnum<queue>)  [unwired: 7 in]
      }
      event "Platform Settings": Value Change {
        n426 = event-data() -> ()  [unwired: 1 in, 1 out]
        n427 = call-poly "Enqueue Message.vi"("Priority Message? (F)"=TRUE, "Message"="Platform Setting", "Message Queue"=w474) -> ("error out"=w472:errorcluster, "dup Message Queue"=w473:refnum<queue>)  [unwired: 7 in]
      }
      event "Configure": Value Change {
        n428 = event-data() -> ()  [unwired: 1 in, 1 out]
        n429 = call-poly "Enqueue Message.vi"("Priority Message? (F)"=TRUE, "Message"="Configure", "Message Queue"=w479) -> ("error out"=w477:errorcluster, "dup Message Queue"=w478:refnum<queue>)  [unwired: 7 in]
      }
      event "Analysis": Value Change {
        n430 = event-data() -> ()  [unwired: 1 in, 1 out]
        n431 = call-poly "Enqueue Message.vi"("Priority Message? (F)"=TRUE, "Message"="Analysis", "Message Queue"=w484) -> ("error out"=w482:errorcluster, "dup Message Queue"=w483:refnum<queue>)  [unwired: 7 in]
      }
      event "service 2": Value Change {
        n432 = event-data() -> ()  [unwired: 1 in, 1 out]
        n433 = call-poly "Enqueue Message.vi"("Priority Message? (F)"=TRUE, "Message"="service 2", "Message Queue"=w489) -> ("error out"=w487:errorcluster, "dup Message Queue"=w488:refnum<queue>)  [unwired: 7 in]
      }
      event "Auto": Value Change {
        n434 = event-data() -> ()  [unwired: 1 in, 1 out]
        n435 = call-poly "Enqueue Message.vi"("Priority Message? (F)"=TRUE, "Message"="Auto", "Message Queue"=w494) -> ("error out"=w492:errorcluster, "dup Message Queue"=w493:refnum<queue>)  [unwired: 7 in]
      }
      event "Select Load Head": Value Change {
        n436 = event-data() -> ()  [unwired: 1 in, 1 out]
        n437 = call-poly "Enqueue Message.vi"("Priority Message? (F)"=TRUE, "Message"="Select Load Head", "Message Queue"=w499) -> ("error out"=w497:errorcluster, "dup Message Queue"=w498:refnum<queue>)  [unwired: 7 in]
      }
      event "com 3": Value Change {
        n438 = event-data() -> ()  [unwired: 1 in, 1 out]
        n439 = call-poly "Enqueue Message.vi"("Priority Message? (F)"=TRUE, "Message"="com 3", "Message Queue"=w504) -> ("error out"=w502:errorcluster, "dup Message Queue"=w503:refnum<queue>)  [unwired: 7 in]
      }
      event "Loading Mode": Value Change {
        n440 = event-data() -> ()  [unwired: 1 in, 1 out]
        n441 = call-poly "Enqueue Message.vi"("Priority Message? (F)"=TRUE, "Message"="Loading Mode", "Message Queue"=w509) -> ("error out"=w507:errorcluster, "dup Message Queue"=w508:refnum<queue>)  [unwired: 7 in]
      }
      event "SSP 0.3": Value Change {
        n442 = event-data() -> ()  [unwired: 1 in, 1 out]
        n443 = call-poly "Enqueue Message.vi"("Priority Message? (F)"=TRUE, "Message"="SSP 0.3", "Message Queue"=w514) -> ("error out"=w512:errorcluster, "dup Message Queue"=w513:refnum<queue>)  [unwired: 7 in]
      }
      event "SSP 0.5": Value Change {
        n444 = event-data() -> ()  [unwired: 1 in, 1 out]
        n445 = call-poly "Enqueue Message.vi"("Priority Message? (F)"=TRUE, "Message"="SSP 0.5", "Message Queue"=w519) -> ("error out"=w517:errorcluster, "dup Message Queue"=w518:refnum<queue>)  [unwired: 7 in]
      }
      event "SSP 0.75": Value Change {
        n446 = event-data() -> ()  [unwired: 1 in, 1 out]
        n447 = call-poly "Enqueue Message.vi"("Priority Message? (F)"=TRUE, "Message"="SSP 0.75", "Message Queue"=w524) -> ("error out"=w522:errorcluster, "dup Message Queue"=w523:refnum<queue>)  [unwired: 7 in]
      }
      event "LHBack": Value Change {
        n448 = event-data() -> ()  [unwired: 1 in, 1 out]
        n449 = call-poly "Enqueue Message.vi"("Priority Message? (F)"=TRUE, "Message"="LHBack", "Message Queue"=w529) -> ("error out"=w527:errorcluster, "dup Message Queue"=w528:refnum<queue>)  [unwired: 7 in]
      }
      event "LHNext": Value Change {
        n450 = event-data() -> ()  [unwired: 1 in, 1 out]
        n451 = call-poly "Enqueue Message.vi"("Priority Message? (F)"=TRUE, "Message"="LHNext", "Message Queue"=w534) -> ("error out"=w532:errorcluster, "dup Message Queue"=w533:refnum<queue>)  [unwired: 7 in]
      }
      event "Rot Ver": Value Change {
        n452 = event-data() -> ()  [unwired: 1 in, 1 out]
        n453 = call-poly "Enqueue Message.vi"("Priority Message? (F)"=TRUE, "Message"="Rot Ver", "Message Queue"=w539) -> ("error out"=w537:errorcluster, "dup Message Queue"=w538:refnum<queue>)  [unwired: 7 in]
      }
      event "Scratch": Value Change {
        n454 = event-data() -> ()  [unwired: 1 in, 1 out]
        n455 = call-poly "Enqueue Message.vi"("Priority Message? (F)"=TRUE, "Message"="Scratch", "Message Queue"=w544) -> ("error out"=w542:errorcluster, "dup Message Queue"=w543:refnum<queue>)  [unwired: 7 in]
      }
      event "Motion Mode:": Value Change {
        n456 = event-data() -> ()  [unwired: 1 in, 1 out]
        n457 = call-poly "Enqueue Message.vi"("Priority Message? (F)"=TRUE, "Message"="Motion Mode:", "Message Queue"=w549) -> ("error out"=w547:errorcluster, "dup Message Queue"=w548:refnum<queue>)  [unwired: 7 in]
      }
      event "MMBack": Value Change {
        n458 = event-data() -> ()  [unwired: 1 in, 1 out]
        n459 = call-poly "Enqueue Message.vi"("Priority Message? (F)"=TRUE, "Message"="MMBack", "Message Queue"=w554) -> ("error out"=w552:errorcluster, "dup Message Queue"=w553:refnum<queue>)  [unwired: 7 in]
      }
      event "MMNext": Value Change {
        n460 = event-data() -> ()  [unwired: 1 in, 1 out]
        n461 = call-poly "Enqueue Message.vi"("Priority Message? (F)"=TRUE, "Message"="MMNext", "Message Queue"=w559) -> ("error out"=w557:errorcluster, "dup Message Queue"=w558:refnum<queue>)  [unwired: 7 in]
      }
      event "APBack": Value Change {
        n462 = event-data() -> ()  [unwired: 1 in, 1 out]
        n463 = call-poly "Enqueue Message.vi"("Priority Message? (F)"=TRUE, "Message"="APBack", "Message Queue"=w564) -> ("error out"=w562:errorcluster, "dup Message Queue"=w563:refnum<queue>)  [unwired: 7 in]
      }
      event "SNext": Value Change {
        n464 = event-data() -> ()  [unwired: 1 in, 1 out]
        n465 = call-poly "Enqueue Message.vi"("Priority Message? (F)"=TRUE, "Message"="SNext", "Message Queue"=w569) -> ("error out"=w567:errorcluster, "dup Message Queue"=w568:refnum<queue>)  [unwired: 7 in]
      }
      event Application Instance Close {
        # "#CodeRecommended - When a project closes, all VIs within that project are aborted and leave memory. However, any code placed in this event frame is guaranteed to run to completion, so add any cleanup code that absolutely must happen here."
        n466 = event-data() -> ()  [unwired: 1 in, 1 out]
      }
      event "EXIT": Value Change {
        n467 = event-data() -> ()  [unwired: 1 in, 1 out]
        n468 = call-poly "Enqueue Message.vi"("Priority Message? (F)"=TRUE, "Message"="Exit", "Message Queue"=w577) -> ("error out"=w576:errorcluster, "dup Message Queue"=w575:refnum<queue>)  [unwired: 7 in]
      }
      event User Event {
        # "The Message Handling Loop processed an \"Exit\" message, which fired this event to stop the Event Handling Loop."
        n469 = event-data() -> ()  [unwired: 1 in, 1 out]
      }
    }
    n470 = call "LAB-IQ Error Handler - Event Handling Loop.vi"("error in (no error)"=w447, "Message Queue"=w445) -> ("dup error in"=w444:errorcluster)  [unwired: 8 in, 1 out]
  }
  n471 = while {
    tunnel: w48 -> [w594]
    shift-right: [w601] -> _
    shift-left: w9 -> [w602]
    tunnel: w8 -> [w599]
    tunnel: w41 -> [w598]
    tunnel: [w592] -> w49
    tunnel: w20 -> [w590]
    tunnel: w19 -> [w589]
    tunnel: w17 -> [w588]
    tunnel: w16 -> [w587]
    tunnel: w13 -> [w586]
    tunnel: w12 -> [w585]
    tunnel: w11 -> [w584]
    tunnel: w10 -> [w583]
    tunnel: w6 -> [w582]
    tunnel: w5 -> [w581]
    tunnel: w4 -> [w580]
    stop <- w600 stop-if-true
    # "Message Handling Loop"
    n472 = call "Dequeue Message.vi"("error in (no error)"=w598, "Message Queue"=w594) -> ("error out"=w597:errorcluster, "Message Data"=w595:variant, "Message"=w596:string, "dup Message Queue"=w593:refnum<queue>)  [unwired: 6 in]
    n473 = case "Message Cases" shown="\"SNext\"" w596 {
      selector: w596 -> [_ _ _ _ _ _ _ _ _ _ _ _ _ _ _ _ _ _ _ _ _ _ _ _ _ _ _ _ w1295]
      tunnel: w593 -> [_ w611 _ _ _ _ _ _ _ _ _ _ _ _ _ _ _ _ _ _ _ _ _ _ _ _ w1282 w1294 _]
      tunnel: w597 -> [w604 w613 w638 w642 w663 w680 w697 w714 w735 w747 w797 w801 w806 w871 w897 w923 w954 w966 w1014 w1034 w1123 w1200 w1239 w1251 w1263 w1279 w1286 w1287 _]
      tunnel: [w604 w610 w627 w643 w658 w675 w692 w709 w730 w739 w775 w799 w810 w867 w893 w919 w955 w967 w978 w1025 w1114 w1199 w1238 w1250 w1262 w1273 w1284 w1290 w1296] -> w591
      tunnel: w602 -> [w603 w606 w639 w641 w649 w666 w683 w700 w718 w737 w752 w800 w805 w869 w895 w921 w945 w957 w969 w1018 w1106 w1194 w1237 w1249 w1261 w1278 w1285 w1293 w1297]
      tunnel: [w603 w606 w639 w641 w649 w666 w683 w700 w718 w737 w752 w800 w805 w869 w895 w921 w945 w957 w969 w1018 w1106 w1194 w1237 w1249 w1261 w1278 w1285 w1293 w1297] -> w601
      tunnel: [_ _ _ _ _ _ _ _ _ _ _ _ _ _ _ _ _ _ _ _ _ _ _ _ _ _ _ TRUE _] -> w600
      tunnel: w595 -> [_ _ _ _ _ _ _ _ _ _ _ _ _ _ _ _ _ _ _ _ _ _ _ _ _ w1277 _ _ _]
      tunnel: w599 -> [_ _ _ _ _ _ _ _ _ _ _ _ _ _ _ _ _ _ _ _ _ _ _ _ _ _ _ w1289 _]
      tunnel: w590 -> [_ _ w625 _ _ _ _ _ _ _ _ _ _ _ _ _ _ _ _ _ _ _ _ _ _ _ _ _ _]
      tunnel: w589 -> [_ _ w624 _ _ _ _ _ _ _ _ _ _ _ _ _ _ _ _ _ _ _ _ _ _ _ _ _ _]
      tunnel: w588 -> [_ _ w623 _ _ _ _ _ _ _ _ _ _ _ _ _ _ _ _ _ _ _ _ _ _ _ _ _ _]
      tunnel: w587 -> [_ _ w622 _ _ _ _ _ _ _ _ _ _ _ _ _ _ _ _ _ _ _ _ _ _ _ _ _ _]
      tunnel: w586 -> [_ _ w621 _ _ _ _ _ _ _ _ _ _ _ _ _ _ _ _ _ _ _ _ _ _ _ _ _ _]
      tunnel: w585 -> [_ _ w620 _ _ _ _ _ _ _ _ _ _ _ _ _ _ _ _ _ _ _ _ _ _ _ _ _ _]
      tunnel: w584 -> [_ _ w619 _ _ _ _ _ _ _ _ _ _ _ _ _ _ _ _ _ _ _ _ _ _ _ _ _ _]
      tunnel: w583 -> [_ _ w618 _ _ _ _ _ _ _ _ _ _ _ _ _ _ _ _ _ _ _ _ _ _ _ _ _ _]
      tunnel: w582 -> [_ _ w617 _ _ _ _ _ _ _ _ _ _ _ _ _ _ _ _ _ _ _ _ _ _ _ _ _ _]
      tunnel: w581 -> [_ _ w616 _ _ _ _ _ _ _ _ _ _ _ _ _ _ _ _ _ _ _ _ _ _ _ _ _ _]
      tunnel: w580 -> [_ _ w615 _ _ _ _ _ _ _ _ _ _ _ _ _ _ _ _ _ _ _ _ _ _ _ _ _ _]
      frame "Time Out" {
      }
      frame "init" {
        # "Initialize - All initialization work should take place in this message, since other loops can potentially enqueue messages that execute immediately after this one."
        n474 = call-poly "Enqueue Message.vi"("error in (no error)"=w613, "Message"="Init Other Loop", "Message Queue"=w611) -> ("error out"=w614:errorcluster)  [unwired: 7 in, 1 out]
        n475 = call "Read Config Unitest.vi"("error in (no error)"=w614, "main ref"=w606) -> ("error out"=w609:errorcluster)  [unwired: 9 in]
        n476 = call "Encrypt file path creation.vi"("error in (no error)"=w609) -> ("error out"=w608:errorcluster, "File Path"=w607:path)  [unwired: 9 in]
        n477 = call "DATA ENCRYPT STRING FILE WRITE.vi"("file path (dialog if empty)"=w607, "error in (no error)"=w608, "User Action"="System Booted", "main ref"=w606) -> ("error out"=w610:errorcluster)  [unwired: 5 in, 1 out]
      }
      frame "Init Other Loop" {
        w626 = "Init" ("Message")
        n478 = call-poly "Enqueue Message.vi"("error in (no error)"=w638, "Message"=w626, "Message Queue"=w625) -> ("error out"=w637:errorcluster)  [unwired: 7 in, 1 out]
        n479 = call-poly "Enqueue Message.vi"("error in (no error)"=w637, "Message"=w626, "Message Queue"=w624) -> ("error out"=w636:errorcluster)  [unwired: 7 in, 1 out]
        n480 = call-poly "Enqueue Message.vi"("error in (no error)"=w636, "Message"=w626, "Message Queue"=w623) -> ("error out"=w635:errorcluster)  [unwired: 7 in, 1 out]
        n481 = call-poly "Enqueue Message.vi"("error in (no error)"=w635, "Message"=w626, "Message Queue"=w622) -> ("error out"=w634:errorcluster)  [unwired: 7 in, 1 out]
        n482 = call-poly "Enqueue Message.vi"("error in (no error)"=w634, "Message"=w626, "Message Queue"=w621) -> ("error out"=w633:errorcluster)  [unwired: 7 in, 1 out]
        n483 = call-poly "Enqueue Message.vi"("error in (no error)"=w633, "Message"=w626, "Message Queue"=w620) -> ("error out"=w632:errorcluster)  [unwired: 7 in, 1 out]
        n484 = call-poly "Enqueue Message.vi"("error in (no error)"=w632, "Message"=w626, "Message Queue"=w619) -> ("error out"=w631:errorcluster)  [unwired: 7 in, 1 out]
        n485 = call-poly "Enqueue Message.vi"("error in (no error)"=w631, "Message"=w626, "Message Queue"=w618) -> ("error out"=w630:errorcluster)  [unwired: 7 in, 1 out]
        n486 = call-poly "Enqueue Message.vi"("error in (no error)"=w630, "Message"=w626, "Message Queue"=w617) -> ("error out"=w629:errorcluster)  [unwired: 7 in, 1 out]
        n487 = call-poly "Enqueue Message.vi"("error in (no error)"=w629, "Message"=w626, "Message Queue"=w616) -> ("error out"=w628:errorcluster)  [unwired: 7 in, 1 out]
        n488 = call-poly "Enqueue Message.vi"("error in (no error)"=w628, "Message"=w626, "Message Queue"=w615) -> ("error out"=w627:errorcluster)  [unwired: 7 in, 1 out]
      }
      frame "Service Save" {
        n489 = call "Write Config Unitest.vi"("error in (no error)"=w642, "main ref"=w641) -> ("error out"=w647:errorcluster)  [unwired: 9 in]
        n490 = call "Stall Data Flow.vim"("value in"=w647, "milliseconds to wait"=u32 2000) -> ("value out"=w646:errorcluster)  [unwired: 1 out]
        n491 = call "Read Config Unitest.vi"("error in (no error)"=w646, "main ref"=w641) -> ("error out"=w644:errorcluster)  [unwired: 9 in]
        n492 = call "DATA ENCRYPT STRING FILE WRITE.vi"("error in (no error)"=w644, "User Action"="Service Parameter Saved", "main ref"=w641) -> ("error out"=w643:errorcluster)  [unwired: 6 in, 1 out]
      }
      frame "HOME" {
        n493 = call "DATA ENCRYPT STRING FILE WRITE.vi"("error in (no error)"=w663, "User Action"="User Pressed Home", "main ref"=w649) -> ("error out"=w659:errorcluster)  [unwired: 6 in, 1 out]
        n494 = Unbundle By Name(w649) -> ("Main Home Screen.MainPage"=w654:refnum<vi>)
        n495 = Unbundle By Name(w649) -> ("Main Home Screen.Home"=w662:refnum<vi>)
        n496 = Unbundle By Name(w649) -> ("Main Home Screen.GUI"=w652:refnum<vi>)
        n497 = property class="Bool (strict)"(reference=w662, error in=w659, "Value"=FALSE) -> (reference out=w660:refnum<vi>, error out=w661:errorcluster)
        n498 = property class="TabCtl (strict)"(reference=w654, "Value"=T5."HOME") -> (reference out=w656:refnum<vi>, error out=w655:errorcluster)  [unwired: 1 in]
        n499 = property class="TabCtl (strict)"(reference=w652, "Value"=T4."Setup") -> (reference out=w650:refnum<vi>, error out=w651:errorcluster)  [unwired: 1 in]
        n500 = Close Reference(reference=w660, error in (no error)=w661) -> (error out=w658:errorcluster)
        n501 = Close Reference(reference=w656, error in (no error)=w655) -> ()  [unwired: 1 out]
        n502 = Close Reference(reference=w650, error in (no error)=w651) -> ()  [unwired: 1 out]
      }
      frame "Platform Setting" {
        n503 = call "DATA ENCRYPT STRING FILE WRITE.vi"("error in (no error)"=w680, "User Action"="User Pressed Platform Setting", "main ref"=w666) -> ("error out"=w676:errorcluster)  [unwired: 6 in, 1 out]
        n504 = Unbundle By Name(w666) -> ("Main Home Screen.Platform Settings"=w679:refnum<vi>)
        n505 = Unbundle By Name(w666) -> ("Main Home Screen.MainPage"=w671:refnum<vi>)
        n506 = Unbundle By Name(w666) -> ("Main Home Screen.GUI"=w669:refnum<vi>)
        n507 = property class="TabCtl (strict)"(reference=w671, "Value"=T5."PlatformSetting") -> (reference out=w673:refnum<vi>, error out=w672:errorcluster)  [unwired: 1 in]
        n508 = property class="TabCtl (strict)"(reference=w669, "Value"=T4."Setup") -> (reference out=w667:refnum<vi>, error out=w668:errorcluster)  [unwired: 1 in]
        n509 = property class="Bool (strict)"(reference=w679, error in=w676, "Value"=FALSE) -> (reference out=w677:refnum<vi>, error out=w678:errorcluster)
        n510 = Close Reference(reference=w673, error in (no error)=w672) -> ()  [unwired: 1 out]
        n511 = Close Reference(reference=w667, error in (no error)=w668) -> ()  [unwired: 1 out]
        n512 = Close Reference(reference=w677, error in (no error)=w678) -> (error out=w675:errorcluster)
      }
      frame "Configure" {
        n513 = call "DATA ENCRYPT STRING FILE WRITE.vi"("error in (no error)"=w697, "User Action"="User Pressed Configure", "main ref"=w683) -> ("error out"=w693:errorcluster)  [unwired: 6 in, 1 out]
        n514 = Unbundle By Name(w683) -> ("Main Home Screen.Configure"=w696:refnum<vi>)
        n515 = Unbundle By Name(w683) -> ("Main Home Screen.MainPage"=w688:refnum<vi>)
        n516 = Unbundle By Name(w683) -> ("Main Home Screen.GUI"=w686:refnum<vi>)
        n517 = property class="Bool (strict)"(reference=w696, error in=w693, "Value"=FALSE) -> (reference out=w694:refnum<vi>, error out=w695:errorcluster)
        n518 = property class="TabCtl (strict)"(reference=w688, "Value"=T5."Details") -> (reference out=w690:refnum<vi>, error out=w689:errorcluster)  [unwired: 1 in]
        n519 = property class="TabCtl (strict)"(reference=w686, "Value"=T4."Setup") -> (reference out=w684:refnum<vi>, error out=w685:errorcluster)  [unwired: 1 in]
        n520 = Close Reference(reference=w694, error in (no error)=w695) -> (error out=w692:errorcluster)
        n521 = Close Reference(reference=w690, error in (no error)=w689) -> ()  [unwired: 1 out]
        n522 = Close Reference(reference=w684, error in (no error)=w685) -> ()  [unwired: 1 out]
      }
      frame "Analysis" {
        n523 = call "DATA ENCRYPT STRING FILE WRITE.vi"("error in (no error)"=w714, "User Action"="User Pressed Analysis", "main ref"=w700) -> ("error out"=w710:errorcluster)  [unwired: 6 in, 1 out]
        n524 = Unbundle By Name(w700) -> ("Main Home Screen.MainPage"=w705:refnum<vi>)
        n525 = Unbundle By Name(w700) -> ("Main Home Screen.Analysis"=w713:refnum<vi>)
        n526 = Unbundle By Name(w700) -> ("Main Home Screen.GUI"=w703:refnum<vi>)
        n527 = property class="Bool (strict)"(reference=w713, error in=w710, "Value"=FALSE) -> (reference out=w711:refnum<vi>, error out=w712:errorcluster)
        n528 = property class="TabCtl (strict)"(reference=w705, "Value"=T5."Analysis") -> (reference out=w707:refnum<vi>, error out=w706:errorcluster)  [unwired: 1 in]
        n529 = property class="TabCtl (strict)"(reference=w703, "Value"=T4."Setup") -> (reference out=w701:refnum<vi>, error out=w702:errorcluster)  [unwired: 1 in]
        n530 = Close Reference(reference=w711, error in (no error)=w712) -> (error out=w709:errorcluster)
        n531 = Close Reference(reference=w707, error in (no error)=w706) -> ()  [unwired: 1 out]
        n532 = Close Reference(reference=w701, error in (no error)=w702) -> ()  [unwired: 1 out]
      }
      frame "service 2" {
        n533 = call "DATA ENCRYPT STRING FILE WRITE.vi"("error in (no error)"=w735, "User Action"="User Pressed service", "main ref"=w718) -> ("error out"=w731:errorcluster)  [unwired: 6 in, 1 out]
        n534 = Unbundle By Name(w718) -> ("Main Screen.Main Screen Tab"=w719:refnum<vi>)
        n535 = Unbundle By Name(w718) -> ("Main Home Screen.MainPage"=w726:refnum<vi>)
        n536 = Unbundle By Name(w718) -> ("Main Home Screen.Analysis"=w734:refnum<vi>)
        n537 = Unbundle By Name(w718) -> ("Main Home Screen.GUI"=w724:refnum<vi>)
        n538 = property class="Bool (strict)"(reference=w734, error in=w731, "Value"=FALSE) -> (reference out=w732:refnum<vi>, error out=w733:errorcluster)
        n539 = property class="TabCtl (strict)"(reference=w726, "Value"=T5."HOME") -> (reference out=w728:refnum<vi>, error out=w727:errorcluster)  [unwired: 1 in]
        n540 = property class="TabCtl (strict)"(reference=w724, "Value"=T4."Begin") -> (reference out=w722:refnum<vi>, error out=w723:errorcluster)  [unwired: 1 in]
        n541 = property class="TabCtl (strict)"(reference=w719, "Value"=T8."About") -> (reference out=w716:refnum<vi>, error out=w720:errorcluster)  [unwired: 1 in]
        n542 = Close Reference(reference=w732, error in (no error)=w733) -> (error out=w730:errorcluster)
        n543 = Close Reference(reference=w728, error in (no error)=w727) -> ()  [unwired: 1 out]
        n544 = Close Reference(reference=w722, error in (no error)=w723) -> ()  [unwired: 1 out]
        n545 = Close Reference(reference=w716, error in (no error)=w720) -> ()  [unwired: 1 out]
      }
      frame "Auto" {
        n546 = call "DATA ENCRYPT STRING FILE WRITE.vi"("error in (no error)"=w747, "User Action"="User Pressed Auto File Name", "main ref"=w737) -> ("error out"=w744:errorcluster)  [unwired: 6 in, 1 out]
        n547 = Get Date/Time In Seconds() -> (seconds since 1Jan1904=w745:timestamp)
        n548 = Format Into String(format string="%<%I_%M_%S_%p_%d_%B_%Y>T", error in=w744, w745) -> (resulting string=w738:string, error out=w740:errorcluster)  [unwired: 1 in]
        n549 = Unbundle By Name(w737) -> ("Config Screen.FILE"=w743:refnum<vi>)
        n550 = property class="Str"(reference=w743, error in=w740, "Value"=w738) -> (reference out=w741:refnum<vi>, error out=w742:errorcluster)
        n551 = Close Reference(reference=w741, error in (no error)=w742) -> (error out=w739:errorcluster)
      }
      frame "Select Load Head" {
        n552 = Unbundle By Name(w752) -> ("Loading.Enter the Loading Rate (N/min)"=w773:refnum<vi>)
        n553 = Unbundle By Name(w752) -> ("Loading.Communication is established"=w758:refnum<vi>)
        n554 = call "DATA ENCRYPT STRING FILE WRITE.vi"("error in (no error)"=w797, "User Action"="User Pressed Select Load Head", "main ref"=w752) -> ("error out"=w793:errorcluster)  [unwired: 6 in, 1 out]
        n555 = Unbundle By Name(w752) -> ("Loading.Enter the Final Load (N)"=w768:refnum<vi>)
        n556 = Unbundle By Name(w752) -> ("Loading.DecaForce COM Status"=w754:refnum<vi>)
        n557 = Unbundle By Name(w752) -> ("Loading.Loading Mode"=w796:refnum<vi>)
        n558 = Unbundle By Name(w752) -> ("Config Screen.Select Load Head"=w780:refnum<vi>)
        n559 = Unbundle By Name(w752) -> ("Loading.Warning"=w763:refnum<vi>)
        n560 = Unbundle By Name(w752) -> ("Loading.Load Selection"=w789:refnum<vi>)
        n561 = property class="Bool (strict)"(reference=w780, "Value"=FALSE) -> (reference out=w778:refnum<vi>, error out=w779:errorcluster)  [unwired: 1 in]
        n562 = property class="TabCtl (strict)"(reference=w789, "Value"=T6."Constant") -> (reference out=w791:refnum<vi>, error out=w790:errorcluster)  [unwired: 1 in]
        n563 = property class="Ring (strict)"(reference=w796, error in=w793, "Value"=u16 0) -> (reference out=w794:refnum<vi>, error out=w795:errorcluster)
        n564 = property class="DigNum (strict)"(reference=w773, "DisabledEnum"=T13."Disabled and Grayed Out" ("Disabled")) -> (reference out=w772:refnum<vi>, error out=w774:errorcluster)  [unwired: 1 in]
        n565 = property class="DigNum (strict)"(reference=w768, "DisabledEnum"=T13."Disabled and Grayed Out" ("Disabled")) -> (reference out=w769:refnum<vi>, error out=w767:errorcluster)  [unwired: 1 in]
        n566 = property class="TabCtl (strict)"(reference=w763, "Visible"=FALSE) -> (reference out=w762:refnum<vi>, error out=w764:errorcluster)  [unwired: 1 in]
        n567 = property class="Bool (strict)"(reference=w758, "Visible"=FALSE) -> (reference out=w756:refnum<vi>, error out=w757:errorcluster)  [unwired: 1 in]
        n568 = property class="Bool (strict)"(reference=w754, "Visible"=FALSE) -> (reference out=w749:refnum<vi>, error out=w755:errorcluster)  [unwired: 1 in]
        n569 = Close Reference(reference=w778, error in (no error)=w779) -> (error out=w776:errorcluster)
        n570 = Close Reference(reference=w791, error in (no error)=w790) -> (error out=w782:errorcluster)
        n571 = Close Reference(reference=w794, error in (no error)=w795) -> (error out=w784:errorcluster)
        n572 = Close Reference(reference=w772, error in (no error)=w774) -> (error out=w766:errorcluster)
        n573 = Close Reference(reference=w769, error in (no error)=w767) -> (error out=w765:errorcluster)
        n574 = Close Reference(reference=w762, error in (no error)=w764) -> (error out=w761:errorcluster)
        n575 = Close Reference(reference=w756, error in (no error)=w757) -> (error out=w751:errorcluster)
        n576 = Close Reference(reference=w749, error in (no error)=w755) -> (error out=w750:errorcluster)
        n577 = Merge Errors(w784, w782, w776, w766, w765, w761, w751, w750) -> (w783:errorcluster)
        n578 = Unbundle By Name(w752) -> ("Main Home Screen.GUI"=w785:refnum<vi>)
        n579 = property class="TabCtl (strict)"(reference=w785, error in=w783, "Value"=T4."Load Head") -> (reference out=w787:refnum<vi>, error out=w786:errorcluster)
        n580 = Close Reference(reference=w787, error in (no error)=w786) -> (error out=w775:errorcluster)
      }
      frame "com 3" {
        n581 = call "DATA ENCRYPT STRING FILE WRITE.vi"("error in (no error)"=w801, "User Action"="User Pressed Check Load Communication", "main ref"=w800) -> ("error out"=w799:errorcluster)  [unwired: 6 in, 1 out]
      }
      frame "Loading Mode" {
        n582 = Unbundle By Name(w805) -> ("Loading.Loading Mode"=w807:refnum<vi>)
        n583 = property class="Ring (strict)"(reference=w807, error in=w806) -> (reference out=w809:refnum<vi>, error out=w808:errorcluster, "Value"=w803:u16)
        n584 = Close Reference(reference=w809, error in (no error)=w808) -> (error out=w804:errorcluster)
        n585 = case shown="1" w803 {
          tunnel: [w824 w841 w853 w865] -> w810
          tunnel: w805 -> [w811 w827 w845 w857]
          tunnel: w804 -> [w825 w840 w852 w864]
          frame 0, Default {
            n586 = Unbundle By Name(w811) -> ("Loading.Enter the Loading Rate (N/min)"=w818:refnum<vi>)
            n587 = Unbundle By Name(w811) -> ("Loading.Load Selection"=w821:refnum<vi>)
            n588 = Unbundle By Name(w811) -> ("Loading.Enter the Final Load (N)"=w813:refnum<vi>)
            n589 = property class="TabCtl (strict)"(reference=w821, "Value"=T6."Constant") -> (reference out=w823:refnum<vi>, error out=w822:errorcluster)  [unwired: 1 in]
            n590 = property class="DigNum (strict)"(reference=w818, "DisabledEnum"=T13."Disabled and Grayed Out" ("Disabled")) -> (reference out=w817:refnum<vi>, error out=w819:errorcluster)  [unwired: 1 in]
            n591 = property class="DigNum (strict)"(reference=w813, "DisabledEnum"=T13."Disabled and Grayed Out" ("Disabled")) -> (reference out=w814:refnum<vi>, error out=w812:errorcluster)  [unwired: 1 in]
            n592 = call "DATA ENCRYPT STRING FILE WRITE.vi"("error in (no error)"=w825, "User Action"="User selected Constant Mode", "main ref"=w811) -> ("error out"=w824:errorcluster)  [unwired: 6 in, 1 out]
            n593 = Close Reference(reference=w823, error in (no error)=w822) -> ()  [unwired: 1 out]
            n594 = Close Reference(reference=w817, error in (no error)=w819) -> ()  [unwired: 1 out]
            n595 = Close Reference(reference=w814, error in (no error)=w812) -> ()  [unwired: 1 out]
          }
          frame 1 {
            n596 = Unbundle By Name(w827) -> ("Loading.Enter the Loading Rate (N/min)"=w838:refnum<vi>)
            n597 = Unbundle By Name(w827) -> ("Loading.Enter the Final Load (N)"=w833:refnum<vi>)
            n598 = Unbundle By Name(w827) -> ("Loading.Load Selection"=w829:refnum<vi>)
            n599 = property class="TabCtl (strict)"(reference=w829, "Value"=T6."Constant") -> (reference out=w831:refnum<vi>, error out=w830:errorcluster)  [unwired: 1 in]
            n600 = property class="DigNum (strict)"(reference=w838, "DisabledEnum"=T13."Enabled" ("Disabled")) -> (reference out=w837:refnum<vi>, error out=w839:errorcluster)  [unwired: 1 in]
            n601 = property class="DigNum (strict)"(reference=w833, "DisabledEnum"=T13."Enabled" ("Disabled")) -> (reference out=w834:refnum<vi>, error out=w832:errorcluster)  [unwired: 1 in]
            n602 = call "DATA ENCRYPT STRING FILE WRITE.vi"("error in (no error)"=w840, "User Action"="User selected Ramp Mode", "main ref"=w827) -> ("error out"=w841:errorcluster)  [unwired: 6 in, 1 out]
            n603 = Close Reference(reference=w831, error in (no error)=w830) -> ()  [unwired: 1 out]
            n604 = Close Reference(reference=w837, error in (no error)=w839) -> ()  [unwired: 1 out]
            n605 = Close Reference(reference=w834, error in (no error)=w832) -> ()  [unwired: 1 out]
          }
          frame 2 {
            n606 = Unbundle By Name(w845) -> ("Loading.Load Selection"=w849:refnum<vi>)
            n607 = Unbundle By Name(w845) -> ("Loading.Warning 2"=w847:refnum<vi>)
            n608 = property class="TabCtl (strict)"(reference=w849, "Value"=T6."Step") -> (reference out=w851:refnum<vi>, error out=w850:errorcluster)  [unwired: 1 in]
            n609 = property class="Bool (strict)"(reference=w847, "Visible"=FALSE) -> (reference out=w843:refnum<vi>, error out=w846:errorcluster)  [unwired: 1 in]
            n610 = call "DATA ENCRYPT STRING FILE WRITE.vi"("error in (no error)"=w852, "User Action"="User selected Step Mode", "main ref"=w845) -> ("error out"=w853:errorcluster)  [unwired: 6 in, 1 out]
            n611 = Close Reference(reference=w851, error in (no error)=w850) -> ()  [unwired: 1 out]
            n612 = Close Reference(reference=w843, error in (no error)=w846) -> ()  [unwired: 1 out]
          }
          frame 3 {
            n613 = Unbundle By Name(w857) -> ("Loading.Load Selection"=w861:refnum<vi>)
            n614 = Unbundle By Name(w857) -> ("Loading.Warning 2"=w859:refnum<vi>)
            n615 = property class="TabCtl (strict)"(reference=w861, "Value"=T6."Indentation") -> (reference out=w863:refnum<vi>, error out=w862:errorcluster)  [unwired: 1 in]
            n616 = property class="Bool (strict)"(reference=w859, "Visible"=FALSE) -> (reference out=w855:refnum<vi>, error out=w858:errorcluster)  [unwired: 1 in]
            n617 = call "DATA ENCRYPT STRING FILE WRITE.vi"("error in (no error)"=w864, "User Action"="User selected Indentation Mode", "main ref"=w857) -> ("error out"=w865:errorcluster)  [unwired: 6 in, 1 out]
            n618 = Close Reference(reference=w863, error in (no error)=w862) -> ()  [unwired: 1 out]
            n619 = Close Reference(reference=w855, error in (no error)=w858) -> ()  [unwired: 1 out]
          }
        }
      }
      frame "SSP 0.3" {
        n620 = Unbundle By Name(w869) -> ("Loading.SSP 0.3"=w872:refnum<vi>)
        n621 = property class="Bool (strict)"(reference=w872, error in=w871) -> (reference out=w874:refnum<vi>, error out=w873:errorcluster, "Value"=w870:bool)
        n622 = Close Reference(reference=w874, error in (no error)=w873) -> (error out=w868:errorcluster)
        n623 = case shown="True" w870 {
          tunnel: w869 -> [_ w876]
          tunnel: w868 -> [w875 w884]
          tunnel: [w875 w883] -> w867
          frame False {
          }
          frame True {
            w886 = FALSE ("Value")
            n624 = Unbundle By Name(w876) -> ("Loading.Enter the Load  (N)"=w882:refnum<vi>)
            n625 = Unbundle By Name(w876) -> ("Loading.SSP 0.75"=w887:refnum<vi>)
            n626 = Unbundle By Name(w876) -> ("Loading.SSP 0.5"=w892:refnum<vi>)
            n627 = property class="Bool (strict)"(reference=w887, "Value"=w886) -> (reference out=w889:refnum<vi>, error out=w888:errorcluster)  [unwired: 1 in]
            n628 = property class="Bool (strict)"(reference=w892, "Value"=w886) -> (reference out=w890:refnum<vi>, error out=w891:errorcluster)  [unwired: 1 in]
            n629 = property class="DigNum (strict)"(reference=w882, "Minimum"=2.0 ("Data Entry Limits:Minimum"), "Maximum"=50.0 ("Data Entry Limits:Maximum"), "Increment"=0.1 ("Data Entry Limits:Increment")) -> (reference out=w880:refnum<vi>, error out=w881:errorcluster)  [unwired: 1 in]
            n630 = call "DATA ENCRYPT STRING FILE WRITE.vi"("error in (no error)"=w884, "User Action"="User selected 0.3 SSP", "main ref"=w876) -> ("error out"=w883:errorcluster)  [unwired: 6 in, 1 out]
            n631 = Close Reference(reference=w889, error in (no error)=w888) -> ()  [unwired: 1 out]
            n632 = Close Reference(reference=w890, error in (no error)=w891) -> ()  [unwired: 1 out]
            n633 = Close Reference(reference=w880, error in (no error)=w881) -> ()  [unwired: 1 out]
          }
        }
      }
      frame "SSP 0.5" {
        n634 = Unbundle By Name(w895) -> ("Loading.SSP 0.5"=w898:refnum<vi>)
        n635 = property class="Bool (strict)"(reference=w898, error in=w897) -> (reference out=w900:refnum<vi>, error out=w899:errorcluster, "Value"=w896:bool)
        n636 = Close Reference(reference=w900, error in (no error)=w899) -> (error out=w894:errorcluster)
        n637 = case shown="True" w896 {
          tunnel: w895 -> [_ w902]
          tunnel: w894 -> [w901 w910]
          tunnel: [w901 w909] -> w893
          frame False {
          }
          frame True {
            w912 = FALSE ("Value")
            n638 = Unbundle By Name(w902) -> ("Loading.Enter the Load  (N)"=w908:refnum<vi>)
            n639 = Unbundle By Name(w902) -> ("Loading.SSP 0.75"=w918:refnum<vi>)
            n640 = Unbundle By Name(w902) -> ("Loading.SSP 0.3"=w913:refnum<vi>)
            n641 = property class="Bool (strict)"(reference=w913, "Value"=w912) -> (reference out=w915:refnum<vi>, error out=w914:errorcluster)  [unwired: 1 in]
            n642 = property class="Bool (strict)"(reference=w918, "Value"=w912) -> (reference out=w916:refnum<vi>, error out=w917:errorcluster)  [unwired: 1 in]
            n643 = property class="DigNum (strict)"(reference=w908, "Minimum"=2.0 ("Data Entry Limits:Minimum"), "Maximum"=200.0 ("Data Entry Limits:Maximum"), "Increment"=0.1 ("Data Entry Limits:Increment")) -> (reference out=w906:refnum<vi>, error out=w907:errorcluster)  [unwired: 1 in]
            n644 = call "DATA ENCRYPT STRING FILE WRITE.vi"("error in (no error)"=w910, "User Action"="User selected 0.5 SSP", "main ref"=w902) -> ("error out"=w909:errorcluster)  [unwired: 6 in, 1 out]
            n645 = Close Reference(reference=w915, error in (no error)=w914) -> ()  [unwired: 1 out]
            n646 = Close Reference(reference=w916, error in (no error)=w917) -> ()  [unwired: 1 out]
            n647 = Close Reference(reference=w906, error in (no error)=w907) -> ()  [unwired: 1 out]
          }
        }
      }
      frame "SSP 0.75" {
        n648 = Unbundle By Name(w921) -> ("Loading.SSP 0.75"=w924:refnum<vi>)
        n649 = property class="Bool (strict)"(reference=w924, error in=w923) -> (reference out=w926:refnum<vi>, error out=w925:errorcluster, "Value"=w922:bool)
        n650 = Close Reference(reference=w926, error in (no error)=w925) -> (error out=w920:errorcluster)
        n651 = case shown="True" w922 {
          tunnel: w921 -> [_ w928]
          tunnel: w920 -> [w927 w936]
          tunnel: [w927 w935] -> w919
          frame False {
          }
          frame True {
            w938 = FALSE ("Value")
            n652 = Unbundle By Name(w928) -> ("Loading.SSP 0.3"=w939:refnum<vi>)
            n653 = Unbundle By Name(w928) -> ("Loading.SSP 0.5"=w944:refnum<vi>)
            n654 = Unbundle By Name(w928) -> ("Loading.Enter the Load  (N)"=w934:refnum<vi>)
            n655 = property class="Bool (strict)"(reference=w939, "Value"=w938) -> (reference out=w941:refnum<vi>, error out=w940:errorcluster)  [unwired: 1 in]
            n656 = property class="Bool (strict)"(reference=w944, "Value"=w938) -> (reference out=w942:refnum<vi>, error out=w943:errorcluster)  [unwired: 1 in]
            n657 = property class="DigNum (strict)"(reference=w934, "Minimum"=200.0 ("Data Entry Limits:Minimum"), "Maximum"=500.0 ("Data Entry Limits:Maximum"), "Increment"=0.1 ("Data Entry Limits:Increment")) -> (reference out=w932:refnum<vi>, error out=w933:errorcluster)  [unwired: 1 in]
            n658 = call "DATA ENCRYPT STRING FILE WRITE.vi"("error in (no error)"=w936, "User Action"="User selected 0.75 SSP", "main ref"=w928) -> ("error out"=w935:errorcluster)  [unwired: 6 in, 1 out]
            n659 = Close Reference(reference=w941, error in (no error)=w940) -> ()  [unwired: 1 out]
            n660 = Close Reference(reference=w942, error in (no error)=w943) -> ()  [unwired: 1 out]
            n661 = Close Reference(reference=w932, error in (no error)=w933) -> ()  [unwired: 1 out]
          }
        }
      }
      frame "LHBack" {
        # "Back to Configure"
        n662 = Unbundle By Name(w945) -> ("Main Home Screen.GUI"=w951:refnum<vi>)
        n663 = Unbundle By Name(w945) -> ("Main Home Screen.MainPage"=w947:refnum<vi>)
        n664 = property class="TabCtl (strict)"(reference=w947, "Value"=T5."HOME") -> (reference out=w949:refnum<vi>, error out=w948:errorcluster)  [unwired: 1 in]
        n665 = property class="TabCtl (strict)"(reference=w951, "Value"=T4."Setup") -> (reference out=w953:refnum<vi>, error out=w952:errorcluster)  [unwired: 1 in]
        n666 = Close Reference(reference=w949, error in (no error)=w948) -> ()  [unwired: 1 out]
        n667 = Close Reference(reference=w953, error in (no error)=w952) -> ()  [unwired: 1 out]
        n668 = call "DATA ENCRYPT STRING FILE WRITE.vi"("error in (no error)"=w954, "User Action"="User selected Back to Configure", "main ref"=w945) -> ("error out"=w955:errorcluster)  [unwired: 6 in, 1 out]
      }
      frame "MMBack" {
        # "Back to Configure"
        n669 = Unbundle By Name(w957) -> ("Main Home Screen.GUI"=w963:refnum<vi>)
        n670 = Unbundle By Name(w957) -> ("Main Home Screen.MainPage"=w959:refnum<vi>)
        n671 = property class="TabCtl (strict)"(reference=w959, "Value"=T5."HOME") -> (reference out=w961:refnum<vi>, error out=w960:errorcluster)  [unwired: 1 in]
        n672 = property class="TabCtl (strict)"(reference=w963, "Value"=T4."Load Head") -> (reference out=w965:refnum<vi>, error out=w964:errorcluster)  [unwired: 1 in]
        n673 = Close Reference(reference=w961, error in (no error)=w960) -> ()  [unwired: 1 out]
        n674 = Close Reference(reference=w965, error in (no error)=w964) -> ()  [unwired: 1 out]
        n675 = call "DATA ENCRYPT STRING FILE WRITE.vi"("error in (no error)"=w966, "User Action"="User selected Back to Load Selection", "main ref"=w957) -> ("error out"=w967:errorcluster)  [unwired: 6 in, 1 out]
      }
      frame "LHNext" {
        w999 = FALSE ("Visible")
        n676 = Unbundle By Name(w969) -> ("Motion Module.HomeRot"=w1005:refnum<vi>)
        n677 = Unbundle By Name(w969) -> ("Motion Module.HomeScratch"=w1000:refnum<vi>)
        n678 = Unbundle By Name(w969) -> ("Motion Module.PlaceModule"=w998:refnum<vi>)
        n679 = Unbundle By Name(w969) -> ("Motion Module.Motion Mode:"=w991:refnum<vi>)
        n680 = Unbundle By Name(w969) -> ("Motion Module.Motion Direction:  3"=w990:refnum<vi>)
        n681 = Unbundle By Name(w969) -> ("Motion Module.Wear Track Diameter (mm)"=w984:refnum<vi>)
        n682 = Unbundle By Name(w969) -> ("Motion Module.Set WTD"=w981:refnum<vi>)
        n683 = Unbundle By Name(w969) -> ("Motion Module.Rotary Module Selection"=w975:refnum<vi>)
        n684 = call "DATA ENCRYPT STRING FILE WRITE.vi"("error in (no error)"=w1014, "User Action"="User selected Select Module", "main ref"=w969) -> ("error out"=w978:errorcluster)  [unwired: 6 in, 1 out]
        n685 = property class="TabCtl (strict)"(reference=w975, "Visible"=FALSE) -> (reference out=w974:refnum<vi>, error out=w976:errorcluster)  [unwired: 1 in]
        n686 = property class="Bool (strict)"(reference=w1005, error in=w978, "Visible"=w999) -> (reference out=w1003:refnum<vi>, error out=w1004:errorcluster)
        n687 = property class="Bool (strict)"(reference=w1000, error in=w978, "Visible"=w999) -> (reference out=w1002:refnum<vi>, error out=w1001:errorcluster)
        n688 = property class="Bool (strict)"(reference=w998, error in=w978, "Visible"=TRUE) -> (reference out=w996:refnum<vi>, error out=w997:errorcluster)
        n689 = property class="Ring (strict)"(reference=w991, error in=w978, "Visible"=FALSE) -> (reference out=w993:refnum<vi>, error out=w992:errorcluster)
        n690 = property class="Ring (strict)"(reference=w990, error in=w978, "Visible"=FALSE) -> (reference out=w987:refnum<vi>, error out=w989:errorcluster)
        n691 = property class="DigNum (strict)"(reference=w984, "Visible"=FALSE) -> (reference out=w983:refnum<vi>, error out=w985:errorcluster)  [unwired: 1 in]
        n692 = property class="Bool (strict)"(reference=w981, "Visible"=FALSE) -> (reference out=w982:refnum<vi>, error out=w980:errorcluster)  [unwired: 1 in]
        n693 = Close Reference(reference=w1003, error in (no error)=w1004) -> ()  [unwired: 1 out]
        n694 = Close Reference(reference=w1002, error in (no error)=w1001) -> ()  [unwired: 1 out]
        n695 = Close Reference(reference=w996, error in (no error)=w997) -> ()  [unwired: 1 out]
        n696 = Close Reference(reference=w993, error in (no error)=w992) -> ()  [unwired: 1 out]
        n697 = Close Reference(reference=w987, error in (no error)=w989) -> ()  [unwired: 1 out]
        n698 = Close Reference(reference=w983, error in (no error)=w985) -> ()  [unwired: 1 out]
        n699 = Close Reference(reference=w974, error in (no error)=w976) -> ()  [unwired: 1 out]
        n700 = Close Reference(reference=w982, error in (no error)=w980) -> ()  [unwired: 1 out]
        n701 = Unbundle By Name(w969) -> ("Motion Module.M3 Image"=w973:refnum<vi>)
        n702 = Unbundle By Name(w969) -> ("Main Home Screen.GUI"=w1011:refnum<vi>)
        n703 = Unbundle By Name(w969) -> ("Main Home Screen.MainPage"=w1007:refnum<vi>)
        n704 = property class="TabCtl (strict)"(reference=w973, "Value"=enum32{"Page 1", "Page 2"}."Page 2") -> (reference out=w971:refnum<vi>, error out=w972:errorcluster)  [unwired: 1 in]
        n705 = property class="TabCtl (strict)"(reference=w1007, "Value"=T5."HOME") -> (reference out=w1009:refnum<vi>, error out=w1008:errorcluster)  [unwired: 1 in]
        n706 = property class="TabCtl (strict)"(reference=w1011, "Value"=T4."Motion Module") -> (reference out=w1013:refnum<vi>, error out=w1012:errorcluster)  [unwired: 1 in]
        n707 = Close Reference(reference=w971, error in (no error)=w972) -> ()  [unwired: 1 out]
        n708 = Close Reference(reference=w1009, error in (no error)=w1008) -> ()  [unwired: 1 out]
        n709 = Close Reference(reference=w1013, error in (no error)=w1012) -> ()  [unwired: 1 out]
      }
      frame "Rot Ver" {
        # "Rot Ver"
        n710 = Unbundle By Name(w1018) -> ("Motion Module.Rot Ver"=w1017:refnum<vi>)
        n711 = property class="Bool (strict)"(reference=w1017) -> (reference out=w1020:refnum<vi>, error out=w1019:errorcluster, "Value"=w1016:bool)  [unwired: 1 in]
        n712 = Close Reference(reference=w1020, error in (no error)=w1019) -> ()  [unwired: 1 out]
        n713 = case shown="True" w1016 {
          tunnel: w1034 -> [w1069 w1104]
          tunnel: [w1041 w1104] -> w1025
          tunnel: w1018 -> [w1035 w1071]
          frame True {
            n714 = Unbundle By Name(w1035) -> ("Motion Module.HomeRot"=w1068:refnum<vi>)
            n715 = Unbundle By Name(w1035) -> ("Motion Module.HomeScratch"=w1063:refnum<vi>)
            n716 = Unbundle By Name(w1035) -> ("Motion Module.PlaceModule"=w1061:refnum<vi>)
            n717 = Unbundle By Name(w1035) -> ("Motion Module.Motion Mode:"=w1054:refnum<vi>)
            n718 = Unbundle By Name(w1035) -> ("Motion Module.Motion Direction:  3"=w1053:refnum<vi>)
            n719 = Unbundle By Name(w1035) -> ("Motion Module.Wear Track Diameter (mm)"=w1047:refnum<vi>)
            n720 = Unbundle By Name(w1035) -> ("Motion Module.Set WTD"=w1044:refnum<vi>)
            n721 = Unbundle By Name(w1035) -> ("Motion Module.Rotary Module Selection"=w1038:refnum<vi>)
            n722 = call "DATA ENCRYPT STRING FILE WRITE.vi"("error in (no error)"=w1069, "User Action"="User selected Rot Vertical Module", "main ref"=w1035) -> ("error out"=w1041:errorcluster)  [unwired: 6 in, 1 out]
            n723 = property class="TabCtl (strict)"(reference=w1038, "Visible"=TRUE) -> (reference out=w1037:refnum<vi>, error out=w1039:errorcluster)  [unwired: 1 in]
            n724 = property class="Bool (strict)"(reference=w1068, error in=w1041, "Visible"=TRUE) -> (reference out=w1066:refnum<vi>, error out=w1067:errorcluster)
            n725 = property class="Bool (strict)"(reference=w1063, error in=w1041, "Visible"=FALSE) -> (reference out=w1065:refnum<vi>, error out=w1064:errorcluster)
            n726 = property class="Bool (strict)"(reference=w1061, error in=w1041, "Visible"=FALSE) -> (reference out=w1059:refnum<vi>, error out=w1060:errorcluster)
            n727 = property class="Ring (strict)"(reference=w1054, error in=w1041, "Visible"=TRUE) -> (reference out=w1056:refnum<vi>, error out=w1055:errorcluster)
            n728 = property class="Ring (strict)"(reference=w1053, error in=w1041, "Visible"=TRUE) -> (reference out=w1050:refnum<vi>, error out=w1052:errorcluster)
            n729 = property class="DigNum (strict)"(reference=w1047, "Visible"=TRUE) -> (reference out=w1046:refnum<vi>, error out=w1048:errorcluster)  [unwired: 1 in]
            n730 = property class="Bool (strict)"(reference=w1044, "Visible"=TRUE) -> (reference out=w1045:refnum<vi>, error out=w1043:errorcluster)  [unwired: 1 in]
            n731 = Close Reference(reference=w1066, error in (no error)=w1067) -> ()  [unwired: 1 out]
            n732 = Close Reference(reference=w1065, error in (no error)=w1064) -> ()  [unwired: 1 out]
            n733 = Close Reference(reference=w1059, error in (no error)=w1060) -> ()  [unwired: 1 out]
            n734 = Close Reference(reference=w1056, error in (no error)=w1055) -> ()  [unwired: 1 out]
            n735 = Close Reference(reference=w1050, error in (no error)=w1052) -> ()  [unwired: 1 out]
            n736 = Close Reference(reference=w1046, error in (no error)=w1048) -> ()  [unwired: 1 out]
            n737 = Close Reference(reference=w1037, error in (no error)=w1039) -> ()  [unwired: 1 out]
            n738 = Close Reference(reference=w1045, error in (no error)=w1043) -> ()  [unwired: 1 out]
          }
          frame False {
            n739 = Unbundle By Name(w1071) -> ("Motion Module.HomeRot"=w1103:refnum<vi>)
            n740 = Unbundle By Name(w1071) -> ("Motion Module.HomeScratch"=w1098:refnum<vi>)
            n741 = Unbundle By Name(w1071) -> ("Motion Module.PlaceModule"=w1096:refnum<vi>)
            n742 = Unbundle By Name(w1071) -> ("Motion Module.Motion Mode:"=w1089:refnum<vi>)
            n743 = Unbundle By Name(w1071) -> ("Motion Module.Motion Direction:  3"=w1088:refnum<vi>)
            n744 = Unbundle By Name(w1071) -> ("Motion Module.Wear Track Diameter (mm)"=w1082:refnum<vi>)
            n745 = Unbundle By Name(w1071) -> ("Motion Module.Set WTD"=w1079:refnum<vi>)
            n746 = Unbundle By Name(w1071) -> ("Motion Module.Rotary Module Selection"=w1074:refnum<vi>)
            n747 = property class="TabCtl (strict)"(reference=w1074, "Visible"=FALSE) -> (reference out=w1073:refnum<vi>, error out=w1075:errorcluster)  [unwired: 1 in]
            n748 = property class="Bool (strict)"(reference=w1103, error in=w1104, "Visible"=FALSE) -> (reference out=w1101:refnum<vi>, error out=w1102:errorcluster)
            n749 = property class="Bool (strict)"(reference=w1098, error in=w1104, "Visible"=FALSE) -> (reference out=w1100:refnum<vi>, error out=w1099:errorcluster)
            n750 = property class="Bool (strict)"(reference=w1096, error in=w1104, "Visible"=TRUE) -> (reference out=w1094:refnum<vi>, error out=w1095:errorcluster)
            n751 = property class="Ring (strict)"(reference=w1089, error in=w1104, "Visible"=FALSE) -> (reference out=w1091:refnum<vi>, error out=w1090:errorcluster)
            n752 = property class="Ring (strict)"(reference=w1088, error in=w1104, "Visible"=FALSE) -> (reference out=w1085:refnum<vi>, error out=w1087:errorcluster)
            n753 = property class="DigNum (strict)"(reference=w1082, "Visible"=FALSE) -> (reference out=w1081:refnum<vi>, error out=w1083:errorcluster)  [unwired: 1 in]
            n754 = property class="Bool (strict)"(reference=w1079, "Visible"=FALSE) -> (reference out=w1080:refnum<vi>, error out=w1078:errorcluster)  [unwired: 1 in]
            n755 = Close Reference(reference=w1101, error in (no error)=w1102) -> ()  [unwired: 1 out]
            n756 = Close Reference(reference=w1100, error in (no error)=w1099) -> ()  [unwired: 1 out]
            n757 = Close Reference(reference=w1094, error in (no error)=w1095) -> ()  [unwired: 1 out]
            n758 = Close Reference(reference=w1091, error in (no error)=w1090) -> ()  [unwired: 1 out]
            n759 = Close Reference(reference=w1085, error in (no error)=w1087) -> ()  [unwired: 1 out]
            n760 = Close Reference(reference=w1081, error in (no error)=w1083) -> ()  [unwired: 1 out]
            n761 = Close Reference(reference=w1073, error in (no error)=w1075) -> ()  [unwired: 1 out]
            n762 = Close Reference(reference=w1080, error in (no error)=w1078) -> ()  [unwired: 1 out]
          }
        }
        n763 = Unbundle By Name(w1018) -> ("Motion Module.M3 Image"=w1024:refnum<vi>)
        n764 = Unbundle By Name(w1018) -> ("Main Home Screen.GUI"=w1031:refnum<vi>)
        n765 = Unbundle By Name(w1018) -> ("Main Home Screen.MainPage"=w1027:refnum<vi>)
        n766 = property class="TabCtl (strict)"(reference=w1024, "Value"=enum32{"Page 1", "Page 2"}."Page 1") -> (reference out=w1022:refnum<vi>, error out=w1023:errorcluster)  [unwired: 1 in]
        n767 = property class="TabCtl (strict)"(reference=w1027, "Value"=T5."HOME") -> (reference out=w1029:refnum<vi>, error out=w1028:errorcluster)  [unwired: 1 in]
        n768 = property class="TabCtl (strict)"(reference=w1031, "Value"=T4."Motion Module") -> (reference out=w1033:refnum<vi>, error out=w1032:errorcluster)  [unwired: 1 in]
        n769 = Close Reference(reference=w1022, error in (no error)=w1023) -> ()  [unwired: 1 out]
        n770 = Close Reference(reference=w1029, error in (no error)=w1028) -> ()  [unwired: 1 out]
        n771 = Close Reference(reference=w1033, error in (no error)=w1032) -> ()  [unwired: 1 out]
      }
      frame "Scratch" {
        n772 = Unbundle By Name(w1106) -> ("Motion Module.Scratch"=w1107:refnum<vi>)
        n773 = property class="Bool (strict)"(reference=w1107) -> (reference out=w1109:refnum<vi>, error out=w1108:errorcluster, "Value"=w1105:bool)  [unwired: 1 in]
        n774 = Close Reference(reference=w1109, error in (no error)=w1108) -> ()  [unwired: 1 out]
        n775 = case shown="True" w1105 {
          tunnel: w1123 -> [w1158 w1193]
          tunnel: [w1130 w1193] -> w1114
          tunnel: w1106 -> [w1124 w1160]
          frame True {
            n776 = Unbundle By Name(w1124) -> ("Motion Module.HomeRot"=w1157:refnum<vi>)
            n777 = Unbundle By Name(w1124) -> ("Motion Module.HomeScratch"=w1152:refnum<vi>)
            n778 = Unbundle By Name(w1124) -> ("Motion Module.PlaceModule"=w1150:refnum<vi>)
            n779 = Unbundle By Name(w1124) -> ("Motion Module.Motion Mode:"=w1143:refnum<vi>)
            n780 = Unbundle By Name(w1124) -> ("Motion Module.Motion Direction:  3"=w1142:refnum<vi>)
            n781 = Unbundle By Name(w1124) -> ("Motion Module.Wear Track Diameter (mm)"=w1136:refnum<vi>)
            n782 = Unbundle By Name(w1124) -> ("Motion Module.Set WTD"=w1133:refnum<vi>)
            n783 = Unbundle By Name(w1124) -> ("Motion Module.Rotary Module Selection"=w1127:refnum<vi>)
            n784 = call "DATA ENCRYPT STRING FILE WRITE.vi"("error in (no error)"=w1158, "User Action"="User selected Scratch Module", "main ref"=w1124) -> ("error out"=w1130:errorcluster)  [unwired: 6 in, 1 out]
            n785 = property class="TabCtl (strict)"(reference=w1127, "Visible"=FALSE) -> (reference out=w1126:refnum<vi>, error out=w1128:errorcluster)  [unwired: 1 in]
            n786 = property class="Bool (strict)"(reference=w1157, error in=w1130, "Visible"=FALSE) -> (reference out=w1155:refnum<vi>, error out=w1156:errorcluster)
            n787 = property class="Bool (strict)"(reference=w1152, error in=w1130, "Visible"=TRUE) -> (reference out=w1154:refnum<vi>, error out=w1153:errorcluster)
            n788 = property class="Bool (strict)"(reference=w1150, error in=w1130, "Visible"=FALSE) -> (reference out=w1148:refnum<vi>, error out=w1149:errorcluster)
            n789 = property class="Ring (strict)"(reference=w1143, error in=w1130, "Visible"=FALSE) -> (reference out=w1145:refnum<vi>, error out=w1144:errorcluster)
            n790 = property class="Ring (strict)"(reference=w1142, error in=w1130, "Visible"=FALSE) -> (reference out=w1139:refnum<vi>, error out=w1141:errorcluster)
            n791 = property class="DigNum (strict)"(reference=w1136, "Visible"=FALSE) -> (reference out=w1135:refnum<vi>, error out=w1137:errorcluster)  [unwired: 1 in]
            n792 = property class="Bool (strict)"(reference=w1133, "Visible"=FALSE) -> (reference out=w1134:refnum<vi>, error out=w1132:errorcluster)  [unwired: 1 in]
            n793 = Close Reference(reference=w1155, error in (no error)=w1156) -> ()  [unwired: 1 out]
            n794 = Close Reference(reference=w1154, error in (no error)=w1153) -> ()  [unwired: 1 out]
            n795 = Close Reference(reference=w1148, error in (no error)=w1149) -> ()  [unwired: 1 out]
            n796 = Close Reference(reference=w1145, error in (no error)=w1144) -> ()  [unwired: 1 out]
            n797 = Close Reference(reference=w1139, error in (no error)=w1141) -> ()  [unwired: 1 out]
            n798 = Close Reference(reference=w1135, error in (no error)=w1137) -> ()  [unwired: 1 out]
            n799 = Close Reference(reference=w1126, error in (no error)=w1128) -> ()  [unwired: 1 out]
            n800 = Close Reference(reference=w1134, error in (no error)=w1132) -> ()  [unwired: 1 out]
          }
          frame False {
            n801 = Unbundle By Name(w1160) -> ("Motion Module.HomeRot"=w1192:refnum<vi>)
            n802 = Unbundle By Name(w1160) -> ("Motion Module.HomeScratch"=w1187:refnum<vi>)
            n803 = Unbundle By Name(w1160) -> ("Motion Module.PlaceModule"=w1185:refnum<vi>)
            n804 = Unbundle By Name(w1160) -> ("Motion Module.Motion Mode:"=w1178:refnum<vi>)
            n805 = Unbundle By Name(w1160) -> ("Motion Module.Motion Direction:  3"=w1177:refnum<vi>)
            n806 = Unbundle By Name(w1160) -> ("Motion Module.Wear Track Diameter (mm)"=w1171:refnum<vi>)
            n807 = Unbundle By Name(w1160) -> ("Motion Module.Set WTD"=w1168:refnum<vi>)
            n808 = Unbundle By Name(w1160) -> ("Motion Module.Rotary Module Selection"=w1163:refnum<vi>)
            n809 = property class="TabCtl (strict)"(reference=w1163, "Visible"=FALSE) -> (reference out=w1162:refnum<vi>, error out=w1164:errorcluster)  [unwired: 1 in]
            n810 = property class="Bool (strict)"(reference=w1192, error in=w1193, "Visible"=FALSE) -> (reference out=w1190:refnum<vi>, error out=w1191:errorcluster)
            n811 = property class="Bool (strict)"(reference=w1187, error in=w1193, "Visible"=FALSE) -> (reference out=w1189:refnum<vi>, error out=w1188:errorcluster)
            n812 = property class="Bool (strict)"(reference=w1185, error in=w1193, "Visible"=TRUE) -> (reference out=w1183:refnum<vi>, error out=w1184:errorcluster)
            n813 = property class="Ring (strict)"(reference=w1178, error in=w1193, "Visible"=FALSE) -> (reference out=w1180:refnum<vi>, error out=w1179:errorcluster)
            n814 = property class="Ring (strict)"(reference=w1177, error in=w1193, "Visible"=FALSE) -> (reference out=w1174:refnum<vi>, error out=w1176:errorcluster)
            n815 = property class="DigNum (strict)"(reference=w1171, "Visible"=FALSE) -> (reference out=w1170:refnum<vi>, error out=w1172:errorcluster)  [unwired: 1 in]
            n816 = property class="Bool (strict)"(reference=w1168, "Visible"=FALSE) -> (reference out=w1169:refnum<vi>, error out=w1167:errorcluster)  [unwired: 1 in]
            n817 = Close Reference(reference=w1190, error in (no error)=w1191) -> ()  [unwired: 1 out]
            n818 = Close Reference(reference=w1189, error in (no error)=w1188) -> ()  [unwired: 1 out]
            n819 = Close Reference(reference=w1183, error in (no error)=w1184) -> ()  [unwired: 1 out]
            n820 = Close Reference(reference=w1180, error in (no error)=w1179) -> ()  [unwired: 1 out]
            n821 = Close Reference(reference=w1174, error in (no error)=w1176) -> ()  [unwired: 1 out]
            n822 = Close Reference(reference=w1170, error in (no error)=w1172) -> ()  [unwired: 1 out]
            n823 = Close Reference(reference=w1162, error in (no error)=w1164) -> ()  [unwired: 1 out]
            n824 = Close Reference(reference=w1169, error in (no error)=w1167) -> ()  [unwired: 1 out]
          }
        }
        n825 = Unbundle By Name(w1106) -> ("Main Home Screen.GUI"=w1120:refnum<vi>)
        n826 = Unbundle By Name(w1106) -> ("Main Home Screen.MainPage"=w1116:refnum<vi>)
        n827 = Unbundle By Name(w1106) -> ("Motion Module.M3 Image"=w1113:refnum<vi>)
        n828 = property class="TabCtl (strict)"(reference=w1116, "Value"=T5."HOME") -> (reference out=w1118:refnum<vi>, error out=w1117:errorcluster)  [unwired: 1 in]
        n829 = property class="TabCtl (strict)"(reference=w1113, "Value"=enum32{"Page 1", "Page 2"}."Page 2") -> (reference out=w1111:refnum<vi>, error out=w1112:errorcluster)  [unwired: 1 in]
        n830 = property class="TabCtl (strict)"(reference=w1120, "Value"=T4."Motion Module") -> (reference out=w1122:refnum<vi>, error out=w1121:errorcluster)  [unwired: 1 in]
        n831 = Close Reference(reference=w1118, error in (no error)=w1117) -> ()  [unwired: 1 out]
        n832 = Close Reference(reference=w1111, error in (no error)=w1112) -> ()  [unwired: 1 out]
        n833 = Close Reference(reference=w1122, error in (no error)=w1121) -> ()  [unwired: 1 out]
      }
      frame "Motion Mode:" {
        n834 = Unbundle By Name(w1194) -> ("Motion Module.Motion Mode:"=w1196:refnum<vi>)
        n835 = property class="Ring (strict)"(reference=w1196) -> (reference out=w1198:refnum<vi>, error out=w1197:errorcluster, "Value"=w1195:u16)  [unwired: 1 in]
        n836 = Close Reference(reference=w1198, error in (no error)=w1197) -> ()  [unwired: 1 out]
        n837 = case shown="3" w1195 {
          tunnel: w1200 -> [w1209 w1218 w1227 w1236]
          tunnel: [w1208 w1217 w1226 w1235] -> w1199
          tunnel: w1194 -> [w1207 w1216 w1225 w1234]
          tunnel: w1194 -> [w1202 w1211 w1220 w1229]
          frame 0, Default {
            n838 = Unbundle By Name(w1202) -> ("Motion Module.Rotary Module Selection"=w1203:refnum<vi>)
            n839 = property class="TabCtl (strict)"(reference=w1203, "Value"=T7."Uniform Rotation") -> (reference out=w1205:refnum<vi>, error out=w1204:errorcluster)  [unwired: 1 in]
            n840 = Close Reference(reference=w1205, error in (no error)=w1204) -> ()  [unwired: 1 out]
            n841 = call "DATA ENCRYPT STRING FILE WRITE.vi"("error in (no error)"=w1209, "User Action"="User Selected Uniform Rotation", "main ref"=w1207) -> ("error out"=w1208:errorcluster)  [unwired: 6 in, 1 out]
          }
          frame 1 {
            n842 = Unbundle By Name(w1211) -> ("Motion Module.Rotary Module Selection"=w1212:refnum<vi>)
            n843 = property class="TabCtl (strict)"(reference=w1212, "Value"=T7."Angular Oscillation") -> (reference out=w1214:refnum<vi>, error out=w1213:errorcluster)  [unwired: 1 in]
            n844 = Close Reference(reference=w1214, error in (no error)=w1213) -> ()  [unwired: 1 out]
            n845 = call "DATA ENCRYPT STRING FILE WRITE.vi"("error in (no error)"=w1218, "User Action"="User Selected Angular Oscillation", "main ref"=w1216) -> ("error out"=w1217:errorcluster)  [unwired: 6 in, 1 out]
          }
          frame 2 {
            n846 = Unbundle By Name(w1220) -> ("Motion Module.Rotary Module Selection"=w1221:refnum<vi>)
            n847 = property class="TabCtl (strict)"(reference=w1221, "Value"=T7."Speed Ramp") -> (reference out=w1223:refnum<vi>, error out=w1222:errorcluster)  [unwired: 1 in]
            n848 = Close Reference(reference=w1223, error in (no error)=w1222) -> ()  [unwired: 1 out]
            n849 = call "DATA ENCRYPT STRING FILE WRITE.vi"("error in (no error)"=w1227, "User Action"="User Selected Ramp Mode", "main ref"=w1225) -> ("error out"=w1226:errorcluster)  [unwired: 6 in, 1 out]
          }
          frame 3 {
            n850 = Unbundle By Name(w1229) -> ("Motion Module.Rotary Module Selection"=w1230:refnum<vi>)
            n851 = property class="TabCtl (strict)"(reference=w1230, "Value"=T7."Speed Step") -> (reference out=w1232:refnum<vi>, error out=w1231:errorcluster)  [unwired: 1 in]
            n852 = Close Reference(reference=w1232, error in (no error)=w1231) -> ()  [unwired: 1 out]
            n853 = call "DATA ENCRYPT STRING FILE WRITE.vi"("error in (no error)"=w1236, "User Action"="User Selected Step Mode", "main ref"=w1234) -> ("error out"=w1235:errorcluster)  [unwired: 6 in, 1 out]
          }
        }
      }
      frame "MMNext" {
        n854 = Unbundle By Name(w1237) -> ("Motion Module.MMNext"=w1244:refnum<vi>)
        n855 = Unbundle By Name(w1237) -> ("Main Home Screen.GUI"=w1246:refnum<vi>)
        n856 = property class="TabCtl (strict)"(reference=w1246, "Value"=T4."Environment") -> (reference out=w1248:refnum<vi>, error out=w1247:errorcluster)  [unwired: 1 in]
        n857 = property class="Bool (strict)"(reference=w1244, "Value"=FALSE) -> (reference out=w1242:refnum<vi>, error out=w1243:errorcluster)  [unwired: 1 in]
        n858 = Close Reference(reference=w1242, error in (no error)=w1243) -> ()  [unwired: 1 out]
        n859 = Close Reference(reference=w1248, error in (no error)=w1247) -> ()  [unwired: 1 out]
        n860 = call "DATA ENCRYPT STRING FILE WRITE.vi"("error in (no error)"=w1239, "User Action"="User Selected SetUp Module", "main ref"=w1237) -> ("error out"=w1238:errorcluster)  [unwired: 6 in, 1 out]
      }
      frame "APBack" {
        n861 = Unbundle By Name(w1249) -> ("Environmental control.APBack"=w1256:refnum<vi>)
        n862 = Unbundle By Name(w1249) -> ("Main Home Screen.GUI"=w1258:refnum<vi>)
        n863 = property class="TabCtl (strict)"(reference=w1258, "Value"=T4."Motion Module") -> (reference out=w1260:refnum<vi>, error out=w1259:errorcluster)  [unwired: 1 in]
        n864 = property class="Bool (strict)"(reference=w1256, "Value"=FALSE) -> (reference out=w1254:refnum<vi>, error out=w1255:errorcluster)  [unwired: 1 in]
        n865 = Close Reference(reference=w1254, error in (no error)=w1255) -> ()  [unwired: 1 out]
        n866 = Close Reference(reference=w1260, error in (no error)=w1259) -> ()  [unwired: 1 out]
        n867 = call "DATA ENCRYPT STRING FILE WRITE.vi"("error in (no error)"=w1251, "User Action"="User Selected Back to Module", "main ref"=w1249) -> ("error out"=w1250:errorcluster)  [unwired: 6 in, 1 out]
      }
      frame "SNext" {
        n868 = Unbundle By Name(w1261) -> ("Environmental control.SNext"=w1268:refnum<vi>)
        n869 = Unbundle By Name(w1261) -> ("Main Home Screen.GUI"=w1270:refnum<vi>)
        n870 = property class="TabCtl (strict)"(reference=w1270, "Value"=T4."Begin") -> (reference out=w1272:refnum<vi>, error out=w1271:errorcluster)  [unwired: 1 in]
        n871 = property class="Bool (strict)"(reference=w1268, "Value"=FALSE) -> (reference out=w1266:refnum<vi>, error out=w1267:errorcluster)  [unwired: 1 in]
        n872 = Close Reference(reference=w1266, error in (no error)=w1267) -> ()  [unwired: 1 out]
        n873 = Close Reference(reference=w1272, error in (no error)=w1271) -> ()  [unwired: 1 out]
        n874 = call "DATA ENCRYPT STRING FILE WRITE.vi"("error in (no error)"=w1263, "User Action"="User Pressed Setup", "main ref"=w1261) -> ("error out"=w1262:errorcluster)  [unwired: 6 in, 1 out]
      }
      frame "Error" {
        # "#CodeRecommended - If you ever change the name of this \"Error\" message, you'll need to update the name in the Check Loop Error.vi as well."
        # "#CodeRecommended - Consider creating a system for logging errors in some way. These errors are for notification purposes only. Handling of specific errors should be performed in the message frames that generated the error."
        # "Error - Display an error dialog. This message is sent by the \"Error Handler\" VIs at the end of other loops in this application."
        n875 = Variant To Data(error in=w1279, type=errorcluster {"status"=FALSE, "code"=0, "source"=""} ("error constant"), Variant=w1277) -> (data=w1275:errorcluster, error out=w1274:errorcluster)
        n876 = call <vilib>:"Simple Error Handler.vi"("error in (no error)"=w1275) -> ()  [unwired: 4 in, 5 out]
        n877 = Merge Errors(w1274) -> (w1273:errorcluster)
      }
      frame "Confirm Quit" {
        # "#CodeNeeded - If you want to provide an \"Are you sure\" dialog (or some other notification) before the application exits, place that code here. This message is typically sent from a Panel Close? event."
        # "Confirm Quit - Message that can confirm whether or not the user wants to exit the application."
        n878 = call-poly "Enqueue Message.vi"("Priority Message? (F)"=TRUE, "error in (no error)"=w1286, "Message"="Exit", "Message Queue"=w1282) -> ("error out"=w1283:errorcluster)  [unwired: 6 in, 1 out]
        n879 = Merge Errors(w1283) -> (w1284:errorcluster)
      }
      frame "Exit" {
        # "Stop the VI"
        # "Release the message queue reference"
        # "#CodeNeeded - Add any required cleanup code here. Note that if 'Exit' was called as a result of an error, an error dialog will be displayed. Add any custom error handling for an 'Exit' condition here as well."
        # "Exit - Exit the application."
        n880 = call "Fire User Event - Stop.vi"("User Event - Stop"=w1289) -> ("error out"=w1288:errorcluster)  [unwired: 10 in]
        n881 = Release Queue(queue=w1294, error in (no error)=w1287) -> (error out=w1291:errorcluster)  [unwired: 1 in, 2 out]
        n882 = Merge Errors(w1288, w1291) -> (w1290:errorcluster)
      }
      frame Default {
        # "'Default' case only runs if there is a message that isn't defined in any of the other cases.  Output a programming error."
        n883 = xnode "Error Ring"("parameter 0"=w1295) -> ("error out"=w1296:errorcluster)
      }
    }
    n884 = call "LAB-IQ Error Handler - Message Handling Loop.vi"("error in (no error)"=w591, "Message Queue"=w593) -> ("dup error in"=w592:errorcluster)  [unwired: 8 in, 1 out]
  }
  n885 = while {
    shift-right: [w1315] -> _
    shift-left: w9 -> [w1316]
    tunnel: [w1309] -> w21
    tunnel: w20 -> [w1307]
    tunnel: w7 -> [w1306]
    tunnel: w8 -> [w1305]
    stop <- w1314 stop-if-true
    # "Load  Handling Loop"
    n886 = call "Dequeue Message.vi"("error in (no error)"=w1306, "Message Queue"=w1307) -> ("error out"=w1313:errorcluster, "Message Data"=w1311:variant, "Message"=w1312:string, "dup Message Queue"=w1310:refnum<queue>)  [unwired: 6 in]
    n887 = case "Message Cases" shown="\"Exit\"" w1312 {
      selector: w1312 -> [_ _ _ _ _ w1360]
      tunnel: w1310 -> [w1317 w1328 _ w1347 w1359 _]
      tunnel: w1313 -> [w1320 w1325 w1344 w1351 w1353 _]
      tunnel: [w1321 w1329 w1338 w1349 w1355 w1361] -> w1308
      tunnel: w1316 -> [w1319 w1327 w1343 w1350 w1358 w1362]
      tunnel: [w1319 w1327 w1343 w1350 w1358 w1362] -> w1315
      tunnel: [_ _ _ _ TRUE _] -> w1314
      tunnel: w1311 -> [_ _ w1342 _ _ _]
      tunnel: w1305 -> [_ _ _ _ w1352 _]
      frame "init" {
        # "Bundle control references and a sample string value."
        # "Initialize - All initialization work should take place in this message, since other loops can potentially enqueue messages that execute immediately after this one."
        n888 = call-poly "Enqueue Message.vi"("error in (no error)"=w1320, "Message"="Load Main", "Message Queue"=w1317) -> ("error out"=w1321:errorcluster)  [unwired: 7 in, 1 out]
      }
      frame "Load Main" {
        n889 = Unbundle By Name(w1327) -> ("Main Home Screen.EXIT"=w1326:refnum<vi>)
        n890 = property class="Bool (strict)"(reference=w1326) -> (reference out=w1323:refnum<vi>, error out=w1324:errorcluster, "Value"=w1322:bool)  [unwired: 1 in]
        n891 = Close Reference(reference=w1323, error in (no error)=w1324) -> ()  [unwired: 1 out]
        n892 = case shown="False" w1322 {
          tunnel: [w1332 w1336] -> w1329
          tunnel: w1328 -> [w1331 w1335]
          tunnel: w1325 -> [w1330 w1334]
          frame True {
            n893 = call-poly "Enqueue Message.vi"("error in (no error)"=w1330, "Message"="Confirm Quit", "Message Queue"=w1331) -> ("error out"=w1332:errorcluster)  [unwired: 7 in, 1 out]
          }
          frame False {
            n894 = call-poly "Enqueue Message.vi"("error in (no error)"=w1334, "Message"="Load Main", "Message Queue"=w1335) -> ("error out"=w1336:errorcluster)  [unwired: 7 in, 1 out]
          }
        }
      }
      frame "Error" {
        # "#CodeRecommended - If you ever change the name of this \"Error\" message, you'll need to update the name in the Check Loop Error.vi as well."
        # "#CodeRecommended - Consider creating a system for logging errors in some way. These errors are for notification purposes only. Handling of specific errors should be performed in the message frames that generated the error."
        # "Error - Display an error dialog. This message is sent by the \"Error Handler\" VIs at the end of other loops in this application."
        n895 = Variant To Data(error in=w1344, type=errorcluster {"status"=FALSE, "code"=0, "source"=""} ("error constant"), Variant=w1342) -> (data=w1340:errorcluster, error out=w1339:errorcluster)
        n896 = call <vilib>:"Simple Error Handler.vi"("error in (no error)"=w1340) -> ()  [unwired: 4 in, 5 out]
        n897 = Merge Errors(w1339) -> (w1338:errorcluster)
      }
      frame "Confirm Quit" {
        # "#CodeNeeded - If you want to provide an \"Are you sure\" dialog (or some other notification) before the application exits, place that code here. This message is typically sent from a Panel Close? event."
        # "Confirm Quit - Message that can confirm whether or not the user wants to exit the application."
        n898 = call-poly "Enqueue Message.vi"("Priority Message? (F)"=TRUE, "error in (no error)"=w1351, "Message"="Exit", "Message Queue"=w1347) -> ("error out"=w1348:errorcluster)  [unwired: 6 in, 1 out]
        n899 = Merge Errors(w1348) -> (w1349:errorcluster)
      }
      frame "Exit" {
        # "Stop the VI"
        # "Release the message queue reference"
        # "#CodeNeeded - Add any required cleanup code here. Note that if 'Exit' was called as a result of an error, an error dialog will be displayed. Add any custom error handling for an 'Exit' condition here as well."
        # "Exit - Exit the application."
        n900 = call "Fire User Event - Stop.vi"("User Event - Stop"=w1352) -> ("error out"=w1354:errorcluster)  [unwired: 10 in]
        n901 = Release Queue(queue=w1359, error in (no error)=w1353) -> (error out=w1356:errorcluster)  [unwired: 1 in, 2 out]
        n902 = Merge Errors(w1354, w1356) -> (w1355:errorcluster)
      }
      frame Default {
        # "'Default' case only runs if there is a message that isn't defined in any of the other cases.  Output a programming error."
        n903 = xnode "Error Ring"("parameter 0"=w1360) -> ("error out"=w1361:errorcluster)
      }
    }
    n904 = call "LAB-IQ Error Handler - Message Handling Loop.vi"("error in (no error)"=w1308, "Message Queue"=w1310) -> ("dup error in"=w1309:errorcluster)  [unwired: 8 in, 1 out]
  }
  n905 = while {
    shift-right: [w1380] -> _
    shift-left: w9 -> [w1381]
    tunnel: [w1374] -> w18
    tunnel: w19 -> [w1372]
    tunnel: w7 -> [w1371]
    tunnel: w8 -> [w1370]
    stop <- w1379 stop-if-true
    # "Sway Motor  Handling Loop"
    n906 = call "Dequeue Message.vi"("error in (no error)"=w1371, "Message Queue"=w1372) -> ("error out"=w1378:errorcluster, "Message Data"=w1376:variant, "Message"=w1377:string, "dup Message Queue"=w1375:refnum<queue>)  [unwired: 6 in]
    n907 = case "Message Cases" shown="\"Exit\"" w1377 {
      selector: w1377 -> [_ _ _ _ _ w1425]
      tunnel: w1375 -> [w1382 w1393 _ w1412 w1424 _]
      tunnel: w1378 -> [w1385 w1390 w1409 w1416 w1418 _]
      tunnel: [w1386 w1394 w1403 w1414 w1420 w1426] -> w1373
      tunnel: w1381 -> [w1384 w1392 w1408 w1415 w1423 w1427]
      tunnel: [w1384 w1392 w1408 w1415 w1423 w1427] -> w1380
      tunnel: [_ _ _ _ TRUE _] -> w1379
      tunnel: w1376 -> [_ _ w1407 _ _ _]
      tunnel: w1370 -> [_ _ _ _ w1417 _]
      frame "init" {
        # "Bundle control references and a sample string value."
        # "Initialize - All initialization work should take place in this message, since other loops can potentially enqueue messages that execute immediately after this one."
        n908 = call-poly "Enqueue Message.vi"("error in (no error)"=w1385, "Message"="Sway Main", "Message Queue"=w1382) -> ("error out"=w1386:errorcluster)  [unwired: 7 in, 1 out]
      }
      frame "Sway Main" {
        n909 = Unbundle By Name(w1392) -> ("Main Home Screen.EXIT"=w1391:refnum<vi>)
        n910 = property class="Bool (strict)"(reference=w1391) -> (reference out=w1388:refnum<vi>, error out=w1389:errorcluster, "Value"=w1387:bool)  [unwired: 1 in]
        n911 = Close Reference(reference=w1388, error in (no error)=w1389) -> ()  [unwired: 1 out]
        n912 = case shown="False" w1387 {
          tunnel: [w1397 w1401] -> w1394
          tunnel: w1393 -> [w1396 w1400]
          tunnel: w1390 -> [w1395 w1399]
          frame True {
            n913 = call-poly "Enqueue Message.vi"("error in (no error)"=w1395, "Message"="Confirm Quit", "Message Queue"=w1396) -> ("error out"=w1397:errorcluster)  [unwired: 7 in, 1 out]
          }
          frame False {
            n914 = call-poly "Enqueue Message.vi"("error in (no error)"=w1399, "Message"="Sway Main", "Message Queue"=w1400) -> ("error out"=w1401:errorcluster)  [unwired: 7 in, 1 out]
          }
        }
      }
      frame "Error" {
        # "#CodeRecommended - If you ever change the name of this \"Error\" message, you'll need to update the name in the Check Loop Error.vi as well."
        # "#CodeRecommended - Consider creating a system for logging errors in some way. These errors are for notification purposes only. Handling of specific errors should be performed in the message frames that generated the error."
        # "Error - Display an error dialog. This message is sent by the \"Error Handler\" VIs at the end of other loops in this application."
        n915 = Variant To Data(error in=w1409, type=errorcluster {"status"=FALSE, "code"=0, "source"=""} ("error constant"), Variant=w1407) -> (data=w1405:errorcluster, error out=w1404:errorcluster)
        n916 = call <vilib>:"Simple Error Handler.vi"("error in (no error)"=w1405) -> ()  [unwired: 4 in, 5 out]
        n917 = Merge Errors(w1404) -> (w1403:errorcluster)
      }
      frame "Confirm Quit" {
        # "#CodeNeeded - If you want to provide an \"Are you sure\" dialog (or some other notification) before the application exits, place that code here. This message is typically sent from a Panel Close? event."
        # "Confirm Quit - Message that can confirm whether or not the user wants to exit the application."
        n918 = call-poly "Enqueue Message.vi"("Priority Message? (F)"=TRUE, "error in (no error)"=w1416, "Message"="Exit", "Message Queue"=w1412) -> ("error out"=w1413:errorcluster)  [unwired: 6 in, 1 out]
        n919 = Merge Errors(w1413) -> (w1414:errorcluster)
      }
      frame "Exit" {
        # "Stop the VI"
        # "Release the message queue reference"
        # "#CodeNeeded - Add any required cleanup code here. Note that if 'Exit' was called as a result of an error, an error dialog will be displayed. Add any custom error handling for an 'Exit' condition here as well."
        # "Exit - Exit the application."
        n920 = call "Fire User Event - Stop.vi"("User Event - Stop"=w1417) -> ("error out"=w1419:errorcluster)  [unwired: 10 in]
        n921 = Release Queue(queue=w1424, error in (no error)=w1418) -> (error out=w1421:errorcluster)  [unwired: 1 in, 2 out]
        n922 = Merge Errors(w1419, w1421) -> (w1420:errorcluster)
      }
      frame Default {
        # "'Default' case only runs if there is a message that isn't defined in any of the other cases.  Output a programming error."
        n923 = xnode "Error Ring"("parameter 0"=w1425) -> ("error out"=w1426:errorcluster)
      }
    }
    n924 = call "LAB-IQ Error Handler - Message Handling Loop.vi"("error in (no error)"=w1373, "Message Queue"=w1375) -> ("dup error in"=w1374:errorcluster)  [unwired: 8 in, 1 out]
  }
  n925 = while {
    shift-right: [w1445] -> _
    shift-left: w9 -> [w1446]
    tunnel: [w1439] -> w15
    tunnel: w17 -> [w1437]
    tunnel: w7 -> [w1436]
    tunnel: w8 -> [w1435]
    stop <- w1444 stop-if-true
    # "Heave Motor  Handling Loop"
    n926 = call "Dequeue Message.vi"("error in (no error)"=w1436, "Message Queue"=w1437) -> ("error out"=w1443:errorcluster, "Message Data"=w1441:variant, "Message"=w1442:string, "dup Message Queue"=w1440:refnum<queue>)  [unwired: 6 in]
    n927 = case "Message Cases" shown="\"Exit\"" w1442 {
      selector: w1442 -> [_ _ _ _ _ w1490]
      tunnel: w1440 -> [w1447 w1458 _ w1477 w1489 _]
      tunnel: w1443 -> [w1450 w1455 w1474 w1481 w1483 _]
      tunnel: [w1451 w1459 w1468 w1479 w1485 w1491] -> w1438
      tunnel: w1446 -> [w1449 w1457 w1473 w1480 w1488 w1492]
      tunnel: [w1449 w1457 w1473 w1480 w1488 w1492] -> w1445
      tunnel: [_ _ _ _ TRUE _] -> w1444
      tunnel: w1441 -> [_ _ w1472 _ _ _]
      tunnel: w1435 -> [_ _ _ _ w1482 _]
      frame "init" {
        # "Initialize - All initialization work should take place in this message, since other loops can potentially enqueue messages that execute immediately after this one."
        n928 = call-poly "Enqueue Message.vi"("error in (no error)"=w1450, "Message"="Heave Main", "Message Queue"=w1447) -> ("error out"=w1451:errorcluster)  [unwired: 7 in, 1 out]
      }
      frame "Heave Main" {
        n929 = Unbundle By Name(w1457) -> ("Main Home Screen.EXIT"=w1456:refnum<vi>)
        n930 = property class="Bool (strict)"(reference=w1456) -> (reference out=w1453:refnum<vi>, error out=w1454:errorcluster, "Value"=w1452:bool)  [unwired: 1 in]
        n931 = Close Reference(reference=w1453, error in (no error)=w1454) -> ()  [unwired: 1 out]
        n932 = case shown="False" w1452 {
          tunnel: [w1462 w1466] -> w1459
          tunnel: w1458 -> [w1461 w1465]
          tunnel: w1455 -> [w1460 w1464]
          frame True {
            n933 = call-poly "Enqueue Message.vi"("error in (no error)"=w1460, "Message"="Confirm Quit", "Message Queue"=w1461) -> ("error out"=w1462:errorcluster)  [unwired: 7 in, 1 out]
          }
          frame False {
            n934 = call-poly "Enqueue Message.vi"("error in (no error)"=w1464, "Message"="Heave Main", "Message Queue"=w1465) -> ("error out"=w1466:errorcluster)  [unwired: 7 in, 1 out]
          }
        }
      }
      frame "Error" {
        # "#CodeRecommended - If you ever change the name of this \"Error\" message, you'll need to update the name in the Check Loop Error.vi as well."
        # "#CodeRecommended - Consider creating a system for logging errors in some way. These errors are for notification purposes only. Handling of specific errors should be performed in the message frames that generated the error."
        # "Error - Display an error dialog. This message is sent by the \"Error Handler\" VIs at the end of other loops in this application."
        n935 = Variant To Data(error in=w1474, type=errorcluster {"status"=FALSE, "code"=0, "source"=""} ("error constant"), Variant=w1472) -> (data=w1470:errorcluster, error out=w1469:errorcluster)
        n936 = call <vilib>:"Simple Error Handler.vi"("error in (no error)"=w1470) -> ()  [unwired: 4 in, 5 out]
        n937 = Merge Errors(w1469) -> (w1468:errorcluster)
      }
      frame "Confirm Quit" {
        # "#CodeNeeded - If you want to provide an \"Are you sure\" dialog (or some other notification) before the application exits, place that code here. This message is typically sent from a Panel Close? event."
        # "Confirm Quit - Message that can confirm whether or not the user wants to exit the application."
        n938 = call-poly "Enqueue Message.vi"("Priority Message? (F)"=TRUE, "error in (no error)"=w1481, "Message"="Exit", "Message Queue"=w1477) -> ("error out"=w1478:errorcluster)  [unwired: 6 in, 1 out]
        n939 = Merge Errors(w1478) -> (w1479:errorcluster)
      }
      frame "Exit" {
        # "Stop the VI"
        # "Release the message queue reference"
        # "#CodeNeeded - Add any required cleanup code here. Note that if 'Exit' was called as a result of an error, an error dialog will be displayed. Add any custom error handling for an 'Exit' condition here as well."
        # "Exit - Exit the application."
        n940 = call "Fire User Event - Stop.vi"("User Event - Stop"=w1482) -> ("error out"=w1484:errorcluster)  [unwired: 10 in]
        n941 = Release Queue(queue=w1489, error in (no error)=w1483) -> (error out=w1486:errorcluster)  [unwired: 1 in, 2 out]
        n942 = Merge Errors(w1484, w1486) -> (w1485:errorcluster)
      }
      frame Default {
        # "'Default' case only runs if there is a message that isn't defined in any of the other cases.  Output a programming error."
        n943 = xnode "Error Ring"("parameter 0"=w1490) -> ("error out"=w1491:errorcluster)
      }
    }
    n944 = call "LAB-IQ Error Handler - Message Handling Loop.vi"("error in (no error)"=w1438, "Message Queue"=w1440) -> ("dup error in"=w1439:errorcluster)  [unwired: 8 in, 1 out]
  }
  n945 = while {
    shift-right: [w1510] -> _
    shift-left: w9 -> [w1511]
    tunnel: [w1504] -> w14
    tunnel: w16 -> [w1502]
    tunnel: w7 -> [w1501]
    tunnel: w8 -> [w1500]
    stop <- w1509 stop-if-true
    # "Temperature  Handling Loop"
    n946 = call "Dequeue Message.vi"("error in (no error)"=w1501, "Message Queue"=w1502) -> ("error out"=w1508:errorcluster, "Message Data"=w1506:variant, "Message"=w1507:string, "dup Message Queue"=w1505:refnum<queue>)  [unwired: 6 in]
    n947 = case "Message Cases" shown="\"Temperature Main\"" w1507 {
      selector: w1507 -> [_ _ _ _ _ w1555]
      tunnel: w1505 -> [w1512 w1523 _ w1542 w1554 _]
      tunnel: w1508 -> [w1515 w1520 w1539 w1546 w1548 _]
      tunnel: [w1516 w1524 w1533 w1544 w1550 w1556] -> w1503
      tunnel: w1511 -> [w1514 w1522 w1538 w1545 w1553 w1557]
      tunnel: [w1514 w1522 w1538 w1545 w1553 w1557] -> w1510
      tunnel: [_ _ _ _ TRUE _] -> w1509
      tunnel: w1506 -> [_ _ w1537 _ _ _]
      tunnel: w1500 -> [_ _ _ _ w1547 _]
      frame "init" {
        # "Initialize - All initialization work should take place in this message, since other loops can potentially enqueue messages that execute immediately after this one."
        n948 = call-poly "Enqueue Message.vi"("error in (no error)"=w1515, "Message"="Temperature Main", "Message Queue"=w1512) -> ("error out"=w1516:errorcluster)  [unwired: 7 in, 1 out]
      }
      frame "Temperature Main" {
        n949 = Unbundle By Name(w1522) -> ("Main Home Screen.EXIT"=w1521:refnum<vi>)
        n950 = property class="Bool (strict)"(reference=w1521) -> (reference out=w1518:refnum<vi>, error out=w1519:errorcluster, "Value"=w1517:bool)  [unwired: 1 in]
        n951 = case shown="False" w1517 {
          tunnel: [w1527 w1531] -> w1524
          tunnel: w1523 -> [w1526 w1530]
          tunnel: w1520 -> [w1525 w1529]
          frame True {
            n952 = call-poly "Enqueue Message.vi"("error in (no error)"=w1525, "Message"="Confirm Quit", "Message Queue"=w1526) -> ("error out"=w1527:errorcluster)  [unwired: 7 in, 1 out]
          }
          frame False {
            n953 = call-poly "Enqueue Message.vi"("error in (no error)"=w1529, "Message"="Temperature Main", "Message Queue"=w1530) -> ("error out"=w1531:errorcluster)  [unwired: 7 in, 1 out]
          }
        }
        n954 = Close Reference(reference=w1518, error in (no error)=w1519) -> ()  [unwired: 1 out]
      }
      frame "Error" {
        # "#CodeRecommended - If you ever change the name of this \"Error\" message, you'll need to update the name in the Check Loop Error.vi as well."
        # "#CodeRecommended - Consider creating a system for logging errors in some way. These errors are for notification purposes only. Handling of specific errors should be performed in the message frames that generated the error."
        # "Error - Display an error dialog. This message is sent by the \"Error Handler\" VIs at the end of other loops in this application."
        n955 = Variant To Data(error in=w1539, type=errorcluster {"status"=FALSE, "code"=0, "source"=""} ("error constant"), Variant=w1537) -> (data=w1535:errorcluster, error out=w1534:errorcluster)
        n956 = call <vilib>:"Simple Error Handler.vi"("error in (no error)"=w1535) -> ()  [unwired: 4 in, 5 out]
        n957 = Merge Errors(w1534) -> (w1533:errorcluster)
      }
      frame "Confirm Quit" {
        # "#CodeNeeded - If you want to provide an \"Are you sure\" dialog (or some other notification) before the application exits, place that code here. This message is typically sent from a Panel Close? event."
        # "Confirm Quit - Message that can confirm whether or not the user wants to exit the application."
        n958 = call-poly "Enqueue Message.vi"("Priority Message? (F)"=TRUE, "error in (no error)"=w1546, "Message"="Exit", "Message Queue"=w1542) -> ("error out"=w1543:errorcluster)  [unwired: 6 in, 1 out]
        n959 = Merge Errors(w1543) -> (w1544:errorcluster)
      }
      frame "Exit" {
        # "Stop the VI"
        # "Release the message queue reference"
        # "#CodeNeeded - Add any required cleanup code here. Note that if 'Exit' was called as a result of an error, an error dialog will be displayed. Add any custom error handling for an 'Exit' condition here as well."
        # "Exit - Exit the application."
        n960 = call "Fire User Event - Stop.vi"("User Event - Stop"=w1547) -> ("error out"=w1549:errorcluster)  [unwired: 10 in]
        n961 = Release Queue(queue=w1554, error in (no error)=w1548) -> (error out=w1551:errorcluster)  [unwired: 1 in, 2 out]
        n962 = Merge Errors(w1549, w1551) -> (w1550:errorcluster)
      }
      frame Default {
        # "'Default' case only runs if there is a message that isn't defined in any of the other cases.  Output a programming error."
        n963 = xnode "Error Ring"("parameter 0"=w1555) -> ("error out"=w1556:errorcluster)
      }
    }
    n964 = call "LAB-IQ Error Handler - Message Handling Loop.vi"("error in (no error)"=w1503, "Message Queue"=w1505) -> ("dup error in"=w1504:errorcluster)  [unwired: 8 in, 1 out]
  }
  n965 = while {
    shift-right: [w1575] -> _
    shift-left: w9 -> [w1576]
    tunnel: [w1569] -> _
    tunnel: w13 -> [w1567]
    tunnel: w7 -> [w1566]
    tunnel: w8 -> [w1565]
    stop <- w1574 stop-if-true
    # "Ramp Motor  Handling Loop"
    n966 = call "Dequeue Message.vi"("error in (no error)"=w1566, "Message Queue"=w1567) -> ("error out"=w1573:errorcluster, "Message Data"=w1571:variant, "Message"=w1572:string, "dup Message Queue"=w1570:refnum<queue>)  [unwired: 6 in]
    n967 = case "Message Cases" shown="\"init\"" w1572 {
      selector: w1572 -> [_ _ _ _ _ w1620]
      tunnel: w1570 -> [w1577 w1588 _ w1607 w1619 _]
      tunnel: w1573 -> [w1580 w1585 w1604 w1611 w1613 _]
      tunnel: [w1581 w1589 w1598 w1609 w1615 w1621] -> w1568
      tunnel: w1576 -> [w1579 w1587 w1603 w1610 w1618 w1622]
      tunnel: [w1579 w1587 w1603 w1610 w1618 w1622] -> w1575
      tunnel: [_ _ _ _ TRUE _] -> w1574
      tunnel: w1571 -> [_ _ w1602 _ _ _]
      tunnel: w1565 -> [_ _ _ _ w1612 _]
      frame "init" {
        # "Initialize - All initialization work should take place in this message, since other loops can potentially enqueue messages that execute immediately after this one."
        n968 = call-poly "Enqueue Message.vi"("error in (no error)"=w1580, "Message"="Ramp Main", "Message Queue"=w1577) -> ("error out"=w1581:errorcluster)  [unwired: 7 in, 1 out]
      }
      frame "Ramp Main" {
        n969 = Unbundle By Name(w1587) -> ("Main Home Screen.EXIT"=w1586:refnum<vi>)
        n970 = property class="Bool (strict)"(reference=w1586) -> (reference out=w1583:refnum<vi>, error out=w1584:errorcluster, "Value"=w1582:bool)  [unwired: 1 in]
        n971 = case shown="False" w1582 {
          tunnel: [w1592 w1596] -> w1589
          tunnel: w1588 -> [w1591 w1595]
          tunnel: w1585 -> [w1590 w1594]
          frame True {
            n972 = call-poly "Enqueue Message.vi"("error in (no error)"=w1590, "Message"="Confirm Quit", "Message Queue"=w1591) -> ("error out"=w1592:errorcluster)  [unwired: 7 in, 1 out]
          }
          frame False {
            n973 = call-poly "Enqueue Message.vi"("error in (no error)"=w1594, "Message"="Ramp Main", "Message Queue"=w1595) -> ("error out"=w1596:errorcluster)  [unwired: 7 in, 1 out]
          }
        }
        n974 = Close Reference(reference=w1583, error in (no error)=w1584) -> ()  [unwired: 1 out]
      }
      frame "Error" {
        # "#CodeRecommended - If you ever change the name of this \"Error\" message, you'll need to update the name in the Check Loop Error.vi as well."
        # "#CodeRecommended - Consider creating a system for logging errors in some way. These errors are for notification purposes only. Handling of specific errors should be performed in the message frames that generated the error."
        # "Error - Display an error dialog. This message is sent by the \"Error Handler\" VIs at the end of other loops in this application."
        n975 = Variant To Data(error in=w1604, type=errorcluster {"status"=FALSE, "code"=0, "source"=""} ("error constant"), Variant=w1602) -> (data=w1600:errorcluster, error out=w1599:errorcluster)
        n976 = call <vilib>:"Simple Error Handler.vi"("error in (no error)"=w1600) -> ()  [unwired: 4 in, 5 out]
        n977 = Merge Errors(w1599) -> (w1598:errorcluster)
      }
      frame "Confirm Quit" {
        # "#CodeNeeded - If you want to provide an \"Are you sure\" dialog (or some other notification) before the application exits, place that code here. This message is typically sent from a Panel Close? event."
        # "Confirm Quit - Message that can confirm whether or not the user wants to exit the application."
        n978 = call-poly "Enqueue Message.vi"("Priority Message? (F)"=TRUE, "error in (no error)"=w1611, "Message"="Exit", "Message Queue"=w1607) -> ("error out"=w1608:errorcluster)  [unwired: 6 in, 1 out]
        n979 = Merge Errors(w1608) -> (w1609:errorcluster)
      }
      frame "Exit" {
        # "Stop the VI"
        # "Release the message queue reference"
        # "#CodeNeeded - Add any required cleanup code here. Note that if 'Exit' was called as a result of an error, an error dialog will be displayed. Add any custom error handling for an 'Exit' condition here as well."
        # "Exit - Exit the application."
        n980 = call "Fire User Event - Stop.vi"("User Event - Stop"=w1612) -> ("error out"=w1614:errorcluster)  [unwired: 10 in]
        n981 = Release Queue(queue=w1619, error in (no error)=w1613) -> (error out=w1616:errorcluster)  [unwired: 1 in, 2 out]
        n982 = Merge Errors(w1614, w1616) -> (w1615:errorcluster)
      }
      frame Default {
        # "'Default' case only runs if there is a message that isn't defined in any of the other cases.  Output a programming error."
        n983 = xnode "Error Ring"("parameter 0"=w1620) -> ("error out"=w1621:errorcluster)
      }
    }
    n984 = call "LAB-IQ Error Handler - Message Handling Loop.vi"("error in (no error)"=w1568, "Message Queue"=w1570) -> ("dup error in"=w1569:errorcluster)  [unwired: 8 in, 1 out]
  }
  n985 = while {
    shift-right: [w1640] -> _
    shift-left: w9 -> [w1641]
    tunnel: [w1634] -> _
    tunnel: w12 -> [w1632]
    tunnel: w7 -> [w1631]
    tunnel: w8 -> [w1630]
    stop <- w1639 stop-if-true
    # "ECR  Handling Loop"
    n986 = call "Dequeue Message.vi"("error in (no error)"=w1631, "Message Queue"=w1632) -> ("error out"=w1638:errorcluster, "Message Data"=w1636:variant, "Message"=w1637:string, "dup Message Queue"=w1635:refnum<queue>)  [unwired: 6 in]
    n987 = case "Message Cases" shown="\"ECR Main\"" w1637 {
      selector: w1637 -> [_ _ _ _ _ w1685]
      tunnel: w1635 -> [w1642 w1653 _ w1672 w1684 _]
      tunnel: w1638 -> [w1645 w1650 w1669 w1676 w1678 _]
      tunnel: [w1646 w1654 w1663 w1674 w1680 w1686] -> w1633
      tunnel: w1641 -> [w1644 w1652 w1668 w1675 w1683 w1687]
      tunnel: [w1644 w1652 w1668 w1675 w1683 w1687] -> w1640
      tunnel: [_ _ _ _ TRUE _] -> w1639
      tunnel: w1636 -> [_ _ w1667 _ _ _]
      tunnel: w1630 -> [_ _ _ _ w1677 _]
      frame "init" {
        # "Initialize - All initialization work should take place in this message, since other loops can potentially enqueue messages that execute immediately after this one."
        n988 = call-poly "Enqueue Message.vi"("error in (no error)"=w1645, "Message"="ECR Main", "Message Queue"=w1642) -> ("error out"=w1646:errorcluster)  [unwired: 7 in, 1 out]
      }
      frame "ECR Main" {
        n989 = Unbundle By Name(w1652) -> ("Main Home Screen.EXIT"=w1651:refnum<vi>)
        n990 = property class="Bool (strict)"(reference=w1651) -> (reference out=w1648:refnum<vi>, error out=w1649:errorcluster, "Value"=w1647:bool)  [unwired: 1 in]
        n991 = case shown="False" w1647 {
          tunnel: [w1657 w1661] -> w1654
          tunnel: w1653 -> [w1656 w1660]
          tunnel: w1650 -> [w1655 w1659]
          frame True {
            n992 = call-poly "Enqueue Message.vi"("error in (no error)"=w1655, "Message"="Confirm Quit", "Message Queue"=w1656) -> ("error out"=w1657:errorcluster)  [unwired: 7 in, 1 out]
          }
          frame False {
            n993 = call-poly "Enqueue Message.vi"("error in (no error)"=w1659, "Message"="ECR Main", "Message Queue"=w1660) -> ("error out"=w1661:errorcluster)  [unwired: 7 in, 1 out]
          }
        }
        n994 = Close Reference(reference=w1648, error in (no error)=w1649) -> ()  [unwired: 1 out]
      }
      frame "Error" {
        # "#CodeRecommended - If you ever change the name of this \"Error\" message, you'll need to update the name in the Check Loop Error.vi as well."
        # "#CodeRecommended - Consider creating a system for logging errors in some way. These errors are for notification purposes only. Handling of specific errors should be performed in the message frames that generated the error."
        # "Error - Display an error dialog. This message is sent by the \"Error Handler\" VIs at the end of other loops in this application."
        n995 = Variant To Data(error in=w1669, type=errorcluster {"status"=FALSE, "code"=0, "source"=""} ("error constant"), Variant=w1667) -> (data=w1665:errorcluster, error out=w1664:errorcluster)
        n996 = call <vilib>:"Simple Error Handler.vi"("error in (no error)"=w1665) -> ()  [unwired: 4 in, 5 out]
        n997 = Merge Errors(w1664) -> (w1663:errorcluster)
      }
      frame "Confirm Quit" {
        # "#CodeNeeded - If you want to provide an \"Are you sure\" dialog (or some other notification) before the application exits, place that code here. This message is typically sent from a Panel Close? event."
        # "Confirm Quit - Message that can confirm whether or not the user wants to exit the application."
        n998 = call-poly "Enqueue Message.vi"("Priority Message? (F)"=TRUE, "error in (no error)"=w1676, "Message"="Exit", "Message Queue"=w1672) -> ("error out"=w1673:errorcluster)  [unwired: 6 in, 1 out]
        n999 = Merge Errors(w1673) -> (w1674:errorcluster)
      }
      frame "Exit" {
        # "Stop the VI"
        # "Release the message queue reference"
        # "#CodeNeeded - Add any required cleanup code here. Note that if 'Exit' was called as a result of an error, an error dialog will be displayed. Add any custom error handling for an 'Exit' condition here as well."
        # "Exit - Exit the application."
        n1000 = call "Fire User Event - Stop.vi"("User Event - Stop"=w1677) -> ("error out"=w1679:errorcluster)  [unwired: 10 in]
        n1001 = Release Queue(queue=w1684, error in (no error)=w1678) -> (error out=w1681:errorcluster)  [unwired: 1 in, 2 out]
        n1002 = Merge Errors(w1679, w1681) -> (w1680:errorcluster)
      }
      frame Default {
        # "'Default' case only runs if there is a message that isn't defined in any of the other cases.  Output a programming error."
        n1003 = xnode "Error Ring"("parameter 0"=w1685) -> ("error out"=w1686:errorcluster)
      }
    }
    n1004 = call "LAB-IQ Error Handler - Message Handling Loop.vi"("error in (no error)"=w1633, "Message Queue"=w1635) -> ("dup error in"=w1634:errorcluster)  [unwired: 8 in, 1 out]
  }
  n1005 = while {
    shift-right: [w1705] -> _
    shift-left: w9 -> [w1706]
    tunnel: [w1699] -> _
    tunnel: w11 -> [w1697]
    tunnel: w7 -> [w1696]
    tunnel: w8 -> [w1695]
    stop <- w1704 stop-if-true
    # "Humidity  Handling Loop"
    n1006 = call "Dequeue Message.vi"("error in (no error)"=w1696, "Message Queue"=w1697) -> ("error out"=w1703:errorcluster, "Message Data"=w1701:variant, "Message"=w1702:string, "dup Message Queue"=w1700:refnum<queue>)  [unwired: 6 in]
    n1007 = case "Message Cases" shown="\"Humidity Main\"" w1702 {
      selector: w1702 -> [_ _ _ _ _ w1750]
      tunnel: w1700 -> [w1707 w1718 _ w1737 w1749 _]
      tunnel: w1703 -> [w1710 w1715 w1734 w1741 w1743 _]
      tunnel: [w1711 w1719 w1728 w1739 w1745 w1751] -> w1698
      tunnel: w1706 -> [w1709 w1717 w1733 w1740 w1748 w1752]
      tunnel: [w1709 w1717 w1733 w1740 w1748 w1752] -> w1705
      tunnel: [_ _ _ _ TRUE _] -> w1704
      tunnel: w1701 -> [_ _ w1732 _ _ _]
      tunnel: w1695 -> [_ _ _ _ w1742 _]
      frame "init" {
        # "Initialize - All initialization work should take place in this message, since other loops can potentially enqueue messages that execute immediately after this one."
        n1008 = call-poly "Enqueue Message.vi"("error in (no error)"=w1710, "Message"="Humidity Main", "Message Queue"=w1707) -> ("error out"=w1711:errorcluster)  [unwired: 7 in, 1 out]
      }
      frame "Humidity Main" {
        n1009 = Unbundle By Name(w1717) -> ("Main Home Screen.EXIT"=w1716:refnum<vi>)
        n1010 = property class="Bool (strict)"(reference=w1716) -> (reference out=w1713:refnum<vi>, error out=w1714:errorcluster, "Value"=w1712:bool)  [unwired: 1 in]
        n1011 = case shown="False" w1712 {
          tunnel: [w1722 w1726] -> w1719
          tunnel: w1718 -> [w1721 w1725]
          tunnel: w1715 -> [w1720 w1724]
          frame True {
            n1012 = call-poly "Enqueue Message.vi"("error in (no error)"=w1720, "Message"="Confirm Quit", "Message Queue"=w1721) -> ("error out"=w1722:errorcluster)  [unwired: 7 in, 1 out]
          }
          frame False {
            n1013 = call-poly "Enqueue Message.vi"("error in (no error)"=w1724, "Message"="Humidity Main", "Message Queue"=w1725) -> ("error out"=w1726:errorcluster)  [unwired: 7 in, 1 out]
          }
        }
        n1014 = Close Reference(reference=w1713, error in (no error)=w1714) -> ()  [unwired: 1 out]
      }
      frame "Error" {
        # "#CodeRecommended - If you ever change the name of this \"Error\" message, you'll need to update the name in the Check Loop Error.vi as well."
        # "#CodeRecommended - Consider creating a system for logging errors in some way. These errors are for notification purposes only. Handling of specific errors should be performed in the message frames that generated the error."
        # "Error - Display an error dialog. This message is sent by the \"Error Handler\" VIs at the end of other loops in this application."
        n1015 = Variant To Data(error in=w1734, type=errorcluster {"status"=FALSE, "code"=0, "source"=""} ("error constant"), Variant=w1732) -> (data=w1730:errorcluster, error out=w1729:errorcluster)
        n1016 = call <vilib>:"Simple Error Handler.vi"("error in (no error)"=w1730) -> ()  [unwired: 4 in, 5 out]
        n1017 = Merge Errors(w1729) -> (w1728:errorcluster)
      }
      frame "Confirm Quit" {
        # "#CodeNeeded - If you want to provide an \"Are you sure\" dialog (or some other notification) before the application exits, place that code here. This message is typically sent from a Panel Close? event."
        # "Confirm Quit - Message that can confirm whether or not the user wants to exit the application."
        n1018 = call-poly "Enqueue Message.vi"("Priority Message? (F)"=TRUE, "error in (no error)"=w1741, "Message"="Exit", "Message Queue"=w1737) -> ("error out"=w1738:errorcluster)  [unwired: 6 in, 1 out]
        n1019 = Merge Errors(w1738) -> (w1739:errorcluster)
      }
      frame "Exit" {
        # "Stop the VI"
        # "Release the message queue reference"
        # "#CodeNeeded - Add any required cleanup code here. Note that if 'Exit' was called as a result of an error, an error dialog will be displayed. Add any custom error handling for an 'Exit' condition here as well."
        # "Exit - Exit the application."
        n1020 = call "Fire User Event - Stop.vi"("User Event - Stop"=w1742) -> ("error out"=w1744:errorcluster)  [unwired: 10 in]
        n1021 = Release Queue(queue=w1749, error in (no error)=w1743) -> (error out=w1746:errorcluster)  [unwired: 1 in, 2 out]
        n1022 = Merge Errors(w1744, w1746) -> (w1745:errorcluster)
      }
      frame Default {
        # "'Default' case only runs if there is a message that isn't defined in any of the other cases.  Output a programming error."
        n1023 = xnode "Error Ring"("parameter 0"=w1750) -> ("error out"=w1751:errorcluster)
      }
    }
    n1024 = call "LAB-IQ Error Handler - Message Handling Loop.vi"("error in (no error)"=w1698, "Message Queue"=w1700) -> ("dup error in"=w1699:errorcluster)  [unwired: 8 in, 1 out]
  }
  n1025 = while {
    shift-right: [w1770] -> _
    shift-left: w9 -> [w1771]
    tunnel: [w1764] -> _
    tunnel: w10 -> [w1762]
    tunnel: w7 -> [w1761]
    tunnel: w8 -> [w1760]
    stop <- w1769 stop-if-true
    # "Program  Handling Loop"
    n1026 = call "Dequeue Message.vi"("error in (no error)"=w1761, "Message Queue"=w1762) -> ("error out"=w1768:errorcluster, "Message Data"=w1766:variant, "Message"=w1767:string, "dup Message Queue"=w1765:refnum<queue>)  [unwired: 6 in]
    n1027 = case "Message Cases" shown="Default" w1767 {
      selector: w1767 -> [_ _ _ _ _ w1815]
      tunnel: w1765 -> [w1772 w1783 _ w1802 w1814 _]
      tunnel: w1768 -> [w1775 w1780 w1799 w1806 w1808 _]
      tunnel: [w1776 w1784 w1793 w1804 w1810 w1816] -> w1763
      tunnel: w1771 -> [w1774 w1782 w1798 w1805 w1813 w1817]
      tunnel: [w1774 w1782 w1798 w1805 w1813 w1817] -> w1770
      tunnel: [_ _ _ _ TRUE _] -> w1769
      tunnel: w1766 -> [_ _ w1797 _ _ _]
      tunnel: w1760 -> [_ _ _ _ w1807 _]
      frame "init" {
        # "Initialize - All initialization work should take place in this message, since other loops can potentially enqueue messages that execute immediately after this one."
        n1028 = call-poly "Enqueue Message.vi"("error in (no error)"=w1775, "Message"="Program Main", "Message Queue"=w1772) -> ("error out"=w1776:errorcluster)  [unwired: 7 in, 1 out]
      }
      frame "Program Main" {
        n1029 = Unbundle By Name(w1782) -> ("Main Home Screen.EXIT"=w1781:refnum<vi>)
        n1030 = property class="Bool (strict)"(reference=w1781) -> (reference out=w1778:refnum<vi>, error out=w1779:errorcluster, "Value"=w1777:bool)  [unwired: 1 in]
        n1031 = case shown="False" w1777 {
          tunnel: [w1787 w1791] -> w1784
          tunnel: w1783 -> [w1786 w1790]
          tunnel: w1780 -> [w1785 w1789]
          frame True {
            n1032 = call-poly "Enqueue Message.vi"("error in (no error)"=w1785, "Message"="Confirm Quit", "Message Queue"=w1786) -> ("error out"=w1787:errorcluster)  [unwired: 7 in, 1 out]
          }
          frame False {
            n1033 = call-poly "Enqueue Message.vi"("error in (no error)"=w1789, "Message"="Program Main", "Message Queue"=w1790) -> ("error out"=w1791:errorcluster)  [unwired: 7 in, 1 out]
          }
        }
        n1034 = Close Reference(reference=w1778, error in (no error)=w1779) -> ()  [unwired: 1 out]
      }
      frame "Error" {
        # "#CodeRecommended - If you ever change the name of this \"Error\" message, you'll need to update the name in the Check Loop Error.vi as well."
        # "#CodeRecommended - Consider creating a system for logging errors in some way. These errors are for notification purposes only. Handling of specific errors should be performed in the message frames that generated the error."
        # "Error - Display an error dialog. This message is sent by the \"Error Handler\" VIs at the end of other loops in this application."
        n1035 = Variant To Data(error in=w1799, type=errorcluster {"status"=FALSE, "code"=0, "source"=""} ("error constant"), Variant=w1797) -> (data=w1795:errorcluster, error out=w1794:errorcluster)
        n1036 = call <vilib>:"Simple Error Handler.vi"("error in (no error)"=w1795) -> ()  [unwired: 4 in, 5 out]
        n1037 = Merge Errors(w1794) -> (w1793:errorcluster)
      }
      frame "Confirm Quit" {
        # "#CodeNeeded - If you want to provide an \"Are you sure\" dialog (or some other notification) before the application exits, place that code here. This message is typically sent from a Panel Close? event."
        # "Confirm Quit - Message that can confirm whether or not the user wants to exit the application."
        n1038 = call-poly "Enqueue Message.vi"("Priority Message? (F)"=TRUE, "error in (no error)"=w1806, "Message"="Exit", "Message Queue"=w1802) -> ("error out"=w1803:errorcluster)  [unwired: 6 in, 1 out]
        n1039 = Merge Errors(w1803) -> (w1804:errorcluster)
      }
      frame "Exit" {
        # "Stop the VI"
        # "Release the message queue reference"
        # "#CodeNeeded - Add any required cleanup code here. Note that if 'Exit' was called as a result of an error, an error dialog will be displayed. Add any custom error handling for an 'Exit' condition here as well."
        # "Exit - Exit the application."
        n1040 = call "Fire User Event - Stop.vi"("User Event - Stop"=w1807) -> ("error out"=w1809:errorcluster)  [unwired: 10 in]
        n1041 = Release Queue(queue=w1814, error in (no error)=w1808) -> (error out=w1811:errorcluster)  [unwired: 1 in, 2 out]
        n1042 = Merge Errors(w1809, w1811) -> (w1810:errorcluster)
      }
      frame Default {
        # "'Default' case only runs if there is a message that isn't defined in any of the other cases.  Output a programming error."
        n1043 = xnode "Error Ring"("parameter 0"=w1815) -> ("error out"=w1816:errorcluster)
      }
    }
    n1044 = call "LAB-IQ Error Handler - Message Handling Loop.vi"("error in (no error)"=w1763, "Message Queue"=w1765) -> ("dup error in"=w1764:errorcluster)  [unwired: 8 in, 1 out]
  }
  n1045 = while {
    shift-right: [w1835] -> _
    shift-left: w9 -> [w1836]
    tunnel: [w1829] -> _
    tunnel: w6 -> [w1827]
    tunnel: w7 -> [w1826]
    tunnel: w8 -> [w1825]
    stop <- w1834 stop-if-true
    # "Monitor  Handling Loop"
    n1046 = call "Dequeue Message.vi"("error in (no error)"=w1826, "Message Queue"=w1827) -> ("error out"=w1833:errorcluster, "Message Data"=w1831:variant, "Message"=w1832:string, "dup Message Queue"=w1830:refnum<queue>)  [unwired: 6 in]
    n1047 = case "Message Cases" shown="\"Monitor Main\"" w1832 {
      selector: w1832 -> [_ _ _ _ _ w1880]
      tunnel: w1830 -> [w1837 w1848 _ w1867 w1879 _]
      tunnel: w1833 -> [w1840 w1845 w1864 w1871 w1873 _]
      tunnel: [w1841 w1849 w1858 w1869 w1875 w1881] -> w1828
      tunnel: w1836 -> [w1839 w1847 w1863 w1870 w1878 w1882]
      tunnel: [w1839 w1847 w1863 w1870 w1878 w1882] -> w1835
      tunnel: [_ _ _ _ TRUE _] -> w1834
      tunnel: w1831 -> [_ _ w1862 _ _ _]
      tunnel: w1825 -> [_ _ _ _ w1872 _]
      frame "init" {
        # "Initialize - All initialization work should take place in this message, since other loops can potentially enqueue messages that execute immediately after this one."
        n1048 = call-poly "Enqueue Message.vi"("error in (no error)"=w1840, "Message"="Monitor Main", "Message Queue"=w1837) -> ("error out"=w1841:errorcluster)  [unwired: 7 in, 1 out]
      }
      frame "Monitor Main" {
        n1049 = Unbundle By Name(w1847) -> ("Main Home Screen.EXIT"=w1846:refnum<vi>)
        n1050 = property class="Bool (strict)"(reference=w1846) -> (reference out=w1843:refnum<vi>, error out=w1844:errorcluster, "Value"=w1842:bool)  [unwired: 1 in]
        n1051 = case shown="False" w1842 {
          tunnel: [w1852 w1856] -> w1849
          tunnel: w1848 -> [w1851 w1855]
          tunnel: w1845 -> [w1850 w1854]
          frame True {
            n1052 = call-poly "Enqueue Message.vi"("error in (no error)"=w1850, "Message"="Confirm Quit", "Message Queue"=w1851) -> ("error out"=w1852:errorcluster)  [unwired: 7 in, 1 out]
          }
          frame False {
            n1053 = call-poly "Enqueue Message.vi"("error in (no error)"=w1854, "Message"="Monitor Main", "Message Queue"=w1855) -> ("error out"=w1856:errorcluster)  [unwired: 7 in, 1 out]
          }
        }
        n1054 = Close Reference(reference=w1843, error in (no error)=w1844) -> ()  [unwired: 1 out]
      }
      frame "Error" {
        # "#CodeRecommended - If you ever change the name of this \"Error\" message, you'll need to update the name in the Check Loop Error.vi as well."
        # "#CodeRecommended - Consider creating a system for logging errors in some way. These errors are for notification purposes only. Handling of specific errors should be performed in the message frames that generated the error."
        # "Error - Display an error dialog. This message is sent by the \"Error Handler\" VIs at the end of other loops in this application."
        n1055 = Variant To Data(error in=w1864, type=errorcluster {"status"=FALSE, "code"=0, "source"=""} ("error constant"), Variant=w1862) -> (data=w1860:errorcluster, error out=w1859:errorcluster)
        n1056 = call <vilib>:"Simple Error Handler.vi"("error in (no error)"=w1860) -> ()  [unwired: 4 in, 5 out]
        n1057 = Merge Errors(w1859) -> (w1858:errorcluster)
      }
      frame "Confirm Quit" {
        # "#CodeNeeded - If you want to provide an \"Are you sure\" dialog (or some other notification) before the application exits, place that code here. This message is typically sent from a Panel Close? event."
        # "Confirm Quit - Message that can confirm whether or not the user wants to exit the application."
        n1058 = call-poly "Enqueue Message.vi"("Priority Message? (F)"=TRUE, "error in (no error)"=w1871, "Message"="Exit", "Message Queue"=w1867) -> ("error out"=w1868:errorcluster)  [unwired: 6 in, 1 out]
        n1059 = Merge Errors(w1868) -> (w1869:errorcluster)
      }
      frame "Exit" {
        # "Stop the VI"
        # "Release the message queue reference"
        # "#CodeNeeded - Add any required cleanup code here. Note that if 'Exit' was called as a result of an error, an error dialog will be displayed. Add any custom error handling for an 'Exit' condition here as well."
        # "Exit - Exit the application."
        n1060 = call "Fire User Event - Stop.vi"("User Event - Stop"=w1872) -> ("error out"=w1874:errorcluster)  [unwired: 10 in]
        n1061 = Release Queue(queue=w1879, error in (no error)=w1873) -> (error out=w1876:errorcluster)  [unwired: 1 in, 2 out]
        n1062 = Merge Errors(w1874, w1876) -> (w1875:errorcluster)
      }
      frame Default {
        # "'Default' case only runs if there is a message that isn't defined in any of the other cases.  Output a programming error."
        n1063 = xnode "Error Ring"("parameter 0"=w1880) -> ("error out"=w1881:errorcluster)
      }
    }
    n1064 = call "LAB-IQ Error Handler - Message Handling Loop.vi"("error in (no error)"=w1828, "Message Queue"=w1830) -> ("dup error in"=w1829:errorcluster)  [unwired: 8 in, 1 out]
  }
  n1065 = while {
    shift-right: [w1900] -> _
    shift-left: w9 -> [w1901]
    tunnel: [w1894] -> _
    tunnel: w5 -> [w1892]
    tunnel: w7 -> [w1891]
    tunnel: w8 -> [w1890]
    stop <- w1899 stop-if-true
    # "Load Pid  Handling Loop"
    n1066 = call "Dequeue Message.vi"("error in (no error)"=w1891, "Message Queue"=w1892) -> ("error out"=w1898:errorcluster, "Message Data"=w1896:variant, "Message"=w1897:string, "dup Message Queue"=w1895:refnum<queue>)  [unwired: 6 in]
    n1067 = case "Message Cases" shown="\"Load Pid Main\"" w1897 {
      selector: w1897 -> [_ _ _ _ _ w1945]
      tunnel: w1895 -> [w1902 w1913 _ w1932 w1944 _]
      tunnel: w1898 -> [w1905 w1910 w1929 w1936 w1938 _]
      tunnel: [w1906 w1914 w1923 w1934 w1940 w1946] -> w1893
      tunnel: w1901 -> [w1904 w1912 w1928 w1935 w1943 w1947]
      tunnel: [w1904 w1912 w1928 w1935 w1943 w1947] -> w1900
      tunnel: [_ _ _ _ TRUE _] -> w1899
      tunnel: w1896 -> [_ _ w1927 _ _ _]
      tunnel: w1890 -> [_ _ _ _ w1937 _]
      frame "init" {
        # "Initialize - All initialization work should take place in this message, since other loops can potentially enqueue messages that execute immediately after this one."
        n1068 = call-poly "Enqueue Message.vi"("error in (no error)"=w1905, "Message"="Load Pid Main", "Message Queue"=w1902) -> ("error out"=w1906:errorcluster)  [unwired: 7 in, 1 out]
      }
      frame "Load Pid Main" {
        n1069 = Unbundle By Name(w1912) -> ("Main Home Screen.EXIT"=w1911:refnum<vi>)
        n1070 = property class="Bool (strict)"(reference=w1911) -> (reference out=w1908:refnum<vi>, error out=w1909:errorcluster, "Value"=w1907:bool)  [unwired: 1 in]
        n1071 = case shown="False" w1907 {
          tunnel: [w1917 w1921] -> w1914
          tunnel: w1913 -> [w1916 w1920]
          tunnel: w1910 -> [w1915 w1919]
          frame True {
            n1072 = call-poly "Enqueue Message.vi"("error in (no error)"=w1915, "Message"="Confirm Quit", "Message Queue"=w1916) -> ("error out"=w1917:errorcluster)  [unwired: 7 in, 1 out]
          }
          frame False {
            n1073 = call-poly "Enqueue Message.vi"("error in (no error)"=w1919, "Message"="Load Pid Main", "Message Queue"=w1920) -> ("error out"=w1921:errorcluster)  [unwired: 7 in, 1 out]
          }
        }
        n1074 = Close Reference(reference=w1908, error in (no error)=w1909) -> ()  [unwired: 1 out]
      }
      frame "Error" {
        # "#CodeRecommended - If you ever change the name of this \"Error\" message, you'll need to update the name in the Check Loop Error.vi as well."
        # "#CodeRecommended - Consider creating a system for logging errors in some way. These errors are for notification purposes only. Handling of specific errors should be performed in the message frames that generated the error."
        # "Error - Display an error dialog. This message is sent by the \"Error Handler\" VIs at the end of other loops in this application."
        n1075 = Variant To Data(error in=w1929, type=errorcluster {"status"=FALSE, "code"=0, "source"=""} ("error constant"), Variant=w1927) -> (data=w1925:errorcluster, error out=w1924:errorcluster)
        n1076 = call <vilib>:"Simple Error Handler.vi"("error in (no error)"=w1925) -> ()  [unwired: 4 in, 5 out]
        n1077 = Merge Errors(w1924) -> (w1923:errorcluster)
      }
      frame "Confirm Quit" {
        # "#CodeNeeded - If you want to provide an \"Are you sure\" dialog (or some other notification) before the application exits, place that code here. This message is typically sent from a Panel Close? event."
        # "Confirm Quit - Message that can confirm whether or not the user wants to exit the application."
        n1078 = call-poly "Enqueue Message.vi"("Priority Message? (F)"=TRUE, "error in (no error)"=w1936, "Message"="Exit", "Message Queue"=w1932) -> ("error out"=w1933:errorcluster)  [unwired: 6 in, 1 out]
        n1079 = Merge Errors(w1933) -> (w1934:errorcluster)
      }
      frame "Exit" {
        # "Stop the VI"
        # "Release the message queue reference"
        # "#CodeNeeded - Add any required cleanup code here. Note that if 'Exit' was called as a result of an error, an error dialog will be displayed. Add any custom error handling for an 'Exit' condition here as well."
        # "Exit - Exit the application."
        n1080 = call "Fire User Event - Stop.vi"("User Event - Stop"=w1937) -> ("error out"=w1939:errorcluster)  [unwired: 10 in]
        n1081 = Release Queue(queue=w1944, error in (no error)=w1938) -> (error out=w1941:errorcluster)  [unwired: 1 in, 2 out]
        n1082 = Merge Errors(w1939, w1941) -> (w1940:errorcluster)
      }
      frame Default {
        # "'Default' case only runs if there is a message that isn't defined in any of the other cases.  Output a programming error."
        n1083 = xnode "Error Ring"("parameter 0"=w1945) -> ("error out"=w1946:errorcluster)
      }
    }
    n1084 = call "LAB-IQ Error Handler - Message Handling Loop.vi"("error in (no error)"=w1893, "Message Queue"=w1895) -> ("dup error in"=w1894:errorcluster)  [unwired: 8 in, 1 out]
  }
  n1085 = while {
    shift-right: [w1965] -> _
    shift-left: w9 -> [w1966]
    tunnel: [w1959] -> _
    tunnel: w4 -> [w1957]
    tunnel: w7 -> [w1956]
    tunnel: w8 -> [w1955]
    stop <- w1964 stop-if-true
    # "Report  Handling Loop"
    n1086 = call "Dequeue Message.vi"("error in (no error)"=w1956, "Message Queue"=w1957) -> ("error out"=w1963:errorcluster, "Message Data"=w1961:variant, "Message"=w1962:string, "dup Message Queue"=w1960:refnum<queue>)  [unwired: 6 in]
    n1087 = case "Message Cases" shown="\"init\"" w1962 {
      selector: w1962 -> [_ _ _ _ _ w2010]
      tunnel: w1960 -> [w1967 w1978 _ w1997 w2009 _]
      tunnel: w1963 -> [w1970 w1975 w1994 w2001 w2003 _]
      tunnel: [w1971 w1979 w1988 w1999 w2005 w2011] -> w1958
      tunnel: w1966 -> [w1969 w1977 w1993 w2000 w2008 w2012]
      tunnel: [w1969 w1977 w1993 w2000 w2008 w2012] -> w1965
      tunnel: [_ _ _ _ TRUE _] -> w1964
      tunnel: w1961 -> [_ _ w1992 _ _ _]
      tunnel: w1955 -> [_ _ _ _ w2002 _]
      frame "init" {
        # "Initialize - All initialization work should take place in this message, since other loops can potentially enqueue messages that execute immediately after this one."
        n1088 = call-poly "Enqueue Message.vi"("error in (no error)"=w1970, "Message"="Report Main", "Message Queue"=w1967) -> ("error out"=w1971:errorcluster)  [unwired: 7 in, 1 out]
      }
      frame "Report Main" {
        n1089 = Unbundle By Name(w1977) -> ("Main Home Screen.EXIT"=w1976:refnum<vi>)
        n1090 = property class="Bool (strict)"(reference=w1976) -> (reference out=w1973:refnum<vi>, error out=w1974:errorcluster, "Value"=w1972:bool)  [unwired: 1 in]
        n1091 = case shown="False" w1972 {
          tunnel: [w1982 w1986] -> w1979
          tunnel: w1978 -> [w1981 w1985]
          tunnel: w1975 -> [w1980 w1984]
          frame True {
            n1092 = call-poly "Enqueue Message.vi"("error in (no error)"=w1980, "Message"="Confirm Quit", "Message Queue"=w1981) -> ("error out"=w1982:errorcluster)  [unwired: 7 in, 1 out]
          }
          frame False {
            n1093 = call-poly "Enqueue Message.vi"("error in (no error)"=w1984, "Message"="Report Main", "Message Queue"=w1985) -> ("error out"=w1986:errorcluster)  [unwired: 7 in, 1 out]
          }
        }
        n1094 = Close Reference(reference=w1973, error in (no error)=w1974) -> ()  [unwired: 1 out]
      }
      frame "Error" {
        # "#CodeRecommended - If you ever change the name of this \"Error\" message, you'll need to update the name in the Check Loop Error.vi as well."
        # "#CodeRecommended - Consider creating a system for logging errors in some way. These errors are for notification purposes only. Handling of specific errors should be performed in the message frames that generated the error."
        # "Error - Display an error dialog. This message is sent by the \"Error Handler\" VIs at the end of other loops in this application."
        n1095 = Variant To Data(error in=w1994, type=errorcluster {"status"=FALSE, "code"=0, "source"=""} ("error constant"), Variant=w1992) -> (data=w1990:errorcluster, error out=w1989:errorcluster)
        n1096 = call <vilib>:"Simple Error Handler.vi"("error in (no error)"=w1990) -> ()  [unwired: 4 in, 5 out]
        n1097 = Merge Errors(w1989) -> (w1988:errorcluster)
      }
      frame "Confirm Quit" {
        # "#CodeNeeded - If you want to provide an \"Are you sure\" dialog (or some other notification) before the application exits, place that code here. This message is typically sent from a Panel Close? event."
        # "Confirm Quit - Message that can confirm whether or not the user wants to exit the application."
        n1098 = call-poly "Enqueue Message.vi"("Priority Message? (F)"=TRUE, "error in (no error)"=w2001, "Message"="Exit", "Message Queue"=w1997) -> ("error out"=w1998:errorcluster)  [unwired: 6 in, 1 out]
        n1099 = Merge Errors(w1998) -> (w1999:errorcluster)
      }
      frame "Exit" {
        # "Stop the VI"
        # "Release the message queue reference"
        # "#CodeNeeded - Add any required cleanup code here. Note that if 'Exit' was called as a result of an error, an error dialog will be displayed. Add any custom error handling for an 'Exit' condition here as well."
        # "Exit - Exit the application."
        n1100 = call "Fire User Event - Stop.vi"("User Event - Stop"=w2002) -> ("error out"=w2004:errorcluster)  [unwired: 10 in]
        n1101 = Release Queue(queue=w2009, error in (no error)=w2003) -> (error out=w2006:errorcluster)  [unwired: 1 in, 2 out]
        n1102 = Merge Errors(w2004, w2006) -> (w2005:errorcluster)
      }
      frame Default {
        # "'Default' case only runs if there is a message that isn't defined in any of the other cases.  Output a programming error."
        n1103 = xnode "Error Ring"("parameter 0"=w2010) -> ("error out"=w2011:errorcluster)
      }
    }
    n1104 = call "LAB-IQ Error Handler - Message Handling Loop.vi"("error in (no error)"=w1958, "Message Queue"=w1960) -> ("dup error in"=w1959:errorcluster)  [unwired: 8 in, 1 out]
  }
  n1105 = Unregister For Events(event registration refnum=w45, error in=w43) -> (error out=w46:errorcluster)
  n1106 = Merge Errors(w46, w49, w21, w18, w15, w14) -> (w47:errorcluster)
  n1107 = call "Destroy User Event - Stop.vi"("error in (no error)"=w47, "User Event - Stop"=w8) -> ("error out"=w44:errorcluster)  [unwired: 9 in]
  n1108 = disable-structure shown="RUN_TIME_ENGINE==True" {
    disable-tunnel: w44 -> [_ _]
    frame condition #0 (active) {
    }
    frame condition #1 {
      # "Call Quit LabVIEW if running as a built application."
      n1109 = Quit LabVIEW() -> ()  [unwired: 1 in]
    }
  }
